vi "UHR-Fleezers Control (host) - 9.5.vi"() -> ()   [LabVIEW 2009]
uses:
  <vilib>/Utility/miscctls.llb/LVPoint32TypeDef.ctl
  <vilib>/Utility/miscctls.llb/LVMinMaxIncTypeDef.ctl
  <vilib>/userDefined/High Color/nirio_resource_hc.ctl
  <vilib>/Instr/_visa.llb/VISA Configure Serial Port (Instr).vi
  <vilib>/Platform/TimedLoop/XDataNode/XDataNode.xnode
  <vilib>/Platform/TimedLoop/XDataNode/loadlvalarms.vi
  <vilib>/Platform/TimedLoop/XDataNode/timing_clust.ctl
  <vilib>/Platform/TimedLoop/XDataNode/nitl_modes.ctl
  <vilib>/Platform/TimedLoop/XDataNode/wakeup.ctl
  <vilib>/rvi/interface/nirviOpenFPGA/nirviOpenFPGA.xnode
  FPGA Bitfiles/UHR-Fleezers Instr~3C_FPGA Target_UHR-Fleezers Contr~A5.lvbitx
  UHR-Fleezers Control (fpga) - 9.4.vi
  <vilib>/FPGAPlugInAG/PCIe-7852R/nirviIntfOpen_PCIe-7852R.vi
  <vilib>/rvi/interface/nirviMethod/nirviMethod.xnode
  <vilib>/Utility/error.llb/Merge Errors.vi
  <vilib>/LabVIEW Targets/FPGA/Rio/nirio_HostInterface/nirio_Reset.vi
  <vilib>/LabVIEW Targets/FPGA/Rio/nirio_HostInterface/nirio_DMAStopAll.vi
  <vilib>/rvi/interface/common/niFpgaNodeNameForErrorReporting.ctl
  <vilib>/rvi/errors/niLvFpgaWhatHappensToTopLevelVI.ctl
  <vilib>/LabVIEW Targets/FPGA/Rio/nirio_HostInterface/nirio_DisableInterrupts.vi
  <vilib>/Utility/error.llb/Error Cluster From Error Code.vi
  <vilib>/rvi/errors/niLvFpgaAdjustHostInterfaceError.vi
  <vilib>/rvi/interface/nirviReadWriteControl/nirviReadWriteControl.xnode
  <vilib>/LabVIEW Targets/FPGA/Rio/nirio_HostInterface/nirio_WriteBig.vi
  <vilib>/LabVIEW Targets/FPGA/Rio/nirio_HostInterface/nirio_DMAConfigure.vi
  <vilib>/LabVIEW Targets/FPGA/Rio/nirio_HostInterface/nirio_DMAStop.vi
  <vilib>/RVI Host/nirviSupport.llb/nirviErrorClusterFromErrorCode.vi
  <vilib>/LabVIEW Targets/FPGA/Rio/nirio_HostInterface/nirio_EnableInterrupts.vi
  <vilib>/rvi/errors/niLvFpgaReportInternalErrorWithAdditionalInfo.vi
  <vilib>/express/express analysis/Spectral/XNode/ExpressSpectralMeasurementsBlockNode.xnode
  <vilib>/express/express analysis/Spectral/Block/exnSpectralBlock spectral measurements PSD poly.vi
  <vilib>/express/express analysis/Spectral/Block/exnSpectralBlock spectral measurements PSD WFM.vi
  <vilib>/Waveform/WDTOps.llb/WDT Append Waveforms DBL.vi
  <vilib>/LabVIEW Targets/FPGA/Rio/nirio_HostInterface/nirio_ReadBig.vi
  <vilib>/rvi/interface/nirviCloseFPGA/nirviCloseFPGA.xnode
  <vilib>/FPGAPlugInAG/PCIe-7852R/nirviIntfClose_PCIe-7852R.vi
  <vilib>/vision/Avi1.llb/AviRefnum.ctl
  <vilib>/Analysis/NI_AALBase.lvlib
  <vilib>/Platform/TimedLoop/XDataNode/XDNodeRunTimeDep.lvlib
  openfpgaref.8.6.ctl
  NiRioSrv.dll
  <vilib>/vision/NI_Vision_Development_Module.lvlib
panel:
  in  "Sample Channel Flow":bool
  in  "Pump 3 contents":string="Left: ADig beads" caption="contents"
  in  "Pump 1 contents":string="Right: DNA beads" caption="contents"
  in  "Scripts":T1(tab)=enum."Fluor. Triggering (Yanking)"
  in  "Cap 1 Samp Flow ON":bool=TRUE
  in  "Cap 2 Samp Flow ON":bool=TRUE
  in  "Got DNA bead":bool
  in  "Got ADig bead":bool
  in  "Cap 2 Flow ON":bool=TRUE
  in  "Cap 1 Flow ON":bool=TRUE
  in  "Cap 2 T ON":bool=TRUE
  in  "Move Cap. 2 (ADig Left)":bool
  in  "Move Cap. 1 (DNA Right)":bool
  in  "Offset @ (MHz)":dbl=13.0
  in  "Cal/Data Acq. Spot":bool
  in  "W/ Offset":bool=TRUE
  in  "Cal @ (MHz)":dbl=15.0
  in  "Dump Beads":bool
  in  "Lower Ch. Cap.":bool
  in  "Cap 1 T ON":bool=TRUE
  in  "Move to Delta 2 (MHz)":dbl=15.0
  in  "Attempt Limit":dbl=30.0 caption="Limit"
  out "Attempts":dbl
  in  "Wait Before Save (s)":u32=1
  in  "Fish for Tether":bool
  in  "Closest Delta (MHz)":dbl=10.45 step=0.25
  in  "Stop F (pN)":dbl=2.0
  in  "Then...":string(combo)="5"
  in  "Move to Delta 1 (MHz)":dbl=13.0
  in  "Tether Alarm?":bool=TRUE
  out "Tether":bool
  in  "TA Cancel Save?":bool
  in  "TA Green Off?":bool
  in  "Dip Trap Delta 1 (MHz)":dbl=15.0
  in  "Move Trap Before?":bool
  in  "Save Data After?":bool
  in  "Green ON After?":bool
  in  "Dip Trap Delta 2 (MHz)":dbl=15.0
  in  "Move Trap After?":bool
  in  "Duration (s)":dbl=1.0
  in  "Dip for Protein":bool
  in  "APD to Watch":bool
  out "Duration (s)":dbl
  in  "Action":string(combo)="Yank"
  in  "Fl. Triggered...":bool
  in  "Fl. Delta Thresh. (kHz)":dbl=0.6
  out "Waiting":bool
  out "Fl. High":bool
  in  "N pts to average":u16=6
  in  "Yank Delay (s)":dbl=3.5
  in  "Yank to Delta Array (MHz)":dbl[](array[numeric])=[16.3, 15.85, 14.85]
  in  "N Array El":u8=3 min=1 step=1
  in  "Random Choice":bool=TRUE
  in  "Force Yank":bool
  in  "Force Reset":bool
  in  "Y change (mm)":dbl
  in  "Profile":bool
  out "Current Position":cluster{dbl, dbl, dbl}
  out "Sigma/Mean 2":dbl caption="Sigma/Mean" format="%#_2g"
  out "Rate sigma (Hz) 2":dbl caption="Sigma (Hz)" format="%0.2f"
  out "APD 2 Rate (Hz)":dbl format="%#_3p"
  out "Primary Video Display":T2(plugin-control)
  out "Waveform Graph":dbl[](graph) caption="APD Line Scan"
  in  "Inject Pump 3":bool
  in  "Inject Pump 1":bool
  out "Messages":string
  in  "APD Ave N":dbl=10.0
  out "Int. Time (s)":dbl
  in  "Stop All":bool
  out "Sigma/Mean":dbl format="%#_2g"
  out "Rate sigma (Hz)":dbl caption="Sigma (Hz)" format="%0.2f"
  in  "Tab Control 6":T3(tab)=enum."Imaging"
  in  "APD 2 Offset":dbl
  in  "APD 1 Offset":dbl
  out "RMS (Ang)":dbl format="%_2g"
  in  "Bead Sep. Int. Time (s)":dbl=5.0 caption="Int. Time (s)"
  in  "Below (kHz)":dbl=0.5
  in  "Above (kHz)":dbl=2.0
  in  "Adjust Scale\nto Mean":bool
  in  "Rescale on Mean":bool
  in  "Offset (nm)":dbl
  out "Mean":dbl caption="Mean (pN)" format="%#_3g"
  out "Force":waveform(dbl)[](graph)
  out "APD Chart":waveform(dbl)[](graph)
  in  "Calibration":u16(ring)=2 items=["None", "Position", "Force"]
  out "T1 X":dbl caption="T1 X (pN)" format="%0.2f"
  out "T2 X":dbl caption="T2 X (pN)" format="%0.2f"
  out "Bead Separation":waveform(dbl)(graph)
  in  "Amplitude (nm)":dbl=1.0
  out "Bead Mean (nm)":dbl caption="Mean (nm)" format="%0.2f"
  out "Difference":dbl caption="Difference (pN)" format="%.2g"
  in  "Take Detection Laser\nImage":bool
  out "APD 2":T2(plugin-control) caption="APD 2 (Cy5)"
  in  "Flip Green Filter":bool
  in  "Set X Only":bool
  in  "Set Y Only":bool
  out "APD 1":T2(plugin-control) caption="APD 1 (Cy3)"
  out "Detection Laser Y":T2(plugin-control)
  out "Pointer Y (V)":dbl format="%_3g"
  out "Pointer X (V)":dbl format="%_3g"
  in  "Set Confocal Spot (X-Y)":bool
  out "Detection Laser X":T2(plugin-control)
  out "Saved APD":dbl[][](graph) caption="Most Recent Time Trace"
  out "Trap Delta Graph":dbl[](graph) caption="Most Recent Time Trace"
  out "Save APD Deriv":dbl[][](graph) caption="Most Recent Time Trace"
  out "Delta Fl. 1":dbl
  out "Delta Fl. 2":dbl
  out "All Signals":waveform(dbl)[](graph)
  in  "Signals to Plot":i32(listbox)
  out "Trap Disp. Freq. (Hz)":dbl caption="Freq. (Hz)" format="%#_6p"
  out "Display Period (s)":dbl caption="Period (s)" format="%#_6p"
  in  "Trap Disp. Downsample":dbl=20000.0 caption="Downsample"
  in  "APD Disp. Scale":dbl=0.1 caption="Scale (Divide,\nfor above plot only)"
  in  "APD Disp. Downsample":dbl=30.0 caption="Integrate" min=1.0 step=1.0
  out "APD Display Freq. (Hz)":dbl caption="Freq. (Hz)"
  out "APD Display Period (s)":dbl caption="Period (s)"
  out "FFT 1":cluster{"f0":dbl, "df":dbl, "magnitude":dbl[]}[](graph)
  out "FFT 2":cluster{"f0":dbl, "df":dbl, "magnitude":dbl[]}[](graph)
  in  "FFT 1 Choice 1":u16(ring) items=["T1 Y", "T1 X", "T1 Sum", "T2 Y", "T2 X", "T2 Sum", "T1 FB X", "T1 FB Sum", "T2 FB X", "T2 FB Sum", "PSD Y", "PSD X", "PSD Y Sum", "none"]
  in  "FFT 2 Choice 1":u16(ring)=13 items=["T1 Y", "T1 X", "T1 Sum", "T2 Y", "T2 X", "T2 Sum", "T1 FB X", "T1 FB Sum", "T2 FB X", "T2 FB Sum", "PSD Y", "PSD X", "PSD Y Sum", "none"]
  in  "FFT 1 Choice 2":u16(ring)=1 items=["T1 Y", "T1 X", "T1 Sum", "T2 Y", "T2 X", "T2 Sum", "T1 FB X", "T1 FB Sum", "T2 FB X", "T2 FB Sum", "PSD Y", "PSD X", "PSD Y Sum", "none"]
  in  "FFT 2 Choice 2":u16(ring)=13 items=["T1 Y", "T1 X", "T1 Sum", "T2 Y", "T2 X", "T2 Sum", "T1 FB X", "T1 FB Sum", "T2 FB X", "T2 FB Sum", "PSD Y", "PSD X", "PSD Y Sum", "none"]
  in  "Compute FFT":bool
  in  "Reset FFT":bool
  in  "# Spectra to Ave.":dbl=100.0
  out "Ave. Time (s)":dbl
  out "1 Channel":waveform(dbl)(graph)
  out "Slow mean":dbl format="%0.2f"
  in  "Slow mean N ave.":dbl=1.0 min=1.0 step=1.0
  out "Mean Intensity":dbl
  out "Sigma":dbl
  out "Sigma/Mean":dbl
  in  "Subtract mean":bool
  in  "High Res. Display":u16(ring) items=["T1 Y", "T1 X", "T1 Sum", "T2 Y", "T2 X", "T2 Sum", "T1 FB X", "T1 FB Sum", "T2 FB X", "T2 FB Sum", "PSD Y", "PSD X", "PSD Y Sum"]
  out "APD 1 Rate (Hz)":dbl format="%#_3p"
  in  "Tab Control":T4(tab)=enum."Configuration"
  out "Stage Moving":bool
  in  "Read Cal":bool
  in  "Confocal Linescan":bool
  in  "Speed (nm/s)":dbl=100.0
  in  "Furthest Withdraw (MHz)":dbl=15.0
  in  "Confocal Image":bool
  in  "Round T1 X":bool caption="Round"
  in  "T1 offset_x (mV)":dbl=-26.302542012392074 format="%#_2g"
  in  "T1 kappa_x (pN/nm)":dbl=0.22546432407642192 min=0.0 step=0.001 format="%#_2g"
  out "Time (s)":dbl
  out "Total Time (s)":dbl
  in  "Start Saving":bool
  in  "Cal sets to save":u32=50 min=1 step=1
  in  "Comment (data description)":string="testing confocal setup"
  out "Calibrating Trap...":bool
  in  "Trap 2 (ON/OFF)":bool
  in  "Trap 1 (ON/OFF)":bool
  in  "Save Calibration":bool
  in  "N sets to save":u32=200 caption="N Sets"
  in  "Save N Sets":bool
  out "Save file name":path
  in  "Save ave N":dbl=500.0 caption="Averaging Factor"
  out "Saving...":bool
  in  "Stop Saving":bool
  out "Progress":u16(slide) scale=0.0..100.0
  out "Manipulating Trap":bool
  out "Buffer Status":dbl(slide) scale=0.0..1.0
  out "Overflow (data lost)":bool
  in  "Reset":bool
  out "Data Rate (Hz)":dbl caption="Trap Data Rate (Hz)" format="%#_3p"
  out "Data Period (s)":dbl caption="Trap Data Period (s)" format="%#_6p"
  out "Save Data Rate (Hz)":dbl caption="Rate (Hz)" format="%#_6p"
  out "Save Data Period (s)":dbl caption="Period (s)" format="%#_6p"
  in  "T1 alpha_x (nm/V)":dbl=630.439304367558 step=10.0 format="%#_3g"
  in  "T2 alpha_x (nm/V)":dbl=704.7738222964198 step=10.0 format="%#_3g"
  in  "T2 kappa_x (pN/nm)":dbl=0.2030110880477556 min=0.0 step=0.001 format="%#_2g"
  in  "T2 offset_x (mV)":dbl=-26.67973517613748 format="%#_2g"
  in  "BD 1 Frequency 1 (MHz)":dbl=70.0000037011009 caption="T1 X (MHz)" min=60.0 max=90.0 step=1.0 format="%#_6p"
  in  "BD 1 Frequency 2 (MHz)":dbl=85.0 caption="T2 X (MHz)" min=60.0 max=90.0 step=1.0 format="%#_6p"
  in  "Green Laser ON/Interlacing":bool
  in  "Round T2 X":bool caption="Round"
  in  "AO1":dbl(slide)=6.408063513378007 caption="Confocal Y (V)" min=0.0 max=10.0 step=0.01 scale=0.0..10.0 scale format="%_1f"
  in  "AO2":dbl(slide)=2.4332770775475328 caption="Confocal X (V)" min=0.0 max=10.0 step=0.01 scale=0.0..10.0 scale format="%_1f"
  in  "Trap Raster Scan":bool
  out "Raster Scanning...":bool
  in  "Trap Delta (MHz)":dbl=14.999996298899106
  in  "Setpoints (V)":cluster{"Set 1":dbl, "Set 2":dbl}={"Set 1"=9.0, "Set 2"=9.0}
  in  "Index":dbl=1.0 caption="Save File Index" min=1.0 step=1.0
  in  "Position Label 5":string="upper flow spot (UvrD)" caption="5"
  in  "Move to Position":bool
  in  "Position":dbl=1.0 min=1.0 max=10.0 step=1.0
  in  "Set Position":bool
  in  "Saved Stage Positions":dbl[][](array[numeric])=[[1.0, 2.24438, -0.22402, 0.00732], [2.0, 0.0, 0.0, 0.0], [3.0, 2.75063, -0.30498, 0.00732], [4.0, 2.75063, -0.30498, 0.00732], [5.0, 2.75063, -2.32612, 0.00732], [6.0, 0.0, 0.0, 0.0], [7.0, 0.0, 0.0, 0.0], [8.0, 0.0, 0.0, 0.0], [9.0, 0.0, 0.0, 0.0], [10.0, 0.0, 0.0, 0.0]]
  in  "Move to Position 5":bool
  in  "z nudge increment (um)":dbl=0.5
  in  "+z":bool
  in  "Position 1 Label":string="Right capillary (DNA beads)" caption="1"
  in  "Set Position 1":bool
  in  "Set Position 2":bool
  in  "Set Position 3":bool
  in  "Set Position 4":bool
  in  "Move to Position 3":bool
  in  "Move to Position 4":bool
  in  "Move to Position 2":bool
  in  "Move to Position 1":bool
  in  "Position 2 Label":string="Left capillary (ADig beads)" caption="2"
  in  "Position 3 Label":string="lower flow spot (ATP)" caption="3"
  in  "Position 4 Label":string="Dump beads" caption="4"
  in  "-z":bool
  in  "Set Position 5":bool
  out "Stage Control Serial Error":errorcluster
  out "Pump 3 cont disp":string="Left: ADig beads"
  out "Pump 1 cont disp":string="Right: DNA beads "
  in  "Ch 1 Inject Rate (ul/h)":dbl=10.0
  in  "Pump write delay (ms)":dbl=300.0
  in  "All Pump Parameters":T5={"Pump 1"={"Diameter (mm)"=4.61, "Units"=3.0, "Volume"=0.0, "Rate"=0.0}, "Pump 2"={"Diameter (mm)"=4.61, "Units"=3.0, "Volume"=0.0, "Rate"=0.0}, "Pump 3"={"Diameter (mm)"=4.61, "Units"=3.0, "Volume"=0.0, "Rate"=0.0}}
  in  "Ch 2 Inject Volume (uL)":dbl=100.0
  in  "Pump pause delay (ms)":u32
  in  "Ch 3 Inject Volume (uL)":dbl=100.0
  in  "Ch 3 Inject Rate (ul/h)":dbl=10.0
  in  "Flush Center Ch Volume (uL)":dbl=15.0
  in  "Flush Center Ch Rate (ul/m)":dbl=100.0
  in  "Inject Pump 2":bool caption="Inject Pump 2\n(Flush Center)"
  in  "Total Volume\nFlushed (uL)":dbl
  in  "Tab Control 2":T6(tab)=enum."AOD Raster Scan"
  out "Total Counts (ticks)":u32
  in  "Trap ON/OFF X or Y Amp?":bool=TRUE
  in  "Oscillate Set 1":bool
  in  "Trap 1 ON":bool
  in  "Number Interlace Sets":u8=3 min=1 max=3
  in  "DIO count 3 (ticks)":u32=200
  in  "DIO count 2 (ticks)":u32=200
  in  "DIO count 1 (ticks)":u32=200
  in  "BD 2 Amplitude 3 (%)":dbl min=0.0 max=50.0 step=1.0
  in  "BD 2 Amplitude 2 (%)":dbl min=0.0 max=50.0 step=1.0
  in  "BD 2 Amplitude 1 (%)":dbl min=0.0 max=50.0 step=1.0
  in  "BD 1 Amplitude 3 (%)":dbl min=0.0 max=50.0 step=1.0
  in  "BD 1 Amplitude 2 (%)":dbl=35.0 min=0.0 max=50.0 step=1.0
  in  "BD 1 Amplitude 1 (%)":dbl=10.0 min=0.0 max=50.0 step=1.0
  in  "BD 2 Frequency 3 (MHz)":dbl=26.0 min=0.0 max=40.0 step=1.0 format="%#_6p"
  in  "BD 1 Frequency 3 (MHz)":dbl=70.0 min=60.0 max=90.0 step=1.0 format="%#_6p"
  in  "BD 2 Frequency 2 (MHz)":dbl=26.0 min=0.0 max=40.0 step=1.0 format="%#_6p"
  in  "BD 2 Frequency 1 (MHz)":dbl=26.0 min=0.0 max=40.0 step=1.0 format="%#_6p"
  in  "Not-Interlacing Set":enum32{"Set 1", "Set 2", "Set 3"}(radio)
  in  "Interlace":bool=TRUE
  in  "Trap 2 ON":bool
  in  "Trap 3 ON":bool
  in  "Scan axis 2":bool=TRUE
  in  "Osc. freq. (Hz)":dbl=0.25
  in  "Osc. amp. (MHz)":dbl=2.0
  out "Coords":T7
  in  "Manipulation Scaling":cluster{"Horizontal":dbl, "Vertical":dbl}={"Horizontal"=0.075, "Vertical"=0.01}
  in  "Freq or Amp switch first":bool=TRUE
  in  "Swap F1 and F2":bool
  in  "Freq switch delay":u16
  in  "Amp switch delay":u16=5
  in  "MCL Step Increment (V_int)":dbl=3.0
  out "Time to Finish All (min)":dbl format="%#_2p"
  in  "Scan Speed (nm/s)":dbl=100.0
  in  "Scan Range (nm)":dbl=500.0
  in  "Step Size (nm)":dbl=1.0
  in  "MCL/AOM Scale Tweak":dbl=1.0
  in  "MCL Step Position Ratio":dbl=0.5
  in  "Move MCL Also?":bool=TRUE
  out "Final sep (nm)":dbl
  out "Initial sep (nm)":dbl
  out "Save index":dbl
  out "Final delta (MHz)":dbl
  out "Initial delta (MHz)":dbl
  out "Final freq. (MHz)":dbl
  out "Initial freq. (MHz)":dbl
  in  "Saved AOD Raster Scan Parameter Sets":T8(array[cluster])=[{"Scan Range AOD (nm) 2"=500.0, "Step Size AOD (nm) 2"=1.0, "Scan Speed AOD (nm/s) 2"=200.0, "Number of scans (AOD) 2"=1, "Label"=""}, {"Scan Range AOD (nm) 2"=1000.0, "Step Size AOD (nm) 2"=1.0, "Scan Speed AOD (nm/s) 2"=200.0, "Number of scans (AOD) 2"=5, "Label"="wide offset scan"}, {"Scan Range AOD (nm) 2"=20.0, "Step Size AOD (nm) 2"=0.68, "Scan Speed AOD (nm/s) 2"=0.68, "Number of scans (AOD) 2"=1, "Label"="2 bp steps"}]
  in  "Load parameters":bool
  out "Scan Range (MHz)":dbl=10.0
  in  "Restart DMA? (AOD)":bool=TRUE caption="Restart DMA?"
  out "Incr. int (AOD)":i64
  out "Time/Scan (s) (AOD)":dbl format="%#_2p"
  out "Data points/scans":dbl
  out "Data points/scan (f/b)":dbl
  in  "Save scans":bool=TRUE
  out "AOD Scan I":u64 caption="Scan I"
  in  "Continuous AOD Scanning":bool caption="Continuous Scanning"
  in  "Abort AOD Scan":bool caption="Abort Scan"
  in  "Scan BD":bool=TRUE
  out "Cycles/step (AOD)":u64=400 format="%.0p"
  in  "Number of F/B Scans (AOD)":u16=1 min=1
  out "Scan steps (AOD)":u64=1000
  out "Scan Increment (MHz)":dbl=0.2
  out "AOD Scanning":bool caption="Scanning"
  in  "Start AOD Scan":bool caption="Start Scan"
  out "N sets should be saved":dbl
  out "Progress 2":u16(slide) caption="Progress" scale=0.0..100.0
  in  "Abort save 2":bool caption="Abort save"
  in  "Trap 1 Bead Size (nm)":dbl=860.0
  in  "Trap 2 Bead Size (nm)":dbl=790.0
  out "MCL Count":dbl
  in  "All FB On/Off":bool=TRUE
  in  "AI2 to Setpoint":cluster{"Set 1":bool, "Set 2":bool}
  out "AI2 (V)":cluster{"Set 1":dbl, "Set 2":dbl}
  in  "Reset Feedback":cluster{"Set 1":bool, "Set 2":bool}
  in  "PID Gains":T9={"Set 1"={"proportional gain (Kc)"=0, "integral gain (Kc*Ts/Ti)"=5, "derivative gain (Kc*Td/Ts)"=0}, "Set 2"={"proportional gain (Kc)"=0, "integral gain (Kc*Ts/Ti)"=5, "derivative gain (Kc*Td/Ts)"=0}}
  in  "Feedback On/Off":cluster{"Set 1":bool, "Set 2":bool}={"Set 1"=TRUE, "Set 2"=TRUE}
  in  "Tab Control 3":enum32{"Timing", "MCL Scan", "Analog Out"}(tab)
  out "APD 2 Gate Late Counter":u32
  out "APD 2 Gate Relative Phase":i16
  in  "Phase Adj. (APD 2 Gate)":i16=20
  in  "Initial Phase Adjustment (APD 2 Gate)":i16=55
  out "APD 1 Gate Late Counter":u32
  in  "- phase (APD 1 Gate)":bool
  in  "+ phase (APD 1 Gate)":bool
  out "APD 1 Gate Relative Phase":i16
  in  "Phase Adj. (APD 1 Gate)":i16=20
  in  "Initial Phase Adjustment (APD 1 Gate)":i16=60
  in  "Save APD Data\nwith Trap Data":bool=TRUE
  out "APD FIFO Elements Remaining":u32
  in  "- phase (APD Acq)":bool
  in  "+ phase (APD Acq)":bool
  out "APD Acq Late Counter":u32
  out "APD Acq Relative Phase":i16
  in  "Phase Adj. (APD Acq)":i16=20
  in  "Initial Phase Adjustment (APD Acq)":i16
  in  "Invert APD Gate":bool caption="Invert Gate"
  in  "APD Gate OFF Count":u32=450 caption="Gate OFF Count"
  in  "APD Gate ON Count":u32=150 caption="Gate ON Count"
  in  "APD Gate":enum32{"ON", "OFF", "Interlace"}(radio)=enum."Interlace"
  in  "APD Integration Time (s)":dbl=0.01 caption="Integration Time (s)"
  out "APD Acq Rate (Hz)":dbl=20000000.0 caption="Rate (Hz)"
  out "APD Samples/FIFO Acq.":dbl
  out "APD Elements/DMA read":u32
  out "APD Int. Count":u32 format="%.0p"
  in  "+ phase (APD 2 Gate)":bool
  in  "- phase (APD 2 Gate)":bool
  in  "Tab Control 5":enum32{"PSD X", "PSD Y", "Other Data Channel"}(tab)
  out "Data map":dbl[][](graph)
  in  "Channel":i32=4
  in  "Abort MCL Scan":bool
  out "MCL Scan I":u64
  out "MCL Scanning":bool
  in  "Start MCL Scan":bool
  out "wait to reset values":bool
  in  "Tab Control 4":enum32{"Scan Settings", "MCL FPGA Loop Timing"}(tab)
  out "Total Time (s)":dbl
  in  "Scan lines (y)":u64=20
  in  "Fast Scan Dir":bool=TRUE
  in  "2D or 1D Scan":bool=TRUE
  out "Initial X":dbl
  out "Initial Y":dbl
  out "Time/f+b scan (s) (MCL)":dbl caption="Time/scan (s)"
  in  "Number of scans (MCL)":u64=1 caption="Scans"
  in  "Scan steps (MCL)":u64=40 caption="Scan steps (x)"
  in  "N APD Samp/step":dbl=3.0
  in  "Scan Range (V)\n(of steps)":dbl=3.5
  in  "Restart DMA? (MCL)":bool=TRUE caption="Restart DMA?"
  in  "Continuous MCL Scanning":bool caption="Cont. Scanning"
  in  "Center Scan":bool=TRUE
  in  "Save Data (MCL)":bool=TRUE caption="Save Data"
  out "Actual Incr. int (MCL)":i16 caption="Incr. int"
  out "Desired incr (int)":dbl
  out "Desired Scan Incr (V)":dbl
  out "N sets should be saved (MCL)":dbl caption="N sets should be saved"
  out "Data points/scans (MCL)":dbl caption="Data points/scans"
  out "Data points/scan (f+b)":dbl caption="points/scan (f+b)"
  out "Cycles/step (MCL)":u64 caption="Cycles/step" format="%.0p"
  out "Actual MCL Inc (V)":dbl
  in  "Phase adjust (MCL)":i16 caption="Phase adjust"
  out "Relative Phase (MCL)":i16 caption="Relative Phase"
  in  "Initial Phase Adj. (MCL)":i16 caption="Initial Phase Adj."
  in  "Update Count (MCL)":u32=600
  in  "+ phase (MCL)":bool
  in  "- phase (MCL)":bool
  out "MCL Late Counter":u32
  in  "APD 1 AO Mult.":i16=1 min=1
  in  "APD 2 AO Mult.":i16=1 min=1
  in  "APD 1 AO offset":i16
  in  "APD 2 AO offset":i16
  in  "Tab Control 7":enum32{"Green FB Signals", "Slow MCL Scan"}(tab)
  out "Green FB Plot":dbl(graph)
  out "MCL Scan 2":cluster{"Begin (V)":dbl, dbl, dbl[]}(graph)
  out "MCL Scan":cluster{"Begin (V)":dbl, dbl, dbl[]}(graph)
  in  "Green laser mode":enum32{"Laser ON", "Laser OFF", "Interlace"}(radio)=enum."Interlace"
  in  "GI Frequency, ON count":u32=150 min=1 step=1
  in  "Invert GI":bool
  out "GI Late Counter":u32
  in  "Phase adj. (GI)":i16=5
  out "GI relative phase":i16
  in  "+ phase (GI)":bool
  in  "Initial Phase Adjustment (GI)":i16=19
  in  "GI Frequency, OFF count":u32=450 min=1 step=1
  in  "- phase (GI)":bool
  out "Green FB Signals (V)":cluster{"Y":dbl, "X":dbl, "Sum":dbl}
  out "Relative phase (Green FB)":i16
  in  "+ phase (Green FB)":bool
  in  "- phase (Green FB)":bool
  in  "Green FB Count":u32=600
  in  "Phase adj. (Green FB)":i16=10
  in  "Initial Phase Adjustment (Green FB)":i16=50
  in  "Green FB On/Off":bool=TRUE
  in  "Current When FB OFF (%)":dbl=87.0 min=0.0 max=100.0 step=1.0
  in  "Green int current ON count adj":u32=150
  in  "Green FB Gains":T10={"proportional gain (Kc)"=10, "integral gain (Kc*Ts/Ti)"=5, "derivative gain (Kc*Td/Ts)"=0}
  in  "Green FB Setpoint (mV)":dbl=100.0
  in  "- phase (GI) 2":bool
  in  "Initial Phase Adjustment (GI) 2":i16=-100
  in  "+ phase (GI) 2":bool
  out "GI relative phase 2":i16
  in  "Phase adj. (GI) 2":i16=20
  out "GI Late Counter 2":u32
  in  "# Samples/trap":dbl=20000.0 format="%#_6p"
  out "Elements/DMA read":u32 format="%.0p"
  out "Ave. Rate (Hz)":dbl format="%#_6p"
  out "FIFO El. Rem.":u32 format="%.0p"
  in  "Phase adj. (AI1)":i16=15
  out "Relative phase (AI1)":i16
  in  "+ phase (AI1)":bool
  in  "- phase (AI1)":bool
  out "Late Counter (AI1)":u32
  in  "Initial Phase Adjustment (AI1)":i16=220
  out "AI rate (Hz)":dbl=50000.0 format="%#_6p"
  in  "AI Count (ticks)":u32=200
  out "# Samples/channel":u32=20000 format="%.0p"
  in  "FIFO Depth":u32=600000 format="%.0p"
  in  "Detector Type":string(combo)="IR-QPD + PSD + FB-QPD X position"
  in  "N Acq Sets (Traps + Fl.)":i16=3
  in  "Sets to FIFO (Traps)":T11={"Set 1"=TRUE, "Set 2"=TRUE, "Set 3"=FALSE}
  in  "FPGA Ave.":dbl=1.0 min=1.0 step=1.0
  out "Ave. Period (s)":dbl format="%#_6p"
  out "DMA Update Period (s)":dbl
  out "FPGA Averaging":bool
  out "Trap Sets":i16
  out "Counts/DMA":dbl format="%#_6p"
  in  "Video Capture Rate (Hz)":dbl=30.0
  in  "Video Index":dbl=1.0 min=1.0 step=1.0
  in  "New Video File":bool
  in  "Save Video":bool
  in  "Reset Averaging":bool
  in  "Averaging":bool
  in  "Save Image":bool
  in  "Image Index":dbl=1.0 min=1.0
  out "Path Out":path
  in  "Center Point":cluster{"X":i32, "Y":i32}={"X"=335, "Y"=271}
  in  "Zoom Factor":sgl=7.0
  out "Window Size":cluster{"Width":i32, "Height":i32}
  out "Window Position":cluster{"X Position":i32, "Y Position":i32}={"X Position"=40, "Y Position"=40}
  in  "Initial Window Size":cluster{"Width":i32, "Height":i32}={"Width"=884, "Height"=619}
  in  "Initial Window Position":cluster{"X Position":i32, "Y Position":i32}={"X Position"=796, "Y Position"=4}
  in  "Intensity Upper":dbl=88.0
  in  "Intensity Lower":dbl=66.0
  out "error out":errorcluster
  out "error out 2":errorcluster
  in  "Harvard Syringe Pump Serial Port":refnum<visa-resource-name>="ASRL5::INSTR"
  in  "Lost Tether Alarm Threshold (pN)":dbl=0.5
  in  "AOM X Cal (nm/MHz)":dbl=123.0
  in  "MCL X Cal (nm/V)":dbl=1070.0
  out "X RF Amplitude Limits (%)":T12={"Minimum"=0.0, "Maximum"=50.0, "Increment"=1.0}
  out "X RF Frequency Limits (MHz)":T12={"Minimum"=60.0, "Maximum"=90.0, "Increment"=1.0}
  out "Y RF Frequency Limits (MHz)":T12={"Minimum"=60.0, "Maximum"=90.0, "Increment"=1.0}
  out "Y RF Amplitude Limits (%)":T12={"Minimum"=0.0, "Maximum"=50.0, "Increment"=1.0}
  in  "Manip. X?":bool=TRUE
  in  "Manip. Y?":bool
  in  "Force Manip Abort":bool
  out "Read cal error":errorcluster
  in  "DAQ Delay (ms)":u32=1000
  in  "Start Scan":bool
  in  "Scan axis":bool=TRUE
  in  "Osc. amp. (V)":dbl=5.0
  in  "Osc. center (V)":dbl=5.0
  in  "Osc. freq. (Hz) 2":dbl=1.0
  in  "MCL Mode":u16(ring) items=["Manual Positioning", "Sinusoidal Wave", "Linear Scan"]
  in  "Begin (V)":dbl
  in  "End (V)":dbl=10.0
  in  "N Points":dbl=20.0
  in  "Delay to Interlace (s)":dbl
  in  "Delayed Interlace Start":bool
  in  "Read Lateness and Rel Phase":bool
  out "Vec Mean of T1 T2":dbl[](array[numeric])
  in  "Cal read wait (s)":u32=5
  out "Time tether formed":timestamp
  in  "Sample Chamber Stage Serial Port":refnum<visa-resource-name>="ASRL4::INSTR"
  in  "Chemyx Syringe Pump Serial Port":refnum<visa-resource-name>="ASRL3::INSTR"
  in  "APD2 Trigger on Edge?":bool=TRUE
  in  "APD1 Trigger on Edge?":bool=TRUE
  in  "Limit Min (MHz)":dbl=10.0 caption="Min (MHz)"
  in  "Limit Max (MHz)":dbl=16.0 caption="Max (MHz)"
  in  "Limits Enable":bool=TRUE caption="Enable"
  # "After"
  # "During"
  # "Trap On?"
  # "BD Flow ON?"
  # "Samp Flow ON?"
  # "1"
  # "2"
  # "Trap Display:"
  # "APD Display:"
  # "DAQ"
  # "Trap Manipulation"
  # "Data Saving"
  # "Bead Calibration"
  # "Harvard Pump\n(sample channel for flow exp)"
  # "Chemyx Pump 2"
  # "Units: \n1 = ml/m\n2 = ml/h\n3 = ul/m\n4 = ul/h"
  # "Rate param is ul/h\nVolume param is ul"
  # "X"
  # "Y"
  # "Oscillate Set 1 freq. (debugging)"
  # "BD 1"
  # "BD 2"
  # "AOD Raster Scan"
  # "Approx. trap separations"
  # "X"
  # "Y"
  # "APD Gates"
  # "APD 2"
  # "APD 1"
  # "X"
  # "2D"
  # "Y"
  # "1D"
  # "Green Laser Interlacing"
  # "Green FB Measurement"
  # "Digital Gate"
  # "Current Analog Control"
  # "Total AI Rates (NOT rates/trap)"
  # "(Samples/trap x Trap Sets)"
  # "(Samples/channel x\n8 if averaging (8 channels)\n4 if no averaging)"
  # "Trap 1"
  # "Trap 2"
  # "Flour./Trap 3"
  # "External Video Window"
  # "MCL Position Debugging"
  # "Temporary Control Storage\n(these used to be somewhere else, still want to keep them)"
  # "Y"
  # "X"
  # "Trap Position Difference Limits"
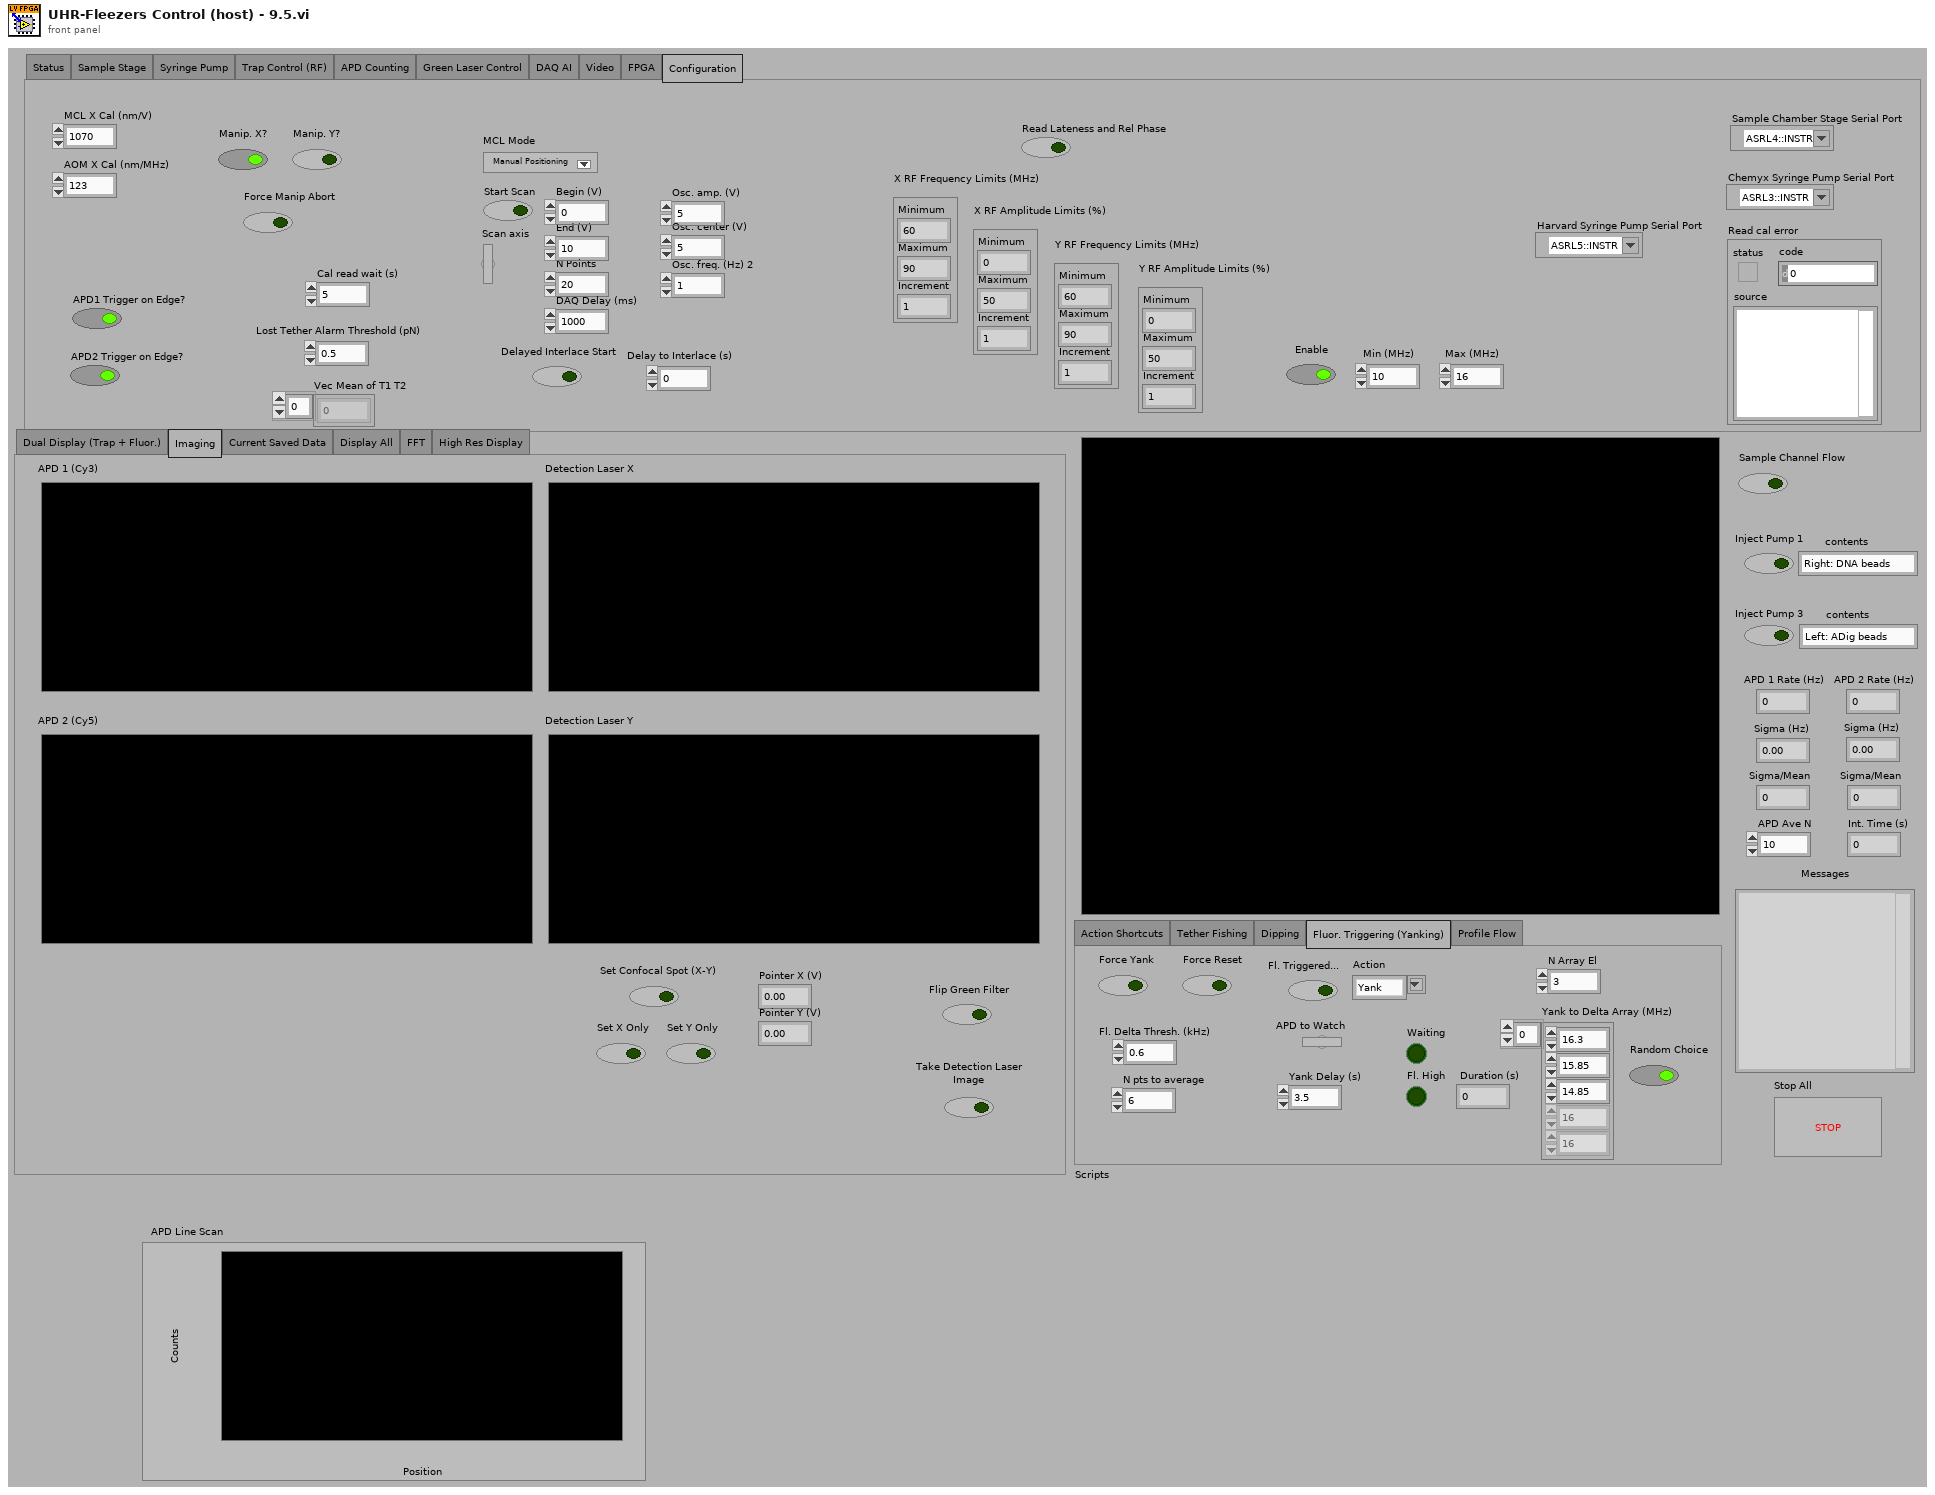
[diagram p1: front panel]
types:
  T1 = enum32{"Action Shortcuts", "Tether Fishing", "Dipping", "Fluor. Triggering (Yanking)", "Profile Flow"}
  T2 = typedef "IMAQ Image.ctl" = refnum<image>
  T3 = enum32{"Dual Display (Trap + Fluor.)", "Imaging", "Current Saved Data", "Display All", "FFT", "High Res Display"}
  T4 = enum32{"Status", "Sample Stage", "Syringe Pump", "Trap Control (RF)", "APD Counting", "Green Laser Control", "DAQ AI", "Video", "FPGA", "Configuration"}
  T5 = cluster{"Pump 1":cluster{"Diameter (mm)":dbl, "Units":dbl, "Volume":dbl, "Rate":dbl}, "Pump 2":cluster{"Diameter (mm)":dbl, "Units":dbl, "Volume":dbl, "Rate":dbl}, "Pump 3":cluster{"Diameter (mm)":dbl, "Units":dbl, "Volume":dbl, "Rate":dbl}}
  T6 = enum32{"IR Laser Interlacing (Direct RF Board Control Method)", "AOD Raster Scan", "Feedback on BD 1 Amp to Control AI2"}
  T7 = typedef "LVPoint32TypeDef.ctl" = cluster{"Horizontal":i32, "Vertical":i32}
  T8 = cluster{"Scan Range AOD (nm) 2":dbl, "Step Size AOD (nm) 2":dbl, "Scan Speed AOD (nm/s) 2":dbl, "Number of scans (AOD) 2":u16, "Label":string}[]
  T9 = cluster{"Set 1":cluster{"proportional gain (Kc)":i16, "integral gain (Kc*Ts/Ti)":i16, "derivative gain (Kc*Td/Ts)":i16}, "Set 2":cluster{"proportional gain (Kc)":i16, "integral gain (Kc*Ts/Ti)":i16, "derivative gain (Kc*Td/Ts)":i16}}
  T10 = cluster{"proportional gain (Kc)":i16, "integral gain (Kc*Ts/Ti)":i16, "derivative gain (Kc*Td/Ts)":i16}
  T11 = cluster{"Set 1":bool, "Set 2":bool, "Set 3":bool}
  T12 = typedef "LVMinMaxIncTypeDef.ctl" = cluster{"Minimum":dbl, "Maximum":dbl, "Increment":dbl}
  T13 = typedef "Image Type" = u32
  T14 = typedef "nirio_resource_hc.ctl" = tag
  T15 = typedef "openfpgaref.8.6.ctl" = refnum<k20>
  T16 = typedef "niFpgaNodeNameForErrorReporting.ctl" = enum16{"Open FPGA VI Reference", "Read/Write Control", "Invoke Method: Abort", "Invoke Method: Acknowledge IRQ", "Invoke Method: Download", "Invoke Method: FIFO.Configure", "Invoke Method: FIFO.Read", "Invoke Method: FIFO.Start", "Invoke Method: FIFO.Stop", "Invoke Method: FIFO.Write", "Invoke Method: Reset", "Invoke Method: Run", "Invoke Method: Wait on IRQ", "Close FPGA VI Reference"}
  T17 = typedef "niLvFpgaWhatHappensToTopLevelVI.ctl" = enum16{"top level VI scripted behind XNode", "top level VI inlined behind XNode"}
  T18 = cluster{"New Image":T2, "New Image":T2, "New Image":T2, "New Image":T2}
  T19 = typedef "XDNodeRunTimeDep.lvlib/timing_clust.ctl" = cluster{"Expected End [f-1]":u64, "Actual End [f-1]":u64, "Finished Late? [f-1]":bool, "Expected End [i-1]":u64, "Actual End [i-1]":u64, "Finished Late? [i-1]":bool, "Expected Start [i]":u64, "Actual Start [i]":u64, "Expected Start [f]":u64, "Actual Start [f]":u64, "Source Name":string, "Structure Name":string, "Period":i64, "Deadline":i64, "Offset":i64, "Start":i64, "Priority":i32, "Timeout":i32, "Mode":T20, "Wakeup Reason":T21, "Error":errorcluster, "Source Type":string, "Secondary Source Type":string, "Global End Time":u64, "Global Start Time":u64, "Frame Duration":u64, "Iteration Duration":u64, "Assigned CPU":i32, "I/O Scan Engine Mode":u32}
  T20 = typedef "XDNodeRunTimeDep.lvlib/nitl_modes.ctl" = enum32{"No Change", "Process missed periods, maintain original phase", "Discard missed periods, maintain original phase", "Process missed periods, ignore original phase", "Discard missed periods, ignore original phase"}
  T21 = typedef "XDNodeRunTimeDep.lvlib/wakeup.ctl" = enum32{"Normal", "Aborted", "Asynchronous wakeup", "Timing source error", "Timed loop error", "Timeout"}
  T22 = enum32{"Normal Display", "Dual Display (APD)", "FFT", "High Res Display"}
  T23 = cluster{"Origin Pixel":cluster{"X":sgl, "Y":sgl}, "Angle Relative to Horizontal (deg)":sgl, "Axis Reference":u32}
  T24 = typedef "Simple Grid Descriptor" = cluster{"X Step":sgl, "Y Step":sgl, "Unit":T25}
  T25 = typedef "Image Unit" = enum32{"Undefined", "Angström", "Micrometer", "Millimeter", "Centimeter", "Meter", "Kilometer", "Microinch", "Inch", "Feet", "Nautical miles", "Standard miles", "Steps"}
  T26 = cluster{"averaging mode":u16, "weighting mode":u16, "number of averages":u32}
  T27 = cluster{"dB On (F)":bool, "unwrap phase (F)":bool, "convert to degree (F)":bool}
  T28 = cluster{"Green FB Ch 0":i16, "Green FB Ch 1":i16, "Green FB Ch 2":i16}
  T29 = enum16{"open", "replace", "create", "open or create", "replace or create", "replace or create with confirmation"}
  T30 = enum16{"big-endian, network order", "native, host order", "little-endian"}
  T31 = cluster{string, string, string, string, string, string, string, string}
  T32 = cluster{string, string, string, string, string, string, string, string, string, string, string, string}
  T33 = cluster{string, string, string, string, string, string, string, string, string, string, string, string, string}
  T34 = cluster{string, string, string, string, string, string, string, string, string, string, string, string, string, string}
  T35 = cluster{"f0":dbl, "df":dbl, "magnitude":dbl[]}[][]
  T36 = cluster{"Green FB Ch 0":dbl, "Green FB Ch 1":dbl, "Green FB Ch 2":dbl}
  T37 = enum32{"setting", "request", "request control", "info", "statistics", "system settings", "I/O sub system", "HRT control", "camera descriptions", "device specific data", "event sub system settings", "event sub system results", "image memory manager"}
  T38 = typedef "AviRefnum.ctl" = refnum<k1>
  T39 = typedef "imagedata.ctl" = cluster{"image type":i32, "image depth":i32, "image":u8[], "mask":u8[], "colors":u32[], "Rectangle":cluster{"left":i16, "top":i16, "right":i16, "bottom":i16}}
  T40 = cluster{"Scan Range AOD (nm) 2":dbl, "Step Size AOD (nm) 2":dbl, "Scan Speed AOD (nm/s) 2":dbl, "Number of scans (AOD) 2":u16, "Label":string}
  T41 = cluster{"[0]":dbl, "[1]":dbl, "[2]":dbl, "[3]":dbl, "[4]":dbl, "[5]":dbl}
  T42 = cluster{"Diameter (mm)":dbl, "Units":dbl, "Volume":dbl, "Rate":dbl}
  T43 = cluster{"Left":i32, "Top":i32, "Width":u32, "Height":u32}
  T44 = cluster{cluster{"Left":i32, "Top":i32, "Width":u32, "Height":u32}}[]
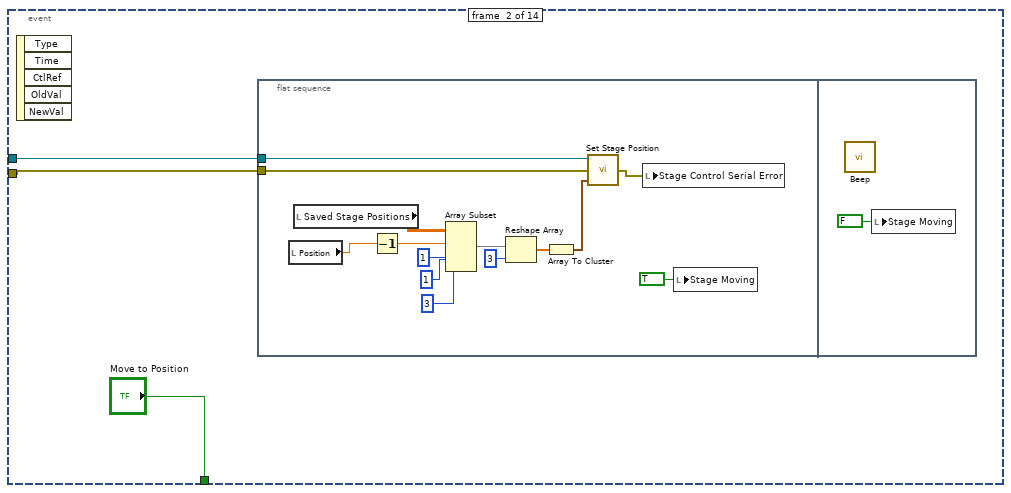
[diagram p2: hidden frame]
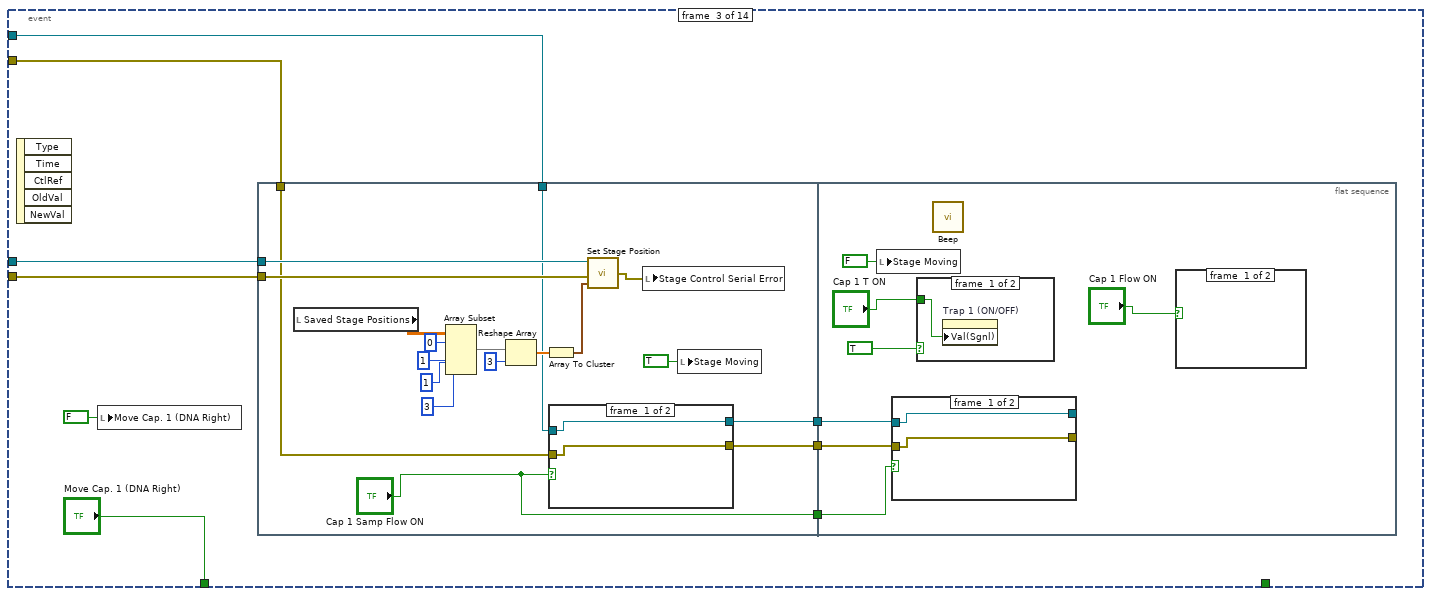
[diagram p3: hidden frame]
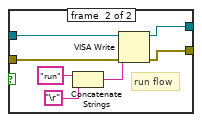
[diagram p4: hidden frame]
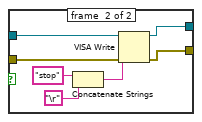
[diagram p5: hidden frame]
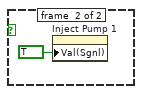
[diagram p6: hidden frame]
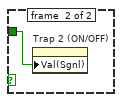
[diagram p7: hidden frame]
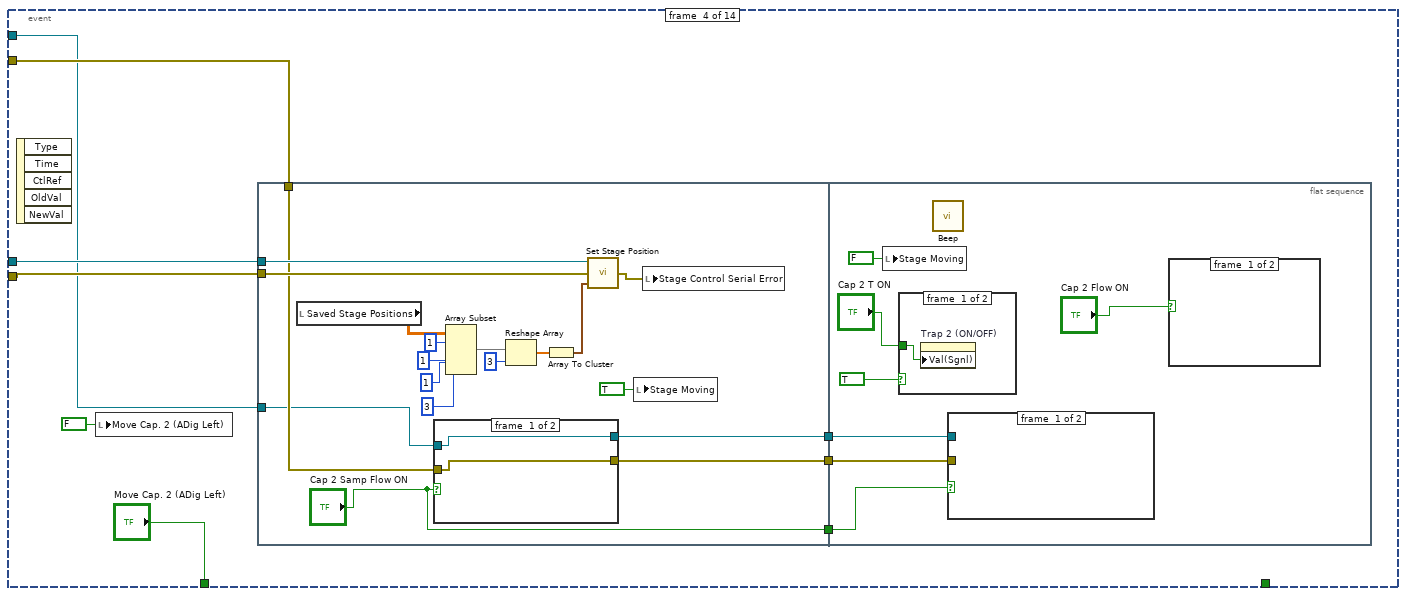
[diagram p8: hidden frame]
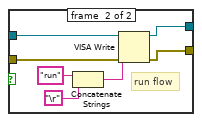
[diagram p9: hidden frame]
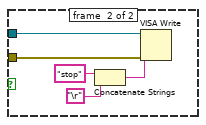
[diagram p10: hidden frame]
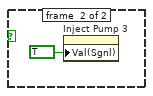
[diagram p11: hidden frame]
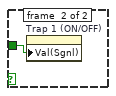
[diagram p12: hidden frame]
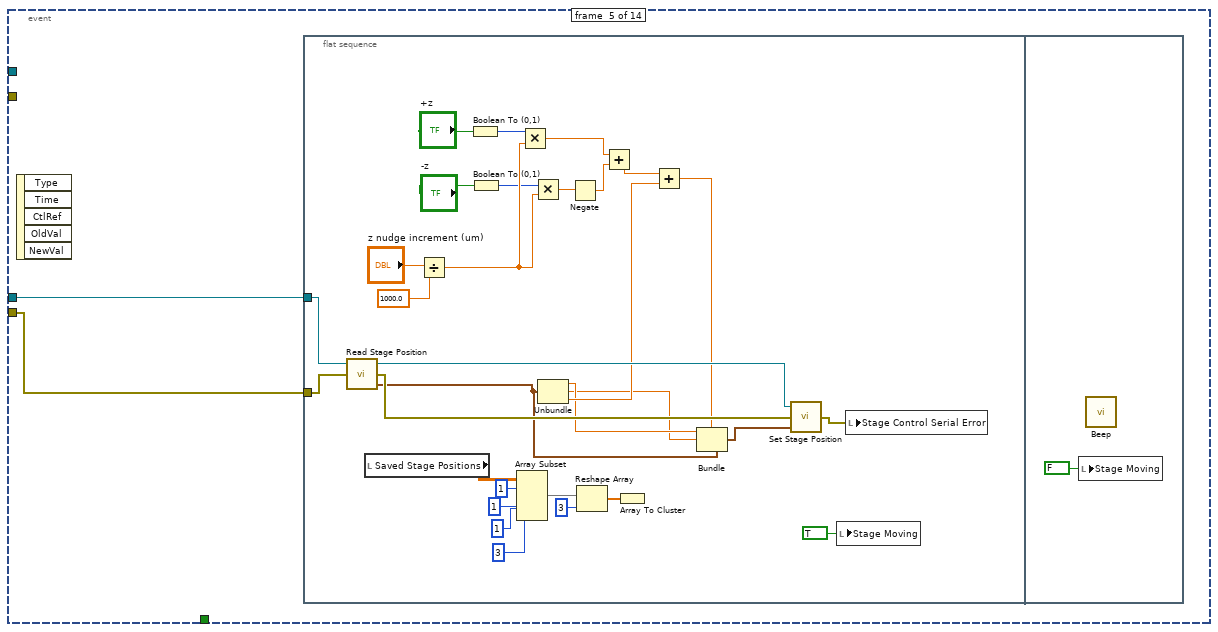
[diagram p13: hidden frame]
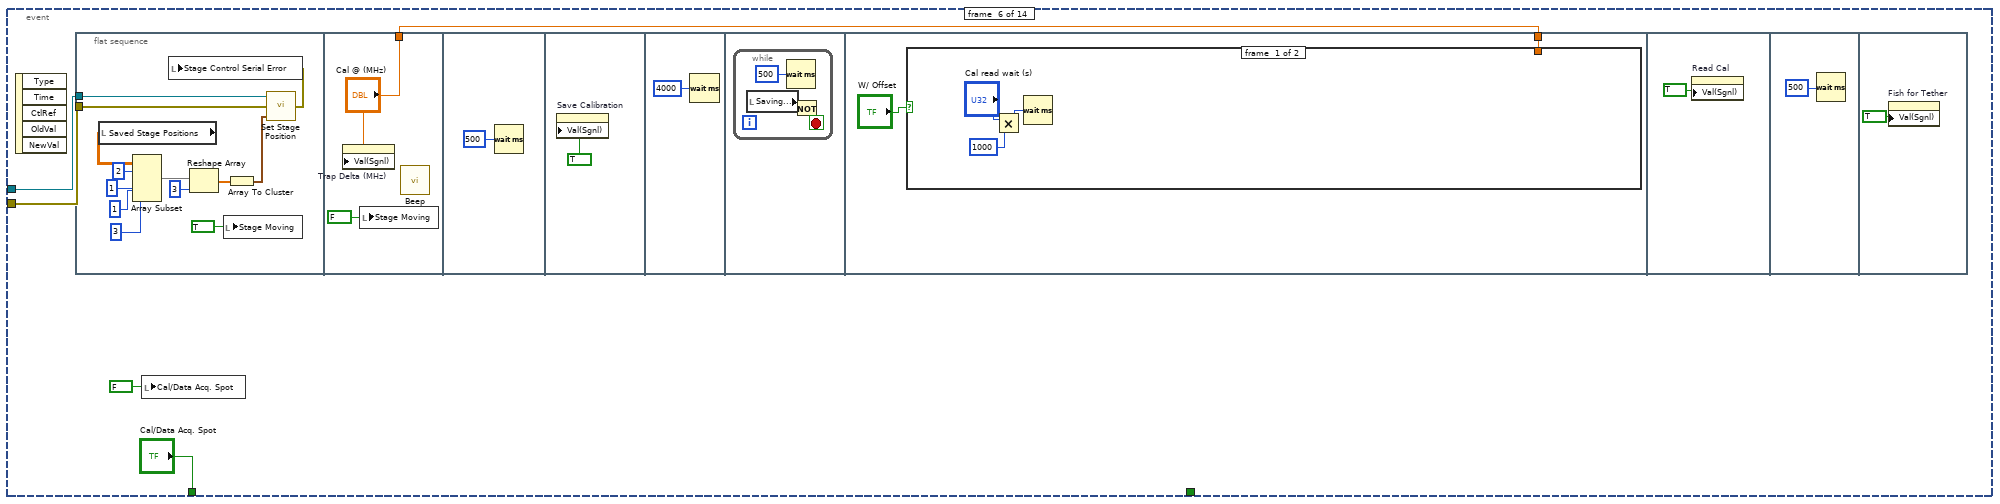
[diagram p14: hidden frame]
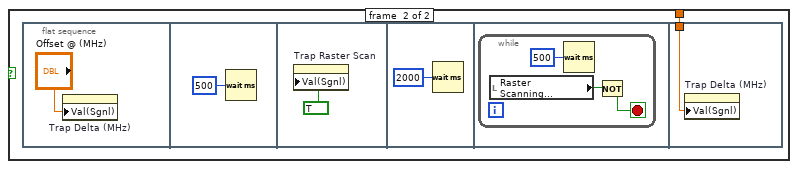
[diagram p15: hidden frame]
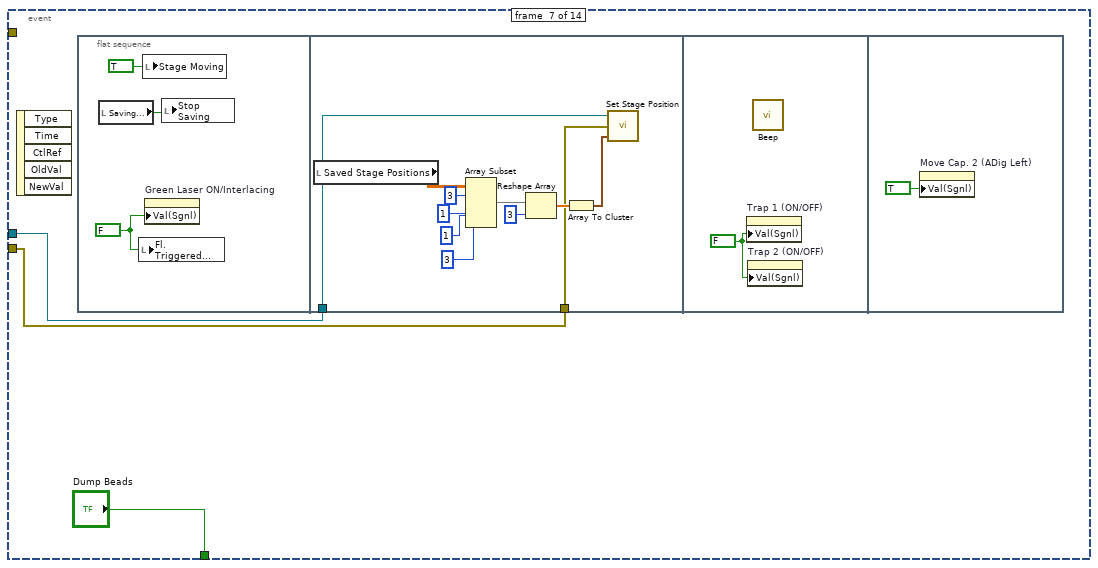
[diagram p16: hidden frame]
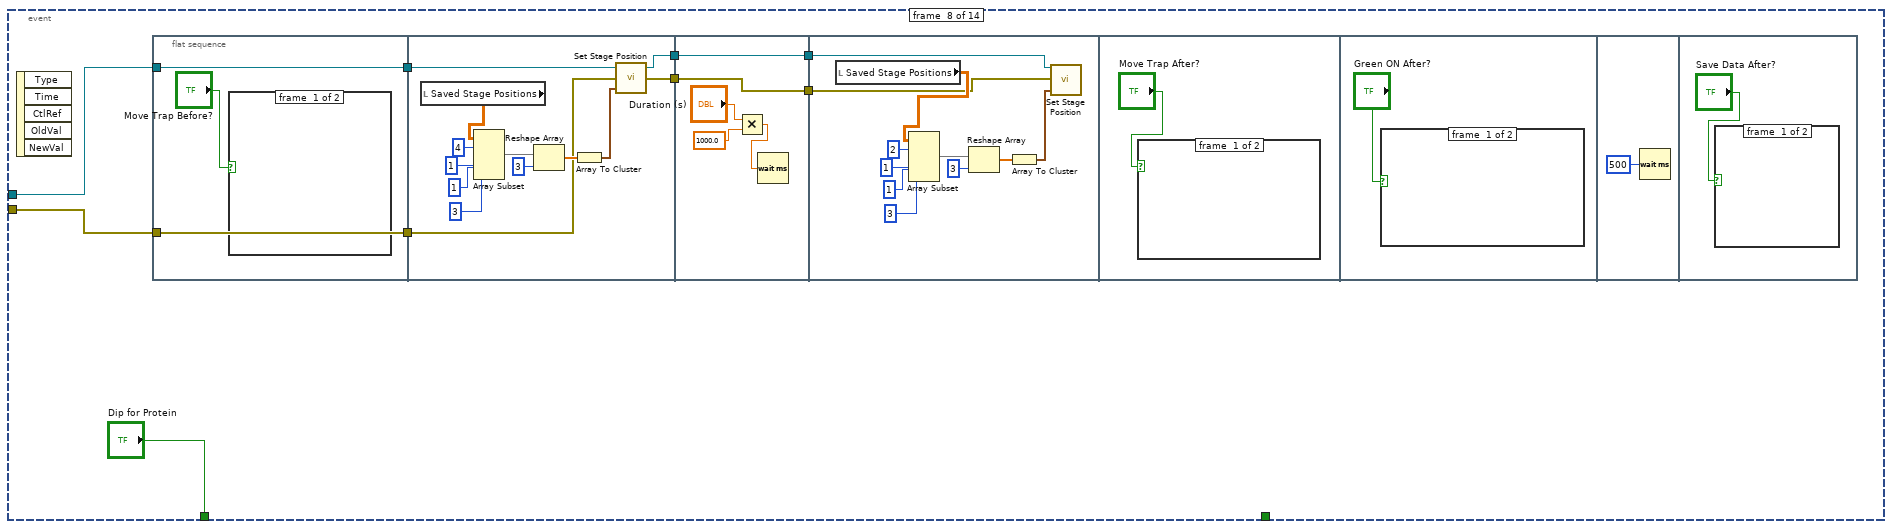
[diagram p17: hidden frame]
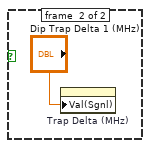
[diagram p18: hidden frame]
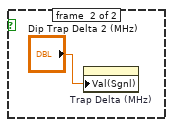
[diagram p19: hidden frame]
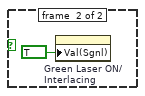
[diagram p20: hidden frame]
diagram:
  w4 = u16 20 items=["1.0"=10, "1.5"=15, "2.0"=20] ("stop bits (10: 1 bit)")
  w11 = T13 2 items=["Grayscale (U8)", "Grayscale (I16)", "Grayscale (SGL)", "Complex (CSG)", "RGB (U32)", "HSL (U32)", "RGB (U64)", "Grayscale (U16)"] ("Image Type")
  w81 = cluster{"output high":i16, "output low":i16} {"output high"=3000, "output low"=0} ("FB output range 1")
  w87 = TRUE ("AI to FIFO")
  w172 = 10.0 ("y")
  w171 = 32767.0 ("y")
  w187 = 6.0  # clock mult.
  w188 = 49152000.0  # TCXO frequ.
  n1 = Build Array("DIO count 1 (ticks)", "DIO count 2 (ticks)", "DIO count 3 (ticks)") -> (w68:u32[])
  n2 = Multiply(x="APD Integration Time (s)", y=40000000.0) -> (x*y=w95:dbl)
  n3 = Reciprocal(x="APD Integration Time (s)") -> (1/x=w92:dbl)
  n4 = local write "APD Acq Rate (Hz)"(w92) -> ()
  n5 = local read "AO1"() -> (w166:dbl)
  n6 = local read "AO2"() -> (w165:dbl)
  n7 = To Unsigned Long Integer(number=w95) -> (unsigned 32bit integer=w94:u32)
  "APD Int. Count" <- w94
  n8 = local read "Scan Increment (MHz)"() -> (w183:dbl)
  n9 = local read "Continuous MCL Scanning"() -> (w153:bool)
  n10 = local read "Fast Scan Dir"() -> (w152:bool)
  n11 = Multiply(x=w166, y=w171) -> (x*y=w168:dbl)
  n12 = local read "Number of scans (MCL)"() -> (w154:u64)
  n13 = Multiply(x=w165, y=w171) -> (x*y=w170:dbl)
  n14 = Divide(x=w168, y=w172) -> (x/y=w167:dbl)
  n15 = Divide(x=w170, y=w172) -> (x/y=w169:dbl)
  n16 = To Word Integer(number=w167) -> (16bit integer=w164:i16)
  n17 = To Word Integer(number=w169) -> (16bit integer=w163:i16)
  n18 = Not(x=w152) -> (.not. x?=w147:bool)
  n19 = local read "Cycles/step (MCL)"() -> (w155:u64)
  n20 = Multiply(x=w183, y=1000.0) -> (x*y=w190:dbl)
  n21 = local read "Scan steps (MCL)"() -> (w156:u64)
  n22 = local read "Desired Scan Incr (V)"() -> (w158:dbl)
  n23 = Scale By Power Of 2(n=48, x=w190) -> (x*2^n=w191:dbl)
  n24 = Multiply(x=w188, y=w187) -> (x*y=w186:dbl)
  n25 = Divide(x=w191, y=w186) -> (x/y=w185:dbl)
  n26 = local read "Setpoints (V)"() -> (w208:cluster{"Set 1":dbl, "Set 2":dbl})
  n27 = property on="AI Count (ticks)" class="DigNum (strict)"("Val(Sgnl)"="AI Count (ticks)") -> ()  [unwired: 2 in, 2 out]
  n28 = local read "Number Interlace Sets"() -> (w61:u8)
  n29 = Split 1D Array(array=w68, index=w61) -> (first subarray=w70:u32[])  [unwired: 1 out]
  n30 = Add Array Elements(numeric array=w70) -> (sum=w69:u32)
  n31 = local read "# Samples/channel"() -> (w175:u32)
  n32 = To Quad Integer(1:w185) -> (0:w182:i64)
  n33 = local read "Sets to FIFO (Traps)"() -> (w215:T11)
  n34 = local read "Number of F/B Scans (AOD)"() -> (w176:u16)
  n35 = local read "Not-Interlacing Set"() -> (w60:enum32{"Set 1", "Set 2", "Set 3"})
  n36 = To Unsigned Byte Integer(number=w60) -> (unsigned 8bit integer=w66:u8)
  n37 = Index Array(array=w68, index=w66) -> (element=w67:u32)
  n38 = Divide(x=40000000.0, y="AI Count (ticks)") -> (x/y=w143:dbl)
  n39 = Multiply(x=w158, y=32767.0) -> (x*y=w160:dbl)
  n40 = local read "Feedback On/Off"() -> (w211:cluster{"Set 1":bool, "Set 2":bool})
  n41 = local read "PID Gains"() -> (w203:T9)
  n42 = local read "Scan steps (AOD)"() -> (w181:u64)
  n43 = local read "All FB On/Off"() -> (w212:bool)
  n44 = local read "Cycles/step (AOD)"() -> (w180:u64)
  n45 = local write "AI rate (Hz)"(w143) -> ()
  n46 = Divide(x=w160, y=10.0) -> (x/y=w159:dbl)
  n47 = Multiply(x=w181, y=w180) -> (x*y=w179:u64)
  n48 = Multiply(x=3276.7, y=w208) -> (x*y=w207:cluster{"Set 1":dbl, "Set 2":dbl})
  n49 = To Word Integer(number=w159) -> (16bit integer=w157:i16)
  n50 = Multiply(x=w179, y=u64 2) -> (x*y=w177:u64)
  n51 = Divide(x=w143, y="FPGA Ave.") -> (x/y=w144:dbl)
  n52 = To Word Integer(number=w207) -> (16bit integer=w206:cluster{"Set 1":i16, "Set 2":i16})
  n53 = xnode "Open FPGA VI Reference"("resource name"=T14 "750kHzDAQ") -> ("FPGA VI Reference Out"=w198:T15, "error out"=w197:errorcluster)  [unwired: 1 in]
  n54 = Unbundle By Name(w203) -> ("Set 1"=w202:T10, "Set 2"=w201:T10)
  n55 = Multiply(x=w177, y=w176) -> (x*y=w174:u64)
  n56 = Divide(x=w174, y=w175) -> (x/y=w173:dbl)
  n57 = local write "Ave. Rate (Hz)"(w144) -> ()
  n58 = Unbundle By Name(w206) -> ("Set 1"=w205:i16, "Set 2"=w204:i16)
  n59 = local read "2D or 1D Scan"() -> (w84:bool)
  n60 = local write "Data points/scans"(w174) -> ()
  n61 = And(x=w211, y=w212) -> (x .and. y?=w210:cluster{"Set 1":bool, "Set 2":bool})
  n62 = local read "Scan BD"() -> (w192:bool)
  n63 = Reciprocal(x=w144) -> (1/x=w145:dbl)
  n64 = local write "Data points/scan (f/b)"(w177) -> ()
  n65 = local read "N Acq Sets (Traps + Fl.)"() -> (w136:i16)
  n66 = local write "N sets should be saved"(w173) -> ()
  n67 = Unbundle By Name(w210) -> ("Set 1"=w214:bool, "Set 2"=w213:bool)
  n68 = xnode "Invoke Method"("FPGA VI Reference In"=w198, "error in"=w197) -> ("FPGA VI Reference Out"=w80:T15, "error out"=w110:errorcluster)
  n69 = local read "Interlace"() -> (w62:bool)
  n70 = Select(t=w69, s=w62, f=w67) -> (s? t:f=w59:u32)
  n71 = local write "Update Count (MCL)"(w59) -> ()
  n72 = local write "Total Counts (ticks)"(w59) -> ()
  n73 = local write "Ave. Period (s)"(w145) -> ()
  n74 = property on="2D or 1D Scan" class="Bool (strict)"("Val(Sgnl)"=w84) -> ()  [unwired: 2 in, 2 out]
  n75 = xnode "Read/Write Control"("FPGA VI Reference In"=w79, "error in"=w110, "ai count"="AI Count (ticks)", "AI Averages"="FPGA Ave.", "DMA buffer timeout"=0, "AI to FIFO"=FALSE, "Interlace ON/OFF"=w62, "Number Interlace Cycles"=w61, "AI1 Sets to FIFO"=w215, "FB On/Off Set 1"=w214, "FB On/Off Set 2"=w213, "Interlace Off Parameters"=w60, "FB Setpoint Set 1"=w205, "FB Setpoint Set 2"=w204, "FB Gains Set 1"=w202, "FB Gains Set 2"=w201, "FB output range 1"=w81, "FB output range 2"=w81, "Cycles per step"=w180, "Scan BD"=w192, "Number of scans"=w176, "Scan steps"=w181, "Scan freq.  increment"=w182, "AO1"=w164, "AO2"=w163, "Scan freq.  increment (MCL)"=w157, "Scan steps (MCL)"=w156, "Cycles per step (MCL)"=w155, "Number of scans (MCL)"=w154, "MCL count"=w59, "Cont. Scan (MCL)"=w153, "MCL Scan Axis"=w147, "1D or 2D Scan?"=w84, "N of AI1 Int Acq Sets"=w136, "Freq or Amp switch first"="Freq or Amp switch first", "Freq switch delay"="Freq switch delay", "Amp switch delay"="Amp switch delay", "Swap F1 and F2"="Swap F1 and F2", "APD Acq Rate Count"=w94, "APD to FIFO"=FALSE, "APD Gate Operating Mode"="APD Gate", "APD Gate ON Count"="APD Gate ON Count", "APD Gate OFF Count"="APD Gate OFF Count", "Invert APD Gate"="Invert APD Gate", "DIO count 1 (ticks)"="DIO count 1 (ticks)", "DIO count 2 (ticks)"="DIO count 2 (ticks)", "DIO count 3 (ticks)"="DIO count 3 (ticks)", "APD 1 AO scale factor"="APD 1 AO Mult.", "APD 2 AO scale factor"="APD 2 AO Mult.", "APD 1 AO offset"="APD 1 AO offset", "APD 2 AO offset"="APD 2 AO offset") -> ("FPGA VI Reference Out"=w54:T15, "error out"=w56:errorcluster)
  n76 = local read "Green Laser ON/Interlacing"() -> (w57:bool)
  n77 = local read "GI Frequency, OFF count"() -> (w50:u32)
  n78 = local read "GI Frequency, ON count"() -> (w49:u32)
  n79 = Multiply(x="Current When FB OFF (%)", y=655.35) -> (x*y=w40:dbl)
  n80 = local read "Green laser mode"() -> (w58:enum32{"Laser ON", "Laser OFF", "Interlace"})
  n81 = local read "Green FB Count"() -> (w48:u32)
  n82 = To Unsigned Word Integer(number=w40) -> (unsigned 16bit integer=w38:u16)
  n83 = local read "Invert GI"() -> (w52:bool)
  n84 = Multiply(x="Green FB Setpoint (mV)", y=3.2767) -> (x*y=w37:dbl)
  n85 = case shown="False" w57 {
    tunnel: w58 -> [_ w242]
    tunnel: [enum32{"Laser ON", "Laser OFF", "Interlace"}."Laser OFF" ("Green laser mode") w242] -> w51
    frame #0 {
    }
    frame #1 {
    }
  }
  n86 = To Word Integer(number=w37) -> (16bit integer=w35:i16)
  n87 = xnode "Read/Write Control"("FPGA VI Reference In"=w54, "error in"=w56, "Green interlace ON count 2"=w49, "Green interlace OFF count 2"=w50, "Invert GI 2"=w52, "Operating Mode 2"=w51, "Green FB Gains"="Green FB Gains", "Green FB Setpoint"=w35, "Green FB On/Off"="Green FB On/Off", "Current Out"=w38, "Green int current ON count adj"="Green int current ON count adj", "Green FB Count"=w48, "Operating Mode"=w51, "Green interlace OFF count"=w50, "Green interlace ON count"=w49, "Invert GI"=w52, "APD2 Trigger on Edge?"="APD2 Trigger on Edge?", "APD1 Trigger on Edge?"="APD1 Trigger on Edge?") -> ("FPGA VI Reference Out"=w53:T15, "error out"=w55:errorcluster)
  n88 = flat-sequence {
    tunnel: w80 -> [w247]
    tunnel: [w247] -> w79
    tunnel: [w246] -> w78
    tunnel: [w245] -> w77
    tunnel: [w243] -> w75
    tunnel: [w244] -> w76
    frame #0 {
      w244 = T12 {"Minimum"=0.0, "Maximum"=40.0, "Increment"=1.0} ("Min Max Inc")
      w243 = T12 {"Minimum"=0.0, "Maximum"=50.0, "Increment"=1.0} ("Data Entry Limits")
      w246 = T12 {"Minimum"=60.0, "Maximum"=90.0, "Increment"=1.0} ("Min Max Inc")
      w245 = T12 {"Minimum"=0.0, "Maximum"=50.0, "Increment"=1.0} ("Data Entry Limits")
      n89 = property on="BD 2 Frequency 1 (MHz)" class="DigNum (strict)"("Data Range"=w244) -> ()  [unwired: 2 in, 2 out]
      n90 = property on="BD 2 Frequency 3 (MHz)" class="DigNum (strict)"("Data Range"=w244) -> ()  [unwired: 2 in, 2 out]
      n91 = property on="BD 2 Frequency 2 (MHz)" class="DigNum (strict)"("Data Range"=w244) -> ()  [unwired: 2 in, 2 out]
      n92 = property on="BD 1 Frequency 1 (MHz)" class="DigNum (strict)"("Data Range"=w246) -> ()  [unwired: 2 in, 2 out]
      n93 = property on="BD 1 Frequency 2 (MHz)" class="DigNum (strict)"("Data Range"=w246) -> ()  [unwired: 2 in, 2 out]
      n94 = property on="BD 1 Frequency 3 (MHz)" class="DigNum (strict)"("Data Range"=w246) -> ()  [unwired: 2 in, 2 out]
      n95 = property on="BD 2 Amplitude 1 (%)" class="DigNum (strict)"("Data Range"=w243) -> ()  [unwired: 2 in, 2 out]
      n96 = property on="BD 2 Amplitude 2 (%)" class="DigNum (strict)"("Data Range"=w243) -> ()  [unwired: 2 in, 2 out]
      n97 = property on="BD 2 Amplitude 3 (%)" class="DigNum (strict)"("Data Range"=w243) -> ()  [unwired: 2 in, 2 out]
      n98 = property on="BD 1 Amplitude 3 (%)" class="DigNum (strict)"("Data Range"=w245) -> ()  [unwired: 2 in, 2 out]
      n99 = property on="BD 1 Amplitude 2 (%)" class="DigNum (strict)"("Data Range"=w245) -> ()  [unwired: 2 in, 2 out]
      n100 = property on="BD 1 Amplitude 1 (%)" class="DigNum (strict)"("Data Range"=w245) -> ()  [unwired: 2 in, 2 out]
      "X RF Frequency Limits (MHz)" <- w246
      "X RF Amplitude Limits (%)" <- w245
      "Y RF Amplitude Limits (%)" <- w243
      "Y RF Frequency Limits (MHz)" <- w244
    }
  }
  n101 = xnode "Invoke Method"("FPGA VI Reference In"=w53, "error in"=w55, "Depth"="FIFO Depth") -> ("FPGA VI Reference Out"=w200:T15, "error out"=w199:errorcluster)
  n102 = xnode "Invoke Method"("FPGA VI Reference In"=w200, "error in"=w199) -> ("FPGA VI Reference Out"=w109:T15, "error out"=w108:errorcluster)
  n103 = xnode "Invoke Method"("FPGA VI Reference In"=w109, "error in"=w108) -> ("FPGA VI Reference Out"=w107:T15, "error out"=w106:errorcluster)  [unwired: 1 out]
  n104 = flat-sequence "Initial FPGA Loop Relative Phase Adjustment" {
    tunnel: "Initial Phase Adjustment (AI1)" -> [w258]
    tunnel: "Initial Phase Adjustment (GI)" -> [w257]
    tunnel: w107 -> [w256]
    tunnel: w106 -> [w255]
    tunnel: "Initial Phase Adj. (MCL)" -> [w254]
    tunnel: [w259] -> w118
    tunnel: [w253] -> w114
    tunnel: "Initial Phase Adjustment (APD Acq)" -> [w252]
    tunnel: "Initial Phase Adjustment (APD 1 Gate)" -> [w251]
    tunnel: "Initial Phase Adjustment (Green FB)" -> [w250]
    tunnel: "Initial Phase Adjustment (GI) 2" -> [w249]
    tunnel: "Initial Phase Adjustment (APD 2 Gate)" -> [w248]
    tunnel: w118 -> [w430]
    tunnel: [w431] -> w115
    tunnel: w114 -> [w431]
    tunnel: [w430] -> w113
    tunnel: w115 -> [w434]
    tunnel: w113 -> [w433]
    tunnel: [w436] -> w112
    tunnel: [w435] -> w111
    tunnel: [w615] -> w116
    tunnel: [w616] -> w117
    tunnel: w112 -> [w616]
    tunnel: w111 -> [w615]
    frame #0 {
      n105 = xnode "Read/Write Control"("FPGA VI Reference In"=w256, "error in"=w255, "Phase count adjustment"=w258, "Phase count adjustment (GI)"=w257, "Phase count adjustment (MCL)"=w254, "Phase Count Adjustment (APD Acq)"=w252, "Phase count adjustment (APD 1 Gate)"=w251, "Phase count adjustment (APD 2 Gate)"=w248, "Phase count adjustment (Green FB)"=w250, "Phase count adjustment (GI) 2"=w249) -> ("FPGA VI Reference Out"=w253:T15, "error out"=w259:errorcluster)
    }
    frame #1 {
      n106 = Wait (ms)(milliseconds to wait=u32 1000) -> ()  [unwired: 1 out]
    }
    frame #2 {
      w432 = TRUE
      n107 = xnode "Read/Write Control"("FPGA VI Reference In"=w434, "error in"=w433, "+ phase"=w432, "+ phase (GI)"=w432, "+ phase (MCL)"=w432, "+ phase (APD Acq)"=w432, "+ phase (APD 1 Gate)"=w432, "+ phase (APD 2 Gate)"=w432, "+ phase (Green FB)"=w432, "+ phase (GI) 2"=w432) -> ("FPGA VI Reference Out"=w435:T15, "error out"=w436:errorcluster)
    }
    frame #3 {
      n108 = Wait (ms)(milliseconds to wait=u32 1000) -> ()  [unwired: 1 out]
    }
  }
  n109 = local read "Phase adj. (Green FB)"() -> (w71:i16)
  n110 = local read "Phase adj. (GI) 2"() -> (w41:i16)
  n111 = local read "Phase adjust (MCL)"() -> (w148:i16)
  n112 = local read "Phase adj. (AI1)"() -> (w150:i16)
  n113 = local read "Phase adj. (GI)"() -> (w149:i16)
  n114 = xnode "Read/Write Control"("FPGA VI Reference In"=w116, "error in"=w117, "Phase count adjustment"=w150, "Phase count adjustment (GI)"=w149, "Phase count adjustment (MCL)"=w148, "Phase Count Adjustment (APD Acq)"="Phase Adj. (APD Acq)", "Phase count adjustment (APD 1 Gate)"="Phase Adj. (APD 1 Gate)", "Phase count adjustment (APD 2 Gate)"="Phase Adj. (APD 2 Gate)", "Phase count adjustment (Green FB)"=w71, "Phase count adjustment (GI) 2"=w41) -> ("FPGA VI Reference Out"=w27:T15, "error out"=w125:errorcluster)
  n115 = call "Initialize RF boards - interlace 3.vi"("error in"=w125, "FPGA VI Reference In"=w27) -> ("error out"=w123:errorcluster, "FPGA VI Reference Out"=w124:T15)
  n116 = call "set RF board frequency - interlace.vi"("Board 2 Frequency Limits"=w76, "Board 1 Frequency Limits"=w78, "error in"=w123, "FPGA VI Reference In"=w124, "Board 2 Frequency 3 (MHz)"="BD 2 Frequency 3 (MHz)", "Board 1 Frequency 3 (MHz)"="BD 1 Frequency 3 (MHz)", "Board 2 Frequency 2 (MHz)"="BD 2 Frequency 2 (MHz)", "Board 2 Frequency 1 (MHz)"="BD 2 Frequency 1 (MHz)", "Board 1 Frequency 2 (MHz)"="BD 1 Frequency 2 (MHz)", "Board 1 Frequency 1  (MHz)"="BD 1 Frequency 1 (MHz)") -> ("error out"=w231:errorcluster, "FPGA VI Reference Out"=w232:T15)
  n117 = call "set RF board amplitude - interlace.vi"("Board 2 Amplitude Limits"=w75, "Board 1 Amplitude Limits"=w77, "error in"=w231, "FPGA VI Reference In"=w232, "Board 2 Amplitude 3 (%)"="BD 2 Amplitude 3 (%)", "Board 1 Amplitude 3 (%)"="BD 1 Amplitude 3 (%)", "Board 2 Amplitude 2 (%)"="BD 2 Amplitude 2 (%)", "Board 2 Amplitude 1 (%)"="BD 2 Amplitude 1 (%)", "Board 1 Amplitude 2 (%)"="BD 1 Amplitude 2 (%)", "Board 1 Amplitude 1 (%)"="BD 1 Amplitude 1 (%)") -> ("error out"=w219:errorcluster, "FPGA VI Reference Out"=w220:T15)
  n118 = flat-sequence {
    tunnel: w220 -> [w625]
    tunnel: w219 -> [w624]
    tunnel: [w623] -> w224
    tunnel: [w622] -> w223
    tunnel: [w666] -> w222
    tunnel: w224 -> [w666]
    tunnel: [w665] -> w221
    tunnel: w223 -> [w665]
    tunnel: w222 -> [w674]
    tunnel: w221 -> [w673]
    tunnel: [w672] -> w89
    tunnel: [w671] -> w88
    frame #0 {
      n119 = local read "Trap 1 (ON/OFF)"() -> (w617:bool)
      n120 = xnode "Read/Write Control"("FPGA VI Reference In"=w625, "error in"=w624, "Direct RF Box  Communication"=FALSE) -> ("FPGA VI Reference Out"=w623:T15, "error out"=w622:errorcluster)
      n121 = local write "Saving..."(FALSE ("Saving Data")) -> ()
      n122 = local write "Stop All"(FALSE ("Stop All")) -> ()
      n123 = local write "Index"(1.0 ("Index")) -> ()
      n124 = property on="Trap 1 ON" class="Bool (strict)"("Value"=w617) -> ()  [unwired: 2 in, 2 out]
      "Manipulating Trap" <- FALSE ("Manipulating Trap")
    }
    frame #1 {
      n125 = local read "Trap 2 (ON/OFF)"() -> (w664:bool)
      n126 = Wait (ms)(milliseconds to wait=u32 10) -> ()  [unwired: 1 out]
      n127 = property on="Trap 2 ON" class="Bool (strict)"("Val(Sgnl)"=w664) -> ()  [unwired: 2 in, 2 out]
    }
    frame #2 {
      n128 = xnode "Read/Write Control"("FPGA VI Reference In"=w674, "error in"=w673, "FPGA Controls  RF Box"=TRUE ("Direct RF Box  Communication")) -> ("FPGA VI Reference Out"=w672:T15, "error out"=w671:errorcluster)
      n129 = call "Update messages.vi"("Message to add"="UHR-Fleezers ready.", "Old message string"="") -> ("New message string"=w670:string)
      n130 = local write "Messages"(w670) -> ()
    }
  }
  n131 = Subtract(x="BD 1 Frequency 1 (MHz)", y="BD 1 Frequency 2 (MHz)") -> (x-y=w135:dbl)
  n132 = Subtract(x="BD 2 Frequency 1 (MHz)", y="BD 2 Frequency 2 (MHz)") -> (x-y=w134:dbl)
  n133 = Square(x=w134) -> (x^2=w132:dbl)
  n134 = Square(x=w135) -> (x^2=w133:dbl)
  n135 = Add(x=w133, y=w132) -> (x+y=w131:dbl)
  n136 = Square Root(x=w131) -> (sqrt(x)=w130:dbl)
  n137 = local write "Trap Delta (MHz)"(w130) -> ()
  n138 = xnode "Read/Write Control"("FPGA VI Reference In"=w89, "error in"=w88, "AI to FIFO"=w87, "APD to FIFO"=w87) -> ("FPGA VI Reference Out"=w86:T15, "error out"=w85:errorcluster)
  n139 = call-poly "VISA Configure Serial Port"("VISA resource name"="Sample Chamber Stage Serial Port") -> ("VISA resource name out"=w22:refnum<visa-resource-name>, "error out"=w23:errorcluster)  [unwired: 5 in, 8 out]
  "Stage Control Serial Error" <- w23
  n140 = call "IMAQ Create"("Image Name"="APD 1 Image", "Image Type"=w11) -> ("New Image"=w10:T2)  [unwired: 3 in, 1 out]
  n141 = call "IMAQ Create"("Image Name"="APD 2 Image", "Image Type"=w11) -> ("New Image"=w9:T2)  [unwired: 3 in, 1 out]
  n142 = call "IMAQ Create"("Image Name"="Det. X Image", "Image Type"=w11) -> ("New Image"=w8:T2)  [unwired: 3 in, 1 out]
  n143 = call "IMAQ Create"("Image Name"="Det. Y Image", "Image Type"=w11) -> ("New Image"=w7:T2)  [unwired: 3 in, 1 out]
  n144 = call-poly "VISA Configure Serial Port"("VISA resource name"="Harvard Syringe Pump Serial Port", "baud rate (9600)"=u32 115200, "stop bits (10: 1 bit)"=w4) -> ("VISA resource name out"=w1:refnum<visa-resource-name>, "error out"=w2:errorcluster)  [unwired: 4 in, 7 out]
  n145 = Bundle("New Image"=w10, "New Image"=w9, "New Image"=w8, "New Image"=w7) -> (w6:T18)  [unwired: 1 in]
  n146 = node-c288(i64 1 ("Period")) -> (w139:T19)  [unwired: 3 out]
  n147 = node-c288() -> (w31:T19)  [unwired: 4 out]
  n148 = node-c288() -> (w29:T19)  [unwired: 4 out]
  n149 = node-c288() -> (w33:T19)  [unwired: 4 out]
  n150 = node-c288() -> (w18:T19)  [unwired: 4 in]
  n151 = timed-loop "Acquire Data" {
    tunnel: w86 -> [w904]
    tunnel: w85 -> [w903]
    tunnel: [w939] -> w239
    tunnel: [w933] -> w237
    timing: w139 -> [_]
    timing-out: [_] -> w138
    tunnel: w6 -> [w714]
    stop <- "Stop All" stop-if-true
    w790 = "NI_ChannelName" ("name")
    n152 = node-c288() -> ()  [unwired: 2 out]
    n153 = case "Reset data stream" shown="True" "Reset" {
      tunnel: w904 -> [w3205 w3212]
      tunnel: w903 -> [w3204 w3211]
      tunnel: [w3205 w3207] -> w899
      tunnel: [w3204 w3206] -> w898
      frame #0 {
      }
      frame #1 {
        w3210 = TRUE ("AI to FIFO")
        w3217 = FALSE ("AI to FIFO")
        n154 = local write "Overflow (data lost)"(FALSE ("Overflow (data lost)")) -> ()
        n155 = xnode "Read/Write Control"("FPGA VI Reference In"=w3212, "error in"=w3211, "AI to FIFO"=w3217, "APD to FIFO"=w3217) -> ("FPGA VI Reference Out"=w3215:T15, "error out"=w3216:errorcluster)
        n156 = xnode "Invoke Method"("FPGA VI Reference In"=w3215, "error in"=w3216) -> ("FPGA VI Reference Out"=w3213:T15, "error out"=w3214:errorcluster)
        n157 = xnode "Invoke Method"("FPGA VI Reference In"=w3213, "error in"=w3214) -> ("FPGA VI Reference Out"=w3209:T15, "error out"=w3208:errorcluster)
        n158 = xnode "Read/Write Control"("FPGA VI Reference In"=w3209, "error in"=w3208, "AI to FIFO"=w3210, "APD to FIFO"=w3210) -> ("FPGA VI Reference Out"=w3207:T15, "error out"=w3206:errorcluster)
      }
    }
    n159 = Or(x="Start AOD Scan", y="Trap Raster Scan") -> (x .or. y?=w849:bool)
    n160 = And(x="Save scans", y=w849) -> (x .and. y?=w895:bool)
    n161 = case "Start AOM raster scan" shown="True" w849 {
      tunnel: w899 -> [w2443 w2453]
      tunnel: w898 -> [w2442 w2452]
      tunnel: [w2443 w2446] -> w897
      tunnel: [w2442 w2445] -> w896
      frame #0 {
      }
      frame #1 {
        n162 = case shown="True" "Restart DMA? (AOD)" {
          tunnel: [w2819 w2820] -> w2447
          tunnel: [w2818 w2821] -> w2448
          tunnel: w2453 -> [w2819 w2827]
          tunnel: w2452 -> [w2818 w2826]
          frame #0 {
          }
          frame #1 {
            w2823 = FALSE ("AI to FIFO")
            n163 = xnode "Read/Write Control"("FPGA VI Reference In"=w2827, "error in"=w2826, "AI to FIFO"=w2823, "APD to FIFO"=w2823) -> ("FPGA VI Reference Out"=w2825:T15, "error out"=w2824:errorcluster)
            n164 = xnode "Invoke Method"("FPGA VI Reference In"=w2825, "error in"=w2824) -> ("FPGA VI Reference Out"=w2829:T15, "error out"=w2828:errorcluster)
            n165 = xnode "Invoke Method"("FPGA VI Reference In"=w2829, "error in"=w2828) -> ("FPGA VI Reference Out"=w2820:T15, "error out"=w2821:errorcluster)
            n166 = local write "Overflow (data lost)"(FALSE ("Overflow (data lost)")) -> ()
          }
        }
        n167 = case shown="True" "Move MCL Also?" {
          tunnel: w2448 -> [w2456 w2562]
          tunnel: w2447 -> [w2457 w2563]
          tunnel: [w2455 w2566] -> w2446
          tunnel: [w2454 w2565] -> w2445
          frame #0 {
            w2458 = TRUE ("AI to FIFO")
            n168 = xnode "Read/Write Control"("FPGA VI Reference In"=w2457, "error in"=w2456, "AI to FIFO"=w2458, "APD to FIFO"=w2458, "Start scan"=w2458) -> ("FPGA VI Reference Out"=w2455:T15, "error out"=w2454:errorcluster)
          }
          frame #1 {
            w2559 = FALSE ("1D or 2D Scan?")
            w2564 = TRUE ("AI to FIFO")
            # "Count for MCL loop"
            # "N total cycles"
            # "N steps"
            # "V_int"
            n169 = local read "Scan Range (nm)"() -> (w2541:dbl)
            n170 = local read "Number of F/B Scans (AOD)"() -> (w2558:u16)
            n171 = Sign(1:w2541) -> (0:w2540:dbl)
            n172 = Compound Arithmetic op=MULTIPLY(w2541, "MCL Step Position Ratio", "MCL/AOM Scale Tweak") -> (w2545:dbl)
            n173 = Negate(x=w2540) -> (-x=w2537:dbl)
            n174 = Multiply(x=w2537, y="MCL Step Increment (V_int)") -> (x*y=w2539:dbl)
            n175 = Divide(x=w2545, y="MCL X Cal (nm/V)") -> (x/y=w2551:dbl)
            n176 = Multiply(x=32767.0 ("y"), y=w2551) -> (x*y=w2557:dbl)
            n177 = local read "Total Counts (ticks)"() -> (w2542:u32)
            n178 = local read "Cycles/step (AOD)"() -> (w2553:u64)
            n179 = local read "Scan steps (AOD)"() -> (w2554:u64)
            n180 = Divide(x=w2557, y=10.0) -> (x/y=w2550:dbl)
            n181 = Divide(x=w2550, y="MCL Step Increment (V_int)") -> (x/y=w2548:dbl)
            n182 = Absolute Value(x=w2548) -> (abs(x)=w2536:dbl)
            n183 = Compound Arithmetic op=MULTIPLY(w2554, w2553, w2542) -> (w2549:u64)
            n184 = local write "wait to reset values"(w2564) -> ()
            n185 = local write "MCL Scanning"(w2564) -> ()
            n186 = Divide(x=w2549, y=w2536) -> (x/y=w2546:dbl)
            "MCL Count" <- w2546
            n187 = xnode "Read/Write Control"("FPGA VI Reference In"=w2563, "error in"=w2562, "Scan steps (MCL)"=w2536, "Number of scans (MCL)"=w2558, "Cycles per step (MCL)"=u64 1, "Scan freq.  increment (MCL)"=w2539, "1D or 2D Scan?"=w2559, "MCL Scan Axis"=w2559, "Cont. Scan (MCL)"=w2559, "MCL count"=w2546) -> ("FPGA VI Reference Out"=w2561:T15, "error out"=w2560:errorcluster)
            n188 = xnode "Read/Write Control"("FPGA VI Reference In"=w2561, "error in"=w2560, "AI to FIFO"=w2564, "APD to FIFO"=w2564, "Start scan"=w2564, "Start scan (MCL)"=w2564) -> ("FPGA VI Reference Out"=w2566:T15, "error out"=w2565:errorcluster)
          }
        }
        n189 = local write "Trap Raster Scan"(FALSE ("Trap Raster Scan")) -> ()
        "Raster Scanning..." <- TRUE ("Scanning...")
      }
    }
    n190 = Compound Arithmetic op=OR("Start MCL Scan", "Confocal Image", "Confocal Linescan") -> (w847:bool)
    n191 = And(x="Save Data (MCL)", y=w847) -> (x .and. y?=w894:bool)
    n192 = case "Start MCL raster scan" shown="True" w847 {
      tunnel: w897 -> [w1627 w1642]
      tunnel: w896 -> [w1626 w1641]
      tunnel: [w1627 w1637] -> w785
      tunnel: [w1626 w1636] -> w784
      tunnel: [FALSE w1635] -> w880
      tunnel: "Start MCL Scan" -> [_ w1630]
      tunnel: "Confocal Image" -> [_ w1629]
      tunnel: "Confocal Linescan" -> [_ _]
      frame #0 {
      }
      frame #1 {
        w1635 = TRUE
        n193 = case shown="True" "Restart DMA? (MCL)" {
          tunnel: [w1879 w1882] -> w1640
          tunnel: [w1878 w1881] -> w1639
          tunnel: w1642 -> [w1879 w1887]
          tunnel: w1641 -> [w1878 w1886]
          frame #0 {
          }
          frame #1 {
            w1883 = FALSE ("AI to FIFO")
            n194 = xnode "Read/Write Control"("FPGA VI Reference In"=w1887, "error in"=w1886, "AI to FIFO"=w1883, "APD to FIFO"=w1883) -> ("FPGA VI Reference Out"=w1885:T15, "error out"=w1884:errorcluster)
            n195 = xnode "Invoke Method"("FPGA VI Reference In"=w1885, "error in"=w1884) -> ("FPGA VI Reference Out"=w1889:T15, "error out"=w1888:errorcluster)
            n196 = xnode "Invoke Method"("FPGA VI Reference In"=w1889, "error in"=w1888) -> ("FPGA VI Reference Out"=w1882:T15, "error out"=w1881:errorcluster)
            n197 = local write "Overflow (data lost)"(FALSE ("Overflow (data lost)")) -> ()
          }
        }
        n198 = case shown="False" w1630 {
          selector: w1630 -> [_ w1646]
          tunnel: w1629 -> [w1645 _]
          tunnel: [w1645 w1646] -> w1628
          frame #0 {
            n199 = property on="2D or 1D Scan" class="Bool (strict)"("Val(Sgnl)"=w1645) -> ()  [unwired: 2 in, 2 out]
            n200 = property on="Confocal Image" class="Bool (strict)"("Value"=FALSE ("Start Confocal Map")) -> ()  [unwired: 2 in, 2 out]
          }
          frame #1 {
          }
        }
        n201 = local write "MCL Scanning"(w1635) -> ()
        n202 = local read "AO1"() -> (w1632:dbl)
        n203 = local read "AO2"() -> (w1631:dbl)
        n204 = case shown="True" "Center Scan" {
          tunnel: w1640 -> [w1653 w1762]
          tunnel: w1639 -> [w1652 w1761]
          tunnel: [w1651 w1760] -> w1637
          tunnel: [w1650 w1759] -> w1636
          tunnel: [w1648 w1746] -> w1634
          tunnel: [w1647 w1745] -> w1633
          tunnel: w1632 -> [w1648 w1751]
          tunnel: w1631 -> [w1647 w1754]
          tunnel: w1628 -> [_ _]
          frame #0 {
            w1649 = TRUE ("AI to FIFO")
            n205 = xnode "Read/Write Control"("FPGA VI Reference In"=w1653, "error in"=w1652, "AI to FIFO"=w1649, "APD to FIFO"=w1649, "Start scan (MCL)"=w1649) -> ("FPGA VI Reference Out"=w1651:T15, "error out"=w1650:errorcluster)
          }
          frame #1 {
            w1758 = TRUE ("AI to FIFO")
            n206 = local read "Scan steps (MCL)"() -> (w1737:u64)
            n207 = local read "Scan lines (y)"() -> (w1733:u64)
            n208 = local read "Fast Scan Dir"() -> (w1744:bool)
            n209 = local read "Actual MCL Inc (V)"() -> (w1734:dbl)
            n210 = Decrement(x=w1733) -> (x-1=w1732:u64)
            n211 = Decrement(x=w1737) -> (x-1=w1736:u64)
            n212 = Multiply(x=w1734, y=w1732) -> (x*y=w1731:dbl)
            n213 = Divide(x=w1731, y=2.0) -> (x/y=w1741:dbl)
            n214 = Multiply(x=w1734, y=w1736) -> (x*y=w1735:dbl)
            n215 = Divide(x=w1735, y=2.0) -> (x/y=w1740:dbl)
            n216 = Select(t=w1740, s=w1744, f=w1741) -> (s? t:f=w1739:dbl)
            n217 = Select(t=w1741, s=w1744, f=w1740) -> (s? t:f=w1743:dbl)
            n218 = Subtract(x=w1751, y=w1743) -> (x-y=w1742:dbl)
            n219 = Subtract(x=w1754, y=w1739) -> (x-y=w1738:dbl)
            n220 = local read "2D or 1D Scan"() -> (w1756:bool)
            n221 = Not(x=w1744) -> (.not. x?=w1750:bool)
            n222 = Not(x=w1756) -> (.not. x?=w1752:bool)
            n223 = And(x=w1744, y=w1752) -> (x .and. y?=w1753:bool)
            n224 = And(x=w1752, y=w1750) -> (x .and. y?=w1755:bool)
            n225 = Select(t=w1754, s=w1755, f=w1738) -> (s? t:f=w1745:dbl)
            n226 = Select(t=w1751, s=w1753, f=w1742) -> (s? t:f=w1746:dbl)
            n227 = call "Volt to I16.vi"("Voltage In"=w1746) -> ("I16 Voltage Out"=w1749:i16)
            n228 = call "Volt to I16.vi"("Voltage In"=w1745) -> ("I16 Voltage Out"=w1748:i16)
            n229 = xnode "Read/Write Control"("FPGA VI Reference In"=w1762, "error in"=w1761, "AI to FIFO"=w1758, "APD to FIFO"=w1758, "Start scan (MCL)"=w1758, "AO1"=w1749, "AO2"=w1748) -> ("FPGA VI Reference Out"=w1760:T15, "error out"=w1759:errorcluster)
          }
        }
        "Initial Y" <- w1634
        "Initial X" <- w1633
        "wait to reset values" <- w1635
      }
    }
    n230 = local read "APD Elements/DMA read"() -> (w753:u32)
    n231 = local read "Elements/DMA read"() -> (w808:u32)
    n232 = xnode "Get APD Data"("FPGA VI Reference In"=w785, "error in"=w784, "Number of Elements"=w753, "Timeout (ms)"=-1) -> ("Data"=w752:u32[], "Elements Remaining"=→"APD FIFO Elements Remaining":u32)  [unwired: 2 out]
    n233 = xnode "Get Trap Data"("FPGA VI Reference In"=w785, "error in"=w784, "Number of Elements"=w808, "Timeout (ms)"=-1 ("Timeout")) -> ("FPGA VI Reference Out"=w787:T15, "error out"=w786:errorcluster, "Data"=w918:u32[], "Elements Remaining"=w948:u32)
    "FIFO El. Rem." <- w948
    n234 = local read "FIFO Depth"() -> (w950:u32)
    n235 = Subtract(x=w950, y=w808) -> (x-y=w949:u32)
    n236 = Divide(x=w948, y=w949) -> (x/y=w947:dbl)
    "Buffer Status" <- w947
    n237 = Equal?(x=w947, y=1.0) -> (x = y?=w945:bool)
    n238 = case "Alert buffer overflow" shown="True" w945 {
      frame #0 {
      }
      frame #1 {
        n239 = call <vilib>:"Beep.vi"() -> ()  [unwired: 3 in, 9 out]
        "Overflow (data lost)" <- TRUE ("Overflow (data lost)")
      }
    }
    n240 = local read "FPGA Averaging"() -> (w807:bool)
    n241 = case "Special unpacking case if no averaging done by FPGA" shown="False" w807 {
      tunnel: w918 -> [w2039 w2065]
      tunnel: [w2010 w2040] -> w917
      frame #0 {
        n242 = Decimate 1D Array(w2039) -> (w2038:u32[], w2037:u32[], w2036:u32[], w2035:u32[])
        n243 = Split Number(x=w2038) -> (hi(x)=w2034:u16[], lo(x)=w2033:u16[])
        n244 = Split Number(x=w2037) -> (hi(x)=w2032:u16[], lo(x)=w2031:u16[])
        n245 = Split Number(x=w2036) -> (hi(x)=w2030:u16[], lo(x)=w2029:u16[])
        n246 = Split Number(x=w2035) -> (hi(x)=w2028:u16[], lo(x)=w2027:u16[])
        n247 = To Word Integer(number=w2034) -> (16bit integer=w2026:i16[])
        n248 = To Word Integer(number=w2033) -> (16bit integer=w2025:i16[])
        n249 = To Word Integer(number=w2032) -> (16bit integer=w2024:i16[])
        n250 = To Word Integer(number=w2031) -> (16bit integer=w2023:i16[])
        n251 = To Word Integer(number=w2030) -> (16bit integer=w2022:i16[])
        n252 = To Word Integer(number=w2029) -> (16bit integer=w2021:i16[])
        n253 = To Word Integer(number=w2028) -> (16bit integer=w2020:i16[])
        n254 = To Word Integer(number=w2027) -> (16bit integer=w2019:i16[])
        n255 = To Double Precision Float(number=w2026) -> (double precision float=w2018:dbl[])
        n256 = To Double Precision Float(number=w2025) -> (double precision float=w2017:dbl[])
        n257 = To Double Precision Float(number=w2024) -> (double precision float=w2016:dbl[])
        n258 = To Double Precision Float(number=w2023) -> (double precision float=w2015:dbl[])
        n259 = To Double Precision Float(number=w2022) -> (double precision float=w2014:dbl[])
        n260 = To Double Precision Float(number=w2021) -> (double precision float=w2013:dbl[])
        n261 = To Double Precision Float(number=w2020) -> (double precision float=w2012:dbl[])
        n262 = To Double Precision Float(number=w2019) -> (double precision float=w2011:dbl[])
        n263 = Interleave 1D Arrays(w2018, w2017, w2016, w2015, w2014, w2013, w2012, w2011) -> (w2010:dbl[])
      }
      frame #1 {
        n264 = Decimate 1D Array(w2065) -> (w2056:u32[], w2054:u32[], w2052:u32[], w2050:u32[], w2048:u32[], w2046:u32[], w2044:u32[], w2042:u32[])
        n265 = To Long Integer(number=w2056) -> (32bit integer=w2064:i32[])
        n266 = To Long Integer(number=w2054) -> (32bit integer=w2063:i32[])
        n267 = To Long Integer(number=w2052) -> (32bit integer=w2062:i32[])
        n268 = To Long Integer(number=w2050) -> (32bit integer=w2061:i32[])
        n269 = To Long Integer(number=w2048) -> (32bit integer=w2060:i32[])
        n270 = To Long Integer(number=w2046) -> (32bit integer=w2059:i32[])
        n271 = To Long Integer(number=w2044) -> (32bit integer=w2058:i32[])
        n272 = To Long Integer(number=w2042) -> (32bit integer=w2057:i32[])
        n273 = To Double Precision Float(number=w2064) -> (double precision float=w2055:dbl[])
        n274 = To Double Precision Float(number=w2063) -> (double precision float=w2053:dbl[])
        n275 = To Double Precision Float(number=w2062) -> (double precision float=w2051:dbl[])
        n276 = To Double Precision Float(number=w2061) -> (double precision float=w2049:dbl[])
        n277 = To Double Precision Float(number=w2060) -> (double precision float=w2047:dbl[])
        n278 = To Double Precision Float(number=w2059) -> (double precision float=w2045:dbl[])
        n279 = To Double Precision Float(number=w2058) -> (double precision float=w2043:dbl[])
        n280 = To Double Precision Float(number=w2057) -> (double precision float=w2041:dbl[])
        n281 = Interleave 1D Arrays(w2055, w2053, w2051, w2049, w2047, w2045, w2043, w2041) -> (w2040:dbl[])
      }
    }
    n282 = local read "FPGA Ave."() -> (w806:dbl)
    n283 = feedback #1(i16 -1 ("Trap Sets")) -> (w804:i16)
    n284 = feedback #2("" ("Detector Type")) -> (w801:string)
    n285 = Not Equal?(x=w801, y="Detector Type") -> (x != y?=w799:bool)
    n286 = local read "Trap Sets"() -> (w803:i16)
    n287 = Not Equal?(x=w804, y=w803) -> (x != y?=w798:bool)
    n288 = Or(x=w799, y=w798) -> (x .or. y?=w797:bool)
    n289 = Divide(x=w917, y=w806) -> (x/y=w925:dbl[])
    n290 = case "Deinterlace trap data, average down PSD" shown="2" w803 {
      tunnel: w925 -> [w2084 w2149]
      tunnel: [w2081 w2146] -> w791
      tunnel: [w2084 w2148] -> w924
      tunnel: "Detector Type" -> [w2083 w2144]
      tunnel: [w2082 w2147] -> w789
      tunnel: [w2080 w2145] -> w916
      frame #0 {
        n291 = Divide(x=w2084, y=3276.7) -> (x/y=w2085:dbl[])
        n292 = Decimate 1D Array(w2085) -> (w2094:dbl[], w2093:dbl[], w2092:dbl[], w2091:dbl[], w2090:dbl[], w2089:dbl[], w2088:dbl[], w2087:dbl[])
        n293 = case shown="\"IR-QPD + PSD + FB-QPD position\"" w2083 {
          tunnel: w2094 -> [w2118 w2143]
          tunnel: w2093 -> [w2117 w2142]
          tunnel: w2092 -> [w2102 w2120]
          tunnel: w2091 -> [w2103 w2130]
          tunnel: w2090 -> [w2116 w2141]
          tunnel: w2089 -> [w2115 w2140]
          tunnel: w2088 -> [w2099 w2121]
          tunnel: w2087 -> [w2098 w2119]
          tunnel: [w2097 w2127] -> w2082
          tunnel: [w2096 w2126] -> w2081
          tunnel: [w2095 w2125] -> w2080
          frame #0 {
            w2095 = 0  # Channel pattern
            n294 = Divide(x=w2118, y=w2103) -> (x/y=w2105:dbl[])
            n295 = Divide(x=w2117, y=w2103) -> (x/y=w2104:dbl[])
            n296 = Divide(x=w2116, y=w2099) -> (x/y=w2101:dbl[])
            n297 = Divide(x=w2115, y=w2098) -> (x/y=w2100:dbl[])
            n298 = Build Array(w2105, w2104, w2103, w2102, w2101, w2100, w2099, w2098) -> (w2096:dbl[][])
            n299 = Bundle("T1 Y", "T1 X", "T1 Sum", "FB Sum", "PSD Y", "PSD X", "PSD Y Sum", "PSD X Sum") -> (w2114:T31)  [unwired: 1 out]
            n300 = Cluster To Array(cluster=w2114) -> (array=w2097:string[])
          }
          frame #1 {
            w2125 = 3  # Channel pattern
            n301 = Negate(x=w2121) -> (-x=w2122:dbl[])
            n302 = Divide(x=w2143, y=w2130) -> (x/y=w2132:dbl[])
            n303 = Divide(x=w2142, y=w2130) -> (x/y=w2131:dbl[])
            n304 = Divide(x=w2141, y=w2121) -> (x/y=w2129:dbl[])
            n305 = Divide(x=w2140, y=w2122) -> (x/y=w2128:dbl[])
            n306 = Build Array(w2132, w2131, w2130, w2119, w2120, w2129, w2128, w2121) -> (w2126:dbl[][])
            n307 = Bundle("T1 Y", "T1 X", "T1 Sum", "FB X", "FB Sum", "PSD Y", "PSD X", "PSD Y Sum") -> (w2139:T31)  [unwired: 1 out]
            n308 = Cluster To Array(cluster=w2139) -> (array=w2127:string[])
          }
        }
      }
      frame #1 {
        n309 = case shown="\"IR-QPD + PSD + FB-QPD X position\"" w2144 {
          tunnel: w2149 -> [w2210 w2277 w2347]
          tunnel: [w2190 w2262 w2334] -> w2148
          tunnel: [w2176 w2253 w2325] -> w2147
          tunnel: [w2175 w2213 w2292] -> w2146
          tunnel: [w2169 w2251 w2323] -> w2145
          frame #0 {
            w2169 = 1  # Channel pattern
            # "time average x2 the 4th signal and the 4 psd signals (detection laser)"
            # "deinterlace 3 signals from qpd"
            n310 = Decimate 1D Array(w2210) -> (w2209:dbl[], w2208:dbl[], w2174:dbl[], w2207:dbl[], w2197:dbl[], w2195:dbl[], w2194:dbl[], w2192:dbl[])
            n311 = Decimate 1D Array(w2174) -> (w2173:dbl[], w2172:dbl[])
            n312 = Decimate 1D Array(w2209) -> (w2206:dbl[], w2178:dbl[])
            n313 = Decimate 1D Array(w2208) -> (w2205:dbl[], w2203:dbl[])
            n314 = Decimate 1D Array(w2207) -> (w2204:dbl[], w2202:dbl[])
            n315 = call "downsample 1D array - double.vi"("Ave N"=2.0, "Array In"=w2197) -> ("Array Out"=w2196:dbl[])  [unwired: 1 out]
            n316 = call "downsample 1D array - double.vi"("Ave N"=2.0, "Array In"=w2195) -> ("Array Out"=w2177:dbl[])  [unwired: 1 out]
            n317 = call "downsample 1D array - double.vi"("Ave N"=2.0, "Array In"=w2194) -> ("Array Out"=w2193:dbl[])  [unwired: 1 out]
            n318 = call "downsample 1D array - double.vi"("Ave N"=2.0, "Array In"=w2192) -> ("Array Out"=w2191:dbl[])  [unwired: 1 out]
            n319 = Interleave 1D Arrays(w2206, w2205, w2204, w2178, w2203, w2202, w2173, w2172, w2196, w2177, w2193, w2191) -> (w2190:dbl[])
            n320 = Divide(x=w2190, y=3276.7) -> (x/y=w2189:dbl[])
            n321 = Decimate 1D Array(w2189) -> (w2188:dbl[], w2187:dbl[], w2186:dbl[], w2185:dbl[], w2184:dbl[], w2183:dbl[], w2171:dbl[], w2170:dbl[], w2182:dbl[], w2181:dbl[], w2180:dbl[], w2179:dbl[])
            n322 = Divide(x=w2188, y=w2186) -> (x/y=w2156:dbl[])
            n323 = Divide(x=w2187, y=w2186) -> (x/y=w2155:dbl[])
            n324 = Divide(x=w2185, y=w2183) -> (x/y=w2154:dbl[])
            n325 = Divide(x=w2184, y=w2183) -> (x/y=w2153:dbl[])
            n326 = Divide(x=w2182, y=w2180) -> (x/y=w2152:dbl[])
            n327 = Divide(x=w2181, y=w2179) -> (x/y=w2151:dbl[])
            n328 = Build Array(w2156, w2155, w2186, w2154, w2153, w2183, w2171, w2170, w2152, w2151, w2180, w2179) -> (w2175:dbl[][])
            n329 = Bundle("T1 Y", "T1 X", "T1 Sum", "T2 Y", "T2 X", "T2 Sum", "T1 FB Sum", "T2 FB Sum", "PSD Y", "PSD X", "PSD Y Sum", "PSD X Sum") -> (w2157:T32)  [unwired: 1 out]
            n330 = Cluster To Array(cluster=w2157) -> (array=w2176:string[])
          }
          frame #1 {
            w2251 = 2  # Channel pattern
            # "time average x2 the 3 psd signals (detection laser)"
            # "deinterlace 3 signals from qpds"
            n331 = Decimate 1D Array(w2277) -> (w2276:dbl[], w2275:dbl[], w2252:dbl[], w2274:dbl[], w2265:dbl[], w2264:dbl[], w2263:dbl[], w2239:dbl[])
            n332 = Decimate 1D Array(w2252) -> (w2234:dbl[], w2232:dbl[])
            n333 = Decimate 1D Array(w2276) -> (w2273:dbl[], w2254:dbl[])
            n334 = Decimate 1D Array(w2275) -> (w2272:dbl[], w2270:dbl[])
            n335 = Decimate 1D Array(w2274) -> (w2271:dbl[], w2269:dbl[])
            n336 = Decimate 1D Array(w2239) -> (w2235:dbl[], w2233:dbl[])
            n337 = call "downsample 1D array - double.vi"("Ave N"=2.0, "Array In"=w2265) -> ("Array Out"=w2238:dbl[])  [unwired: 1 out]
            n338 = call "downsample 1D array - double.vi"("Ave N"=2.0, "Array In"=w2264) -> ("Array Out"=w2237:dbl[])  [unwired: 1 out]
            n339 = call "downsample 1D array - double.vi"("Ave N"=2.0, "Array In"=w2263) -> ("Array Out"=w2236:dbl[])  [unwired: 1 out]
            n340 = Interleave 1D Arrays(w2273, w2272, w2271, w2254, w2270, w2269, w2235, w2234, w2233, w2232, w2238, w2237, w2236) -> (w2262:dbl[])
            n341 = Divide(x=w2262, y=3276.7) -> (x/y=w2261:dbl[])
            n342 = Decimate 1D Array(w2261) -> (w2260:dbl[], w2259:dbl[], w2258:dbl[], w2257:dbl[], w2256:dbl[], w2255:dbl[], w2224:dbl[], w2222:dbl[], w2221:dbl[], w2219:dbl[], w2218:dbl[], w2217:dbl[], w2214:dbl[])
            n343 = Negate(x=w2214) -> (-x=w2212:dbl[])
            n344 = Divide(x=w2218, y=w2214) -> (x/y=w2216:dbl[])
            n345 = Divide(x=w2217, y=w2212) -> (x/y=w2215:dbl[])
            n346 = Divide(x=w2260, y=w2258) -> (x/y=w2243:dbl[])
            n347 = Divide(x=w2259, y=w2258) -> (x/y=w2242:dbl[])
            n348 = Divide(x=w2257, y=w2255) -> (x/y=w2241:dbl[])
            n349 = Divide(x=w2256, y=w2255) -> (x/y=w2240:dbl[])
            n350 = Divide(x=w2224, y=w2222) -> (x/y=w2223:dbl[])
            n351 = Divide(x=w2221, y=w2219) -> (x/y=w2220:dbl[])
            n352 = Build Array(w2243, w2242, w2258, w2241, w2240, w2255, w2223, w2222, w2220, w2219, w2216, w2215, w2214) -> (w2213:dbl[][])
            n353 = Bundle("T1 Y", "T1 X", "T1 Sum", "T2 Y", "T2 X", "T2 Sum", "T1 FB X", "T1 FB Sum", "T2 FB X", "T2 FB Sum", "PSD Y", "PSD X", "PSD Y Sum") -> (w2244:T33)  [unwired: 1 out]
            n354 = Cluster To Array(cluster=w2244) -> (array=w2253:string[])
          }
          frame #2 {
            w2323 = 4  # Channel pattern
            # "time average x2 the 3 psd signals (detection laser)"
            # "deinterlace 3 signals from qpds"
            n355 = Decimate 1D Array(w2347) -> (w2346:dbl[], w2345:dbl[], w2324:dbl[], w2344:dbl[], w2290:dbl[], w2336:dbl[], w2335:dbl[], w2312:dbl[])
            n356 = Decimate 1D Array "Feedback Sum"(w2324) -> (w2308:dbl[], w2306:dbl[])
            n357 = Decimate 1D Array "QPD Y"(w2346) -> (w2343:dbl[], w2326:dbl[])
            n358 = Decimate 1D Array "QPD X"(w2345) -> (w2342:dbl[], w2340:dbl[])
            n359 = Decimate 1D Array "Feedback Y"(w2290) -> (w2289:dbl[], w2288:dbl[])
            n360 = Decimate 1D Array "QPD Sum"(w2344) -> (w2341:dbl[], w2339:dbl[])
            n361 = Decimate 1D Array "Feedback X"(w2312) -> (w2309:dbl[], w2307:dbl[])
            n362 = call "downsample 1D array - double.vi"("Ave N"=2.0, "Array In"=w2336) -> ("Array Out"=w2311:dbl[])  [unwired: 1 out]
            n363 = call "downsample 1D array - double.vi"("Ave N"=2.0, "Array In"=w2335) -> ("Array Out"=w2310:dbl[])  [unwired: 1 out]
            n364 = Interleave 1D Arrays(w2343, w2342, w2341, w2326, w2340, w2339, w2289, w2309, w2308, w2288, w2307, w2306, w2311, w2310) -> (w2334:dbl[])
            n365 = Divide(x=w2334, y=3276.7) -> (x/y=w2333:dbl[])
            n366 = Decimate 1D Array(w2333) -> (w2332:dbl[], w2331:dbl[], w2330:dbl[], w2329:dbl[], w2328:dbl[], w2327:dbl[], w2285:dbl[], w2299:dbl[], w2283:dbl[], w2284:dbl[], w2297:dbl[], w2281:dbl[], w2295:dbl[], w2293:dbl[])
            n367 = Negate(x=w2293) -> (-x=w2291:dbl[])
            n368 = Divide(x=w2295, y=w2291) -> (x/y=w2294:dbl[])
            n369 = Divide(x=w2284, y=w2281) -> (x/y=w2280:dbl[])
            n370 = Divide(x=w2285, y=w2283) -> (x/y=w2282:dbl[])
            n371 = Divide(x=w2332, y=w2330) -> (x/y=w2316:dbl[])
            n372 = Divide(x=w2331, y=w2330) -> (x/y=w2315:dbl[])
            n373 = Divide(x=w2329, y=w2327) -> (x/y=w2314:dbl[])
            n374 = Divide(x=w2328, y=w2327) -> (x/y=w2313:dbl[])
            n375 = Divide(x=w2299, y=w2283) -> (x/y=w2298:dbl[])
            n376 = Divide(x=w2297, y=w2281) -> (x/y=w2296:dbl[])
            n377 = Build Array(w2316, w2315, w2330, w2314, w2313, w2327, w2282, w2298, w2283, w2280, w2296, w2281, w2294, w2293) -> (w2292:dbl[][])
            n378 = Bundle("T1 Y", "T1 X", "T1 Sum", "T2 Y", "T2 X", "T2 Sum", "T1 FB Y", "T1 FB X", "T1 FB Sum", "T2 FB Y", "T2 FB X", "T2 FB Sum", "PSD X", "PSD Y Sum") -> (w2279:T34)  [unwired: 1 out]
            n379 = Cluster To Array(cluster=w2279) -> (array=w2325:string[])
          }
        }
      }
    }
    n380 = case "Update these things only if detector type or number of traps changes" shown="True" w797 {
      tunnel: w789 -> [_ w1076]
      frame #0 {
      }
      frame #1 {
        n381 = property on="High Res. Display" class="Ring (strict)"("Strings []"=w1076) -> ()  [unwired: 2 in, 2 out]
        n382 = Build Array (concatenate)(w1076, "none") -> (w1069:string[])
        n383 = property on="FFT 1 Choice 1" class="Ring (strict)"("Strings []"=w1069) -> ()  [unwired: 2 in, 2 out]
        n384 = property on="FFT 1 Choice 2" class="Ring (strict)"("Strings []"=w1069) -> ()  [unwired: 2 in, 2 out]
        n385 = property on="FFT 2 Choice 1" class="Ring (strict)"("Strings []"=w1069) -> ()  [unwired: 2 in, 2 out]
        n386 = property on="FFT 2 Choice 2" class="Ring (strict)"("Strings []"=w1069) -> ()  [unwired: 2 in, 2 out]
        n387 = Bundle("APD 1", "APD 2") -> (w1072:cluster{string, string})  [unwired: 1 out]
        n388 = Cluster To Array(cluster=w1072) -> (array=w1070:string[])
        n389 = Build Array (concatenate)(w1070, w1069) -> (w1074:string[])
        n390 = Array Size(array=w1074) -> (size(s)=w1075:i32)
        n391 = property on="Signals to Plot" class="LstBox (strict)"("Item Names"=w1074) -> ()  [unwired: 2 in, 2 out]
        n392 = property on="Signals to Plot" class="LstBox (strict)"("Number of Rows"=w1075) -> ()  [unwired: 2 in, 2 out]
        n393 = property on="All Signals" class="WFChart (strict)"("LegNumRows"=w1075) -> ()  [unwired: 2 in, 2 out]
      }
    }
    n394 = local read "Data points/scans (MCL)"() -> (w889:dbl)
    n395 = Increment(x=w889) -> (x+1=w890:dbl)
    n396 = feedback #3(w890) -> (w893:dbl)
    n397 = Select(t=0, s=w880, f=w893) -> (s? t:f=w886:dbl)
    n398 = To Word Integer(number=w924) -> (16bit integer=w951:i16[])
    n399 = Decimate 1D Array(w752) -> (w783:u32[], w716:u32[])
    n400 = To Double Precision Float(number=w783) -> (double precision float=w782:dbl[])
    n401 = Array Size(array=w782) -> (size(s)=w892:i32)
    n402 = Add(x=w892, y=w886) -> (x+y=w887:dbl)
    n403 = Greater?(x=w887, y=w889) -> (0:w888:bool)
    n404 = local read "DMA Update Period (s)"() -> (w809:dbl)
    n405 = Select(t=w886, s=w888, f=w887) -> (s? t:f=w885:dbl)
    n406 = local read "MCL Scanning"() -> (w883:bool)
    n407 = Build Array(w783, w716) -> (w877:u32[][])
    n408 = local read "Data Period (s)"() -> (w768:dbl)
    n409 = To Double Precision Float(number=w877) -> (double precision float=w878:dbl[][])
    n410 = Not(x=w888) -> (.not. x?=w882:bool)
    n411 = To Double Precision Float(number=w716) -> (double precision float=w715:dbl[])
    n412 = local read "APD Integration Time (s)"() -> (w729:dbl)
    n413 = And(x=w882, y=w883) -> (x .and. y?=w884:bool)
    n414 = feedback #4(0.0) -> (w912:dbl)
    n415 = Add(x=w809, y=w912) -> (x+y=w920:dbl)
    n416 = Or(x=w884, y=w880) -> (x .or. y?=w881:bool)
    n417 = Multiply(x=w768, y="Trap Disp. Downsample") -> (x*y=w766:dbl)
    "Display Period (s)" <- w766
    n418 = Equal?(x="Tab Control 6", y=T22."High Res Display") -> (x = y?=w794:bool)
    n419 = for {
      tunnel: [w2079] -> w911 mode=indexing
      tunnel: w912 -> [w2078]
      tunnel: "Trap Disp. Downsample" -> [w2075]
      tunnel: w791 -> [w2073] mode=indexing
      tunnel: w768 -> [w2072]
      tunnel: w789 -> [w2071] mode=indexing
      tunnel: w790 -> [w2070]
      tunnel: [w2069] -> w740 mode=indexing
      tunnel: w766 -> [w2068]
      workers-P: _ -> [_]
      n420 = Bundle By Name("Y"=w2073, "dt"=w2072) -> (w2074:waveform(dbl))  [unwired: 1 out]
      n421 = Set Waveform Attribute(5:w2071, 6:w2070, 7:w2074) -> (3:w2069:waveform(dbl))  [unwired: 1 in, 2 out]
      n422 = call "downsample 1D array - double.vi"("Ave N"=w2075, "Array In"=w2073) -> ("Array Out"=w2076:dbl[])  [unwired: 1 out]
      n423 = To Time Stamp(1:w2078) -> (0:w2077:timestamp)
      n424 = Bundle By Name(cluster=w2069, "t0"=w2077, "Y"=w2076, "dt"=w2068) -> (w2079:waveform(dbl))
    }
    n425 = case "For plotting results of scanning MCL" shown="True" w881 {
      tunnel: w880 -> [_ w1517]
      tunnel: w782 -> [_ w1613]
      tunnel: w889 -> [_ _]
      tunnel: w740 -> [_ w1587]
      tunnel: w715 -> [_ w1518]
      tunnel: w714 -> [_ w1491]
      frame #0 {
      }
      frame #1 {
        w1498 = u32 0 items=["Horizontal", "Vertical", "Central", "1st Diagonal", "2nd Diagonal"] ("Type of Symmetry")
        w1526 = u32 0 items=["Horizontal", "Vertical", "Central", "1st Diagonal", "2nd Diagonal"] ("Type of Symmetry")
        w1529 = u32 0 items=["Horizontal", "Vertical", "Central", "1st Diagonal", "2nd Diagonal"] ("Type of Symmetry")
        w1558 = u32 0 items=["Horizontal", "Vertical", "Central", "1st Diagonal", "2nd Diagonal"] ("Type of Symmetry")
        n426 = Index Array(array=w1587, index=10) -> (element=w1593:waveform(dbl))
        n427 = Index Array(array=w1587, index=11) -> (element=w1590:waveform(dbl))
        n428 = Index Array(array=w1587, index="Channel") -> (element=w1589:waveform(dbl))
        n429 = local read "Cycles/step (MCL)"() -> (w1543:u64)
        n430 = Unbundle(w1491) -> ("New Image"=w1490:T2, "New Image"=w1489:T2, "New Image"=w1488:T2, "New Image"=w1487:T2)
        n431 = Unbundle By Name(w1593) -> ("Y"=w1545:dbl[])
        n432 = Unbundle By Name(w1590) -> ("Y"=w1547:dbl[])
        n433 = Unbundle By Name(w1589) -> ("Y"=w1552:dbl[])
        n434 = call "downsample 1D array - double.vi"("Ave N"=w1543, "Array In"=w1545) -> ("Array Out"=w1544:dbl[])  [unwired: 1 out]
        n435 = call "downsample 1D array - double.vi"("Ave N"=w1543, "Array In"=w1547) -> ("Array Out"=w1546:dbl[])  [unwired: 1 out]
        n436 = call "downsample 1D array - double.vi"("Ave N"=w1543, "Array In"=w1552) -> ("Array Out"=w1551:dbl[])  [unwired: 1 out]
        n437 = feedback #5(w1613) -> (w1614:dbl[])
        n438 = Build Array (concatenate)(w1614, w1613) -> (w1595:dbl[])
        n439 = feedback #6(w1518) -> (w1520:dbl[])
        n440 = Build Array (concatenate)(w1520, w1518) -> (w1519:dbl[])
        n441 = Select(t=w1613, s=w1517, f=w1595) -> (s? t:f=w1599:dbl[])
        n442 = local read "Scan steps (MCL)"() -> (w1500:u64)
        n443 = Select(t=w1518, s=w1517, f=w1519) -> (s? t:f=w1501:dbl[])
        n444 = local read "Scan lines (y)"() -> (w1486:u64)
        n445 = local read "N APD Samp/step"() -> (w1502:dbl)
        n446 = feedback #7(w1544) -> (w1601:dbl[])
        n447 = Build Array (concatenate)(w1601, w1544) -> (w1592:dbl[])
        n448 = feedback #8(w1551) -> (w1611:dbl[])
        n449 = Build Array (concatenate)(w1611, w1551) -> (w1610:dbl[])
        n450 = feedback #9(w1546) -> (w1603:dbl[])
        n451 = Build Array (concatenate)(w1603, w1546) -> (w1604:dbl[])
        n452 = Select(t=w1544, s=w1517, f=w1592) -> (s? t:f=w1548:dbl[])
        n453 = Select(t=w1551, s=w1517, f=w1610) -> (s? t:f=w1550:dbl[])
        n454 = Select(t=w1546, s=w1517, f=w1604) -> (s? t:f=w1549:dbl[])
        n455 = Multiply(x=w1500, y=u64 2) -> (x*y=w1485:u64)
        n456 = call "integrate 1D array interval - double.vi"("Ave N"=w1502, "Array In"=w1501) -> ("Array Out"=w1513:dbl[])  [unwired: 1 out]
        n457 = call "integrate 1D array interval - double.vi"("Ave N"=w1502, "Array In"=w1599) -> ("Array Out"=w1598:dbl[])  [unwired: 1 out]
        n458 = Array Size(array=w1513) -> (size(s)=w1514:i32)
        n459 = Array Size(array=w1598) -> (size(s)=w1600:i32)
        n460 = Multiply(x=w1486, y=w1485) -> (x*y=w1516:u64)
        n461 = Multiply(x=w1486, y=w1485) -> (x*y=w1608:u64)
        n462 = call <vilib>:"Mean.vi"("X"=w1548) -> ("mean"=w1532:dbl)  [unwired: 1 out]
        n463 = Subtract(x=w1516, y=w1514) -> (x-y=w1507:u64)
        n464 = call <vilib>:"Mean.vi"("X"=w1550) -> ("mean"=w1537:dbl)  [unwired: 1 out]
        n465 = call <vilib>:"Mean.vi"("X"=w1549) -> ("mean"=w1535:dbl)  [unwired: 1 out]
        n466 = call <vilib>:"Mean.vi"("X"=w1513) -> ("mean"=w1504:dbl)  [unwired: 1 out]
        n467 = Subtract(x=w1608, y=w1600) -> (x-y=w1542:u64)
        n468 = call <vilib>:"Mean.vi"("X"=w1598) -> ("mean"=w1539:dbl)  [unwired: 1 out]
        n469 = Initialize Array(1.0 ("element"), w1507) -> (w1503:dbl[])
        n470 = Initialize Array(1.0 ("element"), w1542) -> (w1533:dbl[])
        n471 = Multiply(x=w1503, y=w1504) -> (x*y=w1505:dbl[])
        n472 = Multiply(x=w1533, y=w1535) -> (x*y=w1536:dbl[])
        n473 = Multiply(x=w1533, y=w1537) -> (x*y=w1538:dbl[])
        n474 = Multiply(x=w1533, y=w1532) -> (x*y=w1534:dbl[])
        n475 = Multiply(x=w1533, y=w1539) -> (x*y=w1540:dbl[])
        n476 = Build Array (concatenate)(w1548, w1534) -> (w1602:dbl[])
        n477 = Build Array (concatenate)(w1550, w1538) -> (w1606:dbl[])
        n478 = Build Array (concatenate)(w1549, w1536) -> (w1605:dbl[])
        n479 = Build Array (concatenate)(w1513, w1505) -> (w1515:dbl[])
        n480 = Build Array (concatenate)(w1598, w1540) -> (w1607:dbl[])
        n481 = Reshape Array(w1602, w1486, w1485) -> (w1568:dbl[][])
        n482 = Reshape Array(w1515, w1486, w1485) -> (w1511:dbl[][])
        n483 = Reshape Array(w1606, w1486, w1485) -> (w1560:dbl[][])
        n484 = Reshape Array(w1605, w1486, w1485) -> (w1575:dbl[][])
        n485 = Reshape Array(w1607, w1486, w1485) -> (w1585:dbl[][])
        n486 = Array Subset(array=w1575, index (col)=0 ("index"), length (col)=w1500) -> (w1580:dbl[][])  [unwired: 2 in]
        n487 = Array Subset(array=w1575, index (col)=w1500) -> (w1578:dbl[][])  [unwired: 3 in]
        n488 = Array Subset(array=w1560, index (col)=0 ("index"), length (col)=w1500) -> (w1566:dbl[][])  [unwired: 2 in]
        n489 = Array Subset(array=w1560, index (col)=w1500) -> (w1564:dbl[][])  [unwired: 3 in]
        n490 = Array Subset(array=w1511, index (col)=0 ("index"), length (col)=w1500) -> (w1510:dbl[][])  [unwired: 2 in]
        n491 = Array Subset(array=w1511, index (col)=w1500) -> (w1508:dbl[][])  [unwired: 3 in]
        n492 = Array Subset(array=w1585, index (col)=0 ("index"), length (col)=w1500) -> (w1584:dbl[][])  [unwired: 2 in]
        n493 = Array Subset(array=w1585, index (col)=w1500) -> (w1582:dbl[][])  [unwired: 3 in]
        n494 = Array Subset(array=w1568, index (col)=0 ("index"), length (col)=w1500) -> (w1573:dbl[][])  [unwired: 2 in]
        n495 = Array Subset(array=w1568, index (col)=w1500) -> (w1571:dbl[][])  [unwired: 3 in]
        n496 = for {
          tunnel: w1580 -> [w1622] mode=indexing
          tunnel: [w1621] -> w1579 mode=indexing
          workers-P: _ -> [_]
          n497 = Reverse 1D Array(array=w1622) -> (reversed array=w1621:dbl[])
        }
        n498 = for {
          tunnel: w1566 -> [w1618] mode=indexing
          tunnel: [w1617] -> w1565 mode=indexing
          workers-P: _ -> [_]
          n499 = Reverse 1D Array(array=w1618) -> (reversed array=w1617:dbl[])
        }
        n500 = for {
          tunnel: w1510 -> [w1616] mode=indexing
          tunnel: [w1615] -> w1509 mode=indexing
          workers-P: _ -> [_]
          n501 = Reverse 1D Array(array=w1616) -> (reversed array=w1615:dbl[])
        }
        n502 = for {
          tunnel: w1584 -> [w1624] mode=indexing
          tunnel: [w1623] -> w1583 mode=indexing
          workers-P: _ -> [_]
          n503 = Reverse 1D Array(array=w1624) -> (reversed array=w1623:dbl[])
        }
        n504 = for {
          tunnel: w1573 -> [w1620] mode=indexing
          tunnel: [w1619] -> w1572 mode=indexing
          workers-P: _ -> [_]
          n505 = Reverse 1D Array(array=w1620) -> (reversed array=w1619:dbl[])
        }
        n506 = Index Array(array=w1585, index (row)=0) -> (element=→"Waveform Graph":dbl[])  [unwired: 1 in]
        n507 = Add(x=w1579, y=w1578) -> (x+y=w1577:dbl[][])
        n508 = Add(x=w1565, y=w1564) -> (x+y=w1563:dbl[][])
        n509 = Add(x=w1509, y=w1508) -> (x+y=w1493:dbl[][])
        n510 = Add(x=w1583, y=w1582) -> (x+y=w1557:dbl[][])
        n511 = Add(x=w1572, y=w1571) -> (x+y=w1570:dbl[][])
        n512 = Divide(x=w1563, y=2) -> (x/y=w1561:dbl[][])
        n513 = Divide(x=w1577, y=2) -> (x/y=w1522:dbl[][])
        n514 = Divide(x=w1570, y=2) -> (x/y=w1524:dbl[][])
        n515 = To Single Precision Float(number=w1557) -> (single precision float=w1556:sgl[][])
        n516 = Transpose 2D Array(2D array=w1561) -> (transposed array=→"Data map":dbl[][])
        n517 = To Single Precision Float(number=w1493) -> (single precision float=w1497:sgl[][])
        n518 = To Single Precision Float(number=w1522) -> (single precision float=w1528:sgl[][])
        n519 = To Single Precision Float(number=w1524) -> (single precision float=w1525:sgl[][])
        n520 = call "IMAQ ArrayToImage"("Image Pixels (Float)"=w1556, "Image"=w1490) -> ("Image Out"=w1559:T2)  [unwired: 8 in, 1 out]
        n521 = call "IMAQ ArrayToImage"("Image Pixels (Float)"=w1497, "Image"=w1489) -> ("Image Out"=w1499:T2)  [unwired: 8 in, 1 out]
        n522 = call "IMAQ ArrayToImage"("Image Pixels (Float)"=w1528, "Image"=w1488) -> ("Image Out"=w1530:T2)  [unwired: 8 in, 1 out]
        n523 = call "IMAQ ArrayToImage"("Image Pixels (Float)"=w1525, "Image"=w1487) -> ("Image Out"=w1527:T2)  [unwired: 8 in, 1 out]
        n524 = call "IMAQ Symmetry"("Type of Symmetry"=w1558, "Image Src"=w1559) -> ("Image Dst Out"=w1554:T2)  [unwired: 3 in, 1 out]
        n525 = call "IMAQ Symmetry"("Type of Symmetry"=w1498, "Image Src"=w1499) -> ("Image Dst Out"=w1495:T2)  [unwired: 3 in, 1 out]
        n526 = call "IMAQ Symmetry"("Type of Symmetry"=w1529, "Image Src"=w1530) -> ("Image Dst Out"=→"Detection Laser X":T2)  [unwired: 3 in, 1 out]
        n527 = call "IMAQ Symmetry"("Type of Symmetry"=w1526, "Image Src"=w1527) -> ("Image Dst Out"=→"Detection Laser Y":T2)  [unwired: 3 in, 1 out]
        n528 = call "IMAQ Set Simple Calibration"("Calibration Axis Info"=T23 {"Origin Pixel"={"X"=0.0, "Y"=0.0}, "Angle Relative to Horizontal (deg)"=0.0, "Axis Reference"=0}, "Grid Descriptor"=T24 {"X Step"=0.3, "Y Step"=0.3, "Unit"=enum."Undefined"}, "Image"=w1554) -> ("Calibrated Image"=→"APD 1":T2)  [unwired: 7 in, 1 out]
        n529 = call "IMAQ Set Simple Calibration"("Calibration Axis Info"=T23 {"Origin Pixel"={"X"=0.0, "Y"=0.0}, "Angle Relative to Horizontal (deg)"=0.0, "Axis Reference"=0}, "Grid Descriptor"=T24 {"X Step"=0.3, "Y Step"=0.3, "Unit"=enum."Undefined"}, "Image"=w1495) -> ("Calibrated Image"=→"APD 2":T2)  [unwired: 7 in, 1 out]
      }
    }
    n530 = Reciprocal(x=w766) -> (1/x=→"Trap Disp. Freq. (Hz)":dbl)
    n531 = case shown="True" w794 {
      tunnel: w740 -> [_ w1045]
      frame #0 {
      }
      frame #1 {
        n532 = Index Array(array=w1045, index="High Res. Display") -> (element=w1046:waveform(dbl))
        n533 = call <vilib>:"Std Deviation and Variance.vi"("X"=w1046) -> ("mean"=w1053:dbl, "standard deviation"=w1058:dbl)  [unwired: 1 in, 1 out]
        "Mean Intensity" <- w1053
        "Sigma" <- w1058
        n534 = Subtract(x=w1046, y=w1053) -> (x-y=w1052:waveform(dbl))
        n535 = Select(t=w1052, s="Subtract mean", f=w1046) -> (s? t:f=→"1 Channel":waveform(dbl))
        n536 = Divide(x=w1058, y=w1053) -> (x/y=→"Sigma/Mean":dbl)
        n537 = feedback #10(1) -> (w1047:i32)
        n538 = Greater Or Equal?(x=w1047, y="Slow mean N ave.") -> (x >= y?=w1060:bool)
        n539 = Increment(x=w1047) -> (x+1=w1062:i32)
        n540 = Select(t=1, s=w1060, f=w1062) -> (s? t:f=w1049:i32)
        n541 = feedback #11() -> (w1050:waveform(dbl))  [unwired: 1 out]
        n542 = case shown="Default" w1047 {
          tunnel: [w1065 w1068] -> w1051
          tunnel: w1050 -> [w1067 _]
          tunnel: w1046 -> [w1066 w1068]
          frame #0 {
            n543 = call-poly <vilib>:"Append Waveforms.vi"("waveform B"=w1066, "waveform A"=w1067) -> ("waveform out"=w1065:waveform(dbl))  [unwired: 1 in, 8 out]
          }
          frame #1 {
          }
        }
        n544 = case shown="True" w1060 {
          tunnel: w1051 -> [_ w1064]
          frame #0 {
          }
          frame #1 {
            n545 = call <vilib>:"Mean.vi"("X"=w1064) -> ("mean"=→"Slow mean":dbl)  [unwired: 1 out]
          }
        }
      }
    }
    n546 = case "For computing FFTs for display" shown="True" "Compute FFT" {
      tunnel: w740 -> [_ w2964]
      frame #0 {
      }
      frame #1 {
        n547 = Build Array("FFT 1 Choice 1", "FFT 1 Choice 2", "FFT 2 Choice 1", "FFT 2 Choice 2") -> (w2957:u16[])
        n548 = Array Size(array=w2964) -> (size(s)=w2963:i32)
        n549 = feedback #12(u16[] [100, 100, 100, 100]) -> (w2958:u16[])
        n550 = feedback #13("# Spectra to Ave.") -> (w2955:dbl)
        n551 = Not Equal?(x="# Spectra to Ave.", y=w2955) -> (x != y?=w2954:bool)
        n552 = Not Equal?(x=w2957, y=w2958) -> (x != y?=w2956:bool)
        n553 = feedback #14(1.0) -> (w2941:dbl)
        n554 = Compound Arithmetic op=OR("Reset FFT", w2956, w2954) -> (w2939:bool)
        n555 = Select(t=1.0, s=w2939, f=w2941) -> (s? t:f=w2943:dbl)
        n556 = Greater?(x=w2943, y="# Spectra to Ave.") -> (0:w2962:bool)
        n557 = Increment(x=w2943) -> (x+1=w2942:dbl)
        n558 = local read "DMA Update Period (s)"() -> (w2937:dbl)
        n559 = Multiply(x="# Spectra to Ave.", y=w2937) -> (x*y=→"Ave. Time (s)":dbl)
        n560 = Build Array(cluster{"f0":dbl, "df":dbl, "magnitude":dbl[]} {"f0"=0.0, "df"=0.0, "magnitude"=[]} ("PSD")) -> (w2946:cluster{"f0":dbl, "df":dbl, "magnitude":dbl[]}[])
        n561 = Build Array(w2946, w2946, w2946, w2946) -> (w2948:T35)
        n562 = feedback #15(w2948) -> (w2953:T35)
        n563 = for {
          N: 4 -> [_]
          tunnel: w2957 -> [w2986] mode=indexing
          tunnel: w2964 -> [w2987]
          tunnel: w2963 -> [w2989]
          tunnel: w2939 -> [w2982]
          tunnel: w2962 -> [w2981]
          tunnel: "# Spectra to Ave." -> [w2980]
          tunnel: [w2979] -> w2952 mode=indexing
          tunnel: w2953 -> [w2984] mode=indexing
          tunnel: [w2983] -> w2940 mode=indexing
          tunnel: w2943 -> [w2978]
          n564 = Less?(x=w2986, y=w2989) -> (x < y?=w2988:bool)
          n565 = Index Array(array=w2987, index=w2986) -> (element=w2985:waveform(dbl))
          n566 = case shown="True" w2988 {
            tunnel: w2985 -> [_ w3006]
            tunnel: w2984 -> [w2991 w3004]
            tunnel: [w2991 w2992] -> w2983
            tunnel: w2982 -> [_ w3003]
            tunnel: w2981 -> [_ w2996]
            tunnel: w2980 -> [_ w2995]
            tunnel: [cluster{"f0":dbl, "df":dbl, "magnitude":dbl[]} {"f0"=0.0, "df"=0.0, "magnitude"=[]} ("PSD") w2997] -> w2979
            tunnel: w2978 -> [_ w2994]
            frame #0 {
            }
            frame #1 {
              n567 = call <vilib>:"Std Deviation and Variance.vi"("X"=w3006) -> ("mean"=w3007:dbl)  [unwired: 1 in, 2 out]
              n568 = Subtract(x=w3006, y=w3007) -> (x-y=w3005:waveform(dbl))
              n569 = xnode "Spectral Measurements"("Signals"=w3005) -> ("PSD"=w2999:cluster{"f0":dbl, "df":dbl, "magnitude":dbl[]})  [unwired: 1 in, 1 out]
              n570 = case shown="False" w3003 {
                tunnel: w3004 -> [w3016 _]
                tunnel: [w3012 w3021] -> w2992
                tunnel: w2999 -> [w3015 w3022]
                tunnel: w2996 -> [w3014 _]
                frame #0 {
                  n571 = Build Array (concatenate)(w3016, w3015) -> (w3013:cluster{"f0":dbl, "df":dbl, "magnitude":dbl[]}[])
                  n572 = case shown="True" w3014 {
                    tunnel: w3013 -> [w3017 w3020]
                    tunnel: [w3017 w3018] -> w3012
                    frame #0 {
                    }
                    frame #1 {
                      n573 = Delete From Array(array=w3020, index=0) -> (array with subset deleted=w3018:cluster{"f0":dbl, "df":dbl, "magnitude":dbl[]}[])  [unwired: 1 in, 1 out]
                    }
                  }
                }
                frame #1 {
                  n574 = Build Array(w3022) -> (w3021:cluster{"f0":dbl, "df":dbl, "magnitude":dbl[]}[])
                }
              }
              n575 = for {
                tunnel: w2992 -> [w3011] mode=indexing
                tunnel: [w3010] -> w3002 mode=indexing
                workers-P: _ -> [_]
                n576 = Unbundle By Name(w3011) -> ("magnitude"=w3010:dbl[])
              }
              n577 = Transpose 2D Array(2D array=w3002) -> (transposed array=w3001:dbl[][])
              n578 = for {
                tunnel: w3001 -> [w3009] mode=indexing
                tunnel: [w3008] -> w3000 mode=indexing
                workers-P: _ -> [_]
                n579 = Add Array Elements(numeric array=w3009) -> (sum=w3008:dbl)
              }
              n580 = Select(t=w2995, s=w2996, f=w2994) -> (s? t:f=w2993:dbl)
              n581 = Divide(x=w3000, y=w2993) -> (x/y=w2998:dbl[])
              n582 = Bundle By Name(cluster=w2999, "magnitude"=w2998) -> (w2997:cluster{"f0":dbl, "df":dbl, "magnitude":dbl[]})
            }
          }
        }
        n583 = case shown="True" w2939 {
          tunnel: w2940 -> [w2971 w2977]
          tunnel: [w2971 w2972] -> w2938
          frame #0 {
          }
          frame #1 {
            n584 = Array Subset(array=w2977, index (row)=0 ("index"), length (row)=4 ("length"), index (col)=0 ("index"), length (col)=1 ("length")) -> (w2972:T35)
          }
        }
        n585 = Split 1D Array(array=w2952, index=2) -> (first subarray=→"FFT 1":cluster{"f0":dbl, "df":dbl, "magnitude":dbl[]}[], second subarray=→"FFT 2":cluster{"f0":dbl, "df":dbl, "magnitude":dbl[]}[])
      }
    }
    n586 = Bundle("APD 1", "APD 2") -> (w910:cluster{string, string})  [unwired: 1 out]
    n587 = Cluster To Array(cluster=w910) -> (array=w907:string[])
    n588 = for {
      tunnel: w878 -> [w1999] mode=indexing
      tunnel: w912 -> [w2008]
      tunnel: w729 -> [w2007]
      tunnel: [w2003] -> w736 mode=indexing
      tunnel: "APD Disp. Scale" -> [w2004]
      tunnel: w790 -> [w2002]
      tunnel: w907 -> [w2001] mode=indexing
      tunnel: "APD Disp. Downsample" -> [w1997]
      tunnel: [w2000] -> w906
      workers-P: _ -> [_]
      n589 = call "integrate 1D array interval - double.vi"("Ave N"=w1997, "Array In"=w1999) -> ("Array Out"=w1998:dbl[])  [unwired: 1 out]
      n590 = Multiply(x=w2007, y=w1997) -> (x*y=w2000:dbl)
      n591 = Divide(x=w1998, y=w2004) -> (x/y=w2005:dbl[])
      n592 = To Time Stamp(1:w2008) -> (0:w2009:timestamp)
      n593 = Bundle By Name("t0"=w2009, "Y"=w2005, "dt"=w2000) -> (w2006:waveform(dbl))  [unwired: 1 out]
      n594 = Set Waveform Attribute(5:w2001, 6:w2002, 7:w2006) -> (3:w2003:waveform(dbl))  [unwired: 1 in, 2 out]
    }
    "APD Display Period (s)" <- w906
    n595 = Reciprocal(x=w906) -> (1/x=→"APD Display Freq. (Hz)":dbl)
    n596 = feedback #16(w783) -> (w876:u32[])
    n597 = Build Array (concatenate)(w876, w783) -> (w873:u32[])
    n598 = feedback #17(w716) -> (w735:u32[])
    n599 = Build Array (concatenate)(w735, w716) -> (w734:u32[])
    n600 = Array Size(array=w873) -> (size(s)=w870:i32)
    n601 = Array Size(array=w783) -> (size(s)=w872:i32)
    n602 = local read "APD Integration Time (s)"() -> (w743:dbl)
    n603 = Build Array (concatenate)(w736, w911) -> (w738:waveform(dbl)[])
    "All Signals" <- w738
    n604 = Multiply(x=w872, y="APD Ave N") -> (x*y=w871:dbl)
    n605 = Greater?(x=w870, y=w871) -> (0:w874:bool)
    n606 = case shown="True" w874 {
      tunnel: w873 -> [w1477 w1484]
      tunnel: [w1477 w1482] -> w814
      tunnel: w871 -> [_ w1479]
      tunnel: w870 -> [_ w1483]
      tunnel: w734 -> [w1476 w1481]
      tunnel: [w1476 w1478] -> w731
      frame #0 {
      }
      frame #1 {
        n607 = Subtract(x=w1483, y=w1479) -> (x-y=w1480:dbl)
        n608 = Array Subset(array=w1484, index=w1480, length=w1479) -> (w1482:u32[])
        n609 = Array Subset(array=w1481, index=w1480, length=w1479) -> (w1478:u32[])
      }
    }
    n610 = Multiply(x="APD Disp. Scale", y=w736) -> (x*y=w745:waveform(dbl)[])
    n611 = Multiply(x="APD Disp. Downsample", y=w743) -> (x*y=w741:dbl)
    n612 = Divide(x=w745, y=w741) -> (x/y=w713:waveform(dbl)[])
    n613 = Index Array(array=w713, index=0) -> (element=w723:waveform(dbl))
    n614 = Index Array(array=w713, index=1) -> (element=w721:waveform(dbl))
    n615 = Subtract(x=w721, y="APD 2 Offset") -> (x-y=w718:waveform(dbl))
    n616 = Subtract(x=w723, y="APD 1 Offset") -> (x-y=w719:waveform(dbl))
    n617 = Index Array(array=w738, index=3) -> (element=w825:waveform(dbl))
    n618 = Index Array(array=w738, index=6) -> (element=w822:waveform(dbl))
    n619 = Build Array(w719, w718) -> (→"APD Chart":waveform(dbl)[])
    n620 = Array Size(array=w814) -> (size(s)=w869:i32)
    n621 = call <vilib>:"Std Deviation and Variance.vi"("X"=w731) -> ("standard deviation"=w730:dbl)  [unwired: 1 in, 2 out]
    n622 = Add Array Elements(numeric array=w731) -> (sum=w733:u32)
    n623 = Add Array Elements(numeric array=w814) -> (sum=w879:u32)
    n624 = call <vilib>:"Std Deviation and Variance.vi"("X"=w814) -> ("standard deviation"=w813:dbl)  [unwired: 1 in, 2 out]
    n625 = Divide(x="T1 offset_x (mV)", y=1000.0) -> (x/y=w826:dbl)
    n626 = Divide(x=w730, y=w729) -> (x/y=w726:dbl)
    "Rate sigma (Hz) 2" <- w726
    n627 = Multiply(x=w729, y=w869) -> (x*y=w732:dbl)
    "Int. Time (s)" <- w732
    n628 = Divide(x=w733, y=w732) -> (x/y=w727:dbl)
    "APD 2 Rate (Hz)" <- w727
    n629 = Divide(x=w879, y=w732) -> (x/y=w811:dbl)
    "APD 1 Rate (Hz)" <- w811
    n630 = Divide(x=w813, y=w729) -> (x/y=w812:dbl)
    "Rate sigma (Hz)" <- w812
    n631 = Divide(x=w726, y=w727) -> (x/y=→"Sigma/Mean 2":dbl)
    n632 = Divide(x=w812, y=w811) -> (x/y=→"Sigma/Mean":dbl)
    n633 = Divide(x="T2 offset_x (mV)", y=1000.0) -> (x/y=w824:dbl)
    n634 = case shown="0, Default" "Calibration" {
      tunnel: "T1 alpha_x (nm/V)" -> [_ w1453 w1474]
      tunnel: "T1 kappa_x (pN/nm)" -> [_ _ w1464]
      tunnel: "T2 alpha_x (nm/V)" -> [_ w1452 w1472]
      tunnel: "T2 kappa_x (pN/nm)" -> [_ _ w1465]
      tunnel: w825 -> [w1435 w1450 w1470]
      tunnel: w822 -> [w1434 w1448 w1468]
      tunnel: [w1435 w1447 w1467] -> w855
      tunnel: [w1434 w1446 w1466] -> w854
      tunnel: ["T1 X (V)" ("Label.Text") "T1 X (nm)" ("Label.Text") "T1 X (pN)" ("Label.Text")] -> w843
      tunnel: ["T2 X (V)" ("Label.Text") "T2 X (nm)" ("Label.Text") "T2 X (pN)" ("Label.Text")] -> w842
      tunnel: ["Position (V)" ("Label.Text") "Position (nm)" ("Label.Text") "Force (pN)" ("Label.Text")] -> w844
      tunnel: w824 -> [_ w1438 w1457]
      tunnel: w826 -> [_ w1441 w1459]
      tunnel: ["Mean (V)" ("Label.Text") "Mean (nm)" ("Label.Text") "Mean (pN)" ("Label.Text")] -> w839
      tunnel: ["Difference (V)" ("Label.Text") "Difference (nm)" ("Label.Text") "Difference (pN)" ("Label.Text")] -> w746
      frame #0 {
      }
      frame #1 {
        n635 = Unbundle By Name(w1450) -> ("Y"=w1454:dbl[])
        n636 = Unbundle By Name(w1448) -> ("Y"=w1439:dbl[])
        n637 = Subtract(x=w1454, y=w1441) -> (x-y=w1442:dbl[])
        n638 = Subtract(x=w1439, y=w1438) -> (x-y=w1440:dbl[])
        n639 = Multiply(x=w1440, y=w1452) -> (x*y=w1449:dbl[])
        n640 = Multiply(x=w1453, y=w1442) -> (x*y=w1451:dbl[])
        n641 = Bundle By Name(cluster=w1448, "Y"=w1449) -> (w1446:waveform(dbl))
        n642 = Bundle By Name(cluster=w1450, "Y"=w1451) -> (w1447:waveform(dbl))
      }
      frame #2 {
        n643 = Unbundle By Name(w1470) -> ("Y"=w1475:dbl[])
        n644 = Unbundle By Name(w1468) -> ("Y"=w1473:dbl[])
        n645 = Subtract(x=w1473, y=w1457) -> (x-y=w1458:dbl[])
        n646 = Subtract(x=w1475, y=w1459) -> (x-y=w1460:dbl[])
        n647 = Compound Arithmetic op=MULTIPLY(w1458, w1472, w1465) -> (w1469:dbl[])
        n648 = Compound Arithmetic op=MULTIPLY(w1464, w1474, w1460) -> (w1471:dbl[])
        n649 = Bundle By Name(cluster=w1468, "Y"=w1469) -> (w1466:waveform(dbl))
        n650 = Bundle By Name(cluster=w1470, "Y"=w1471) -> (w1467:waveform(dbl))
      }
    }
    n651 = feedback #18(u16 1 ("Calibration")) -> (w846:u16)
    n652 = case shown="True" "Read Lateness and Rel Phase" {
      tunnel: w787 -> [w1078 w1098]
      tunnel: w786 -> [w1079 w1097]
      tunnel: [w1078 w1096] -> w817
      tunnel: [w1079 w1095] -> w816
      frame #0 {
      }
      frame #1 {
        n653 = xnode "Read/Write Control"("FPGA VI Reference In"=w1098, "error in"=w1097) -> ("FPGA VI Reference Out"=w1096:T15, "error out"=w1095:errorcluster, "GI Relative phase"=→"GI relative phase":i16, "Relative phase"=→"Relative phase (AI1)":i16, "AI Late Counter"=→"Late Counter (AI1)":u32, "GI Late Counter"=→"GI Late Counter":u32, "MCL Late Counter"=→"MCL Late Counter":u32, "MCL Relative Phase"=→"Relative Phase (MCL)":i16, "APD Acq Relative Phase"=→"APD Acq Relative Phase":i16, "APD 1 Gate Relative Phase"=→"APD 1 Gate Relative Phase":i16, "APD 2 Gate Relative Phase"=→"APD 2 Gate Relative Phase":i16, "APD Acq Late Counter"=→"APD Acq Late Counter":u32, "APD 1 Gate Late Counter"=→"APD 1 Gate Late Counter":u32, "APD 2 Gate Late Counter"=→"APD 2 Gate Late Counter":u32, "Green FB Relative Phase"=→"Relative phase (Green FB)":i16, "GI Relative phase 2"=→"GI relative phase 2":i16, "GI Late Counter 2"=→"GI Late Counter 2":u32)
      }
    }
    n654 = Not Equal?(x=w846, y="Calibration") -> (x != y?=w792:bool)
    n655 = Unbundle By Name(w825) -> ("Y"=w828:dbl[])
    n656 = Unbundle By Name(w822) -> ("Y"=w831:dbl[])
    n657 = Subtract(x=w828, y=w826) -> (x-y=w829:dbl[])
    n658 = Subtract(x=w831, y=w824) -> (x-y=w830:dbl[])
    n659 = Multiply(x=w830, y="T2 alpha_x (nm/V)") -> (x*y=w821:dbl[])
    n660 = Multiply(x="T1 alpha_x (nm/V)", y=w829) -> (x*y=w820:dbl[])
    n661 = Multiply(x=w854, y=-1.0) -> (x*y=w833:waveform(dbl))
    n662 = Subtract(x=w821, y=w820) -> (x-y=w819:dbl[])
    n663 = Unbundle By Name(w854) -> ("Y"=w774:dbl[])
    n664 = Unbundle By Name(w855) -> ("Y"=w775:dbl[])
    n665 = Build Array(w855, w833) -> (→"Force":waveform(dbl)[])
    n666 = Subtract(x=w819, y="Offset (nm)") -> (x-y=w772:dbl[])
    n667 = call <vilib>:"Mean.vi"("X"=w774) -> ("mean"=w750:dbl)  [unwired: 1 out]
    "T2 X" <- w750
    n668 = Absolute Value(x=w775) -> (abs(x)=w776:dbl[])
    n669 = Absolute Value(x=w774) -> (abs(x)=w777:dbl[])
    n670 = call <vilib>:"Mean.vi"("X"=w775) -> ("mean"=w751:dbl)  [unwired: 1 out]
    "T1 X" <- w751
    n671 = Add(x=w776, y=w777) -> (x+y=w778:dbl[])
    n672 = Bundle By Name(cluster=w825, "Y"=w772) -> (w737:waveform(dbl))
    "Bead Separation" <- w737
    n673 = Divide(x=w778, y=2.0) -> (x/y=→"Vec Mean of T1 T2":dbl[])
    n674 = case shown="True" w792 {
      tunnel: w844 -> [_ w1428]
      tunnel: w843 -> [_ w1427]
      tunnel: w842 -> [_ w1426]
      tunnel: w839 -> [_ w1425]
      tunnel: w746 -> [_ w1424]
      frame #0 {
      }
      frame #1 {
        n675 = property on="Force" class="WFChart (strict)"("YScale.NameLbl.Text"=w1428) -> ()  [unwired: 2 in, 2 out]
        n676 = property on="T2 X" class="DigNum (strict)"("Caption.Text"=w1426) -> ()  [unwired: 2 in, 2 out]
        n677 = property on="T1 X" class="DigNum (strict)"("Caption.Text"=w1427) -> ()  [unwired: 2 in, 2 out]
        n678 = property on="Mean" class="DigNum (strict)"("Caption.Text"=w1425) -> ()  [unwired: 2 in, 2 out]
        n679 = property on="Difference" class="DigNum (strict)"("Caption.Text"=w1424) -> ()  [unwired: 2 in, 2 out]
      }
    }
    n680 = local read "Tether"() -> (w781:bool)
    n681 = Absolute Value(x=w751) -> (abs(x)=w748:dbl)
    n682 = Absolute Value(x=w750) -> (abs(x)=w747:dbl)
    n683 = local read "Display Period (s)"() -> (w765:dbl)
    n684 = Add(x=w748, y=w747) -> (x+y=w841:dbl)
    n685 = Subtract(x=w748, y=w747) -> (x-y=→"Difference":dbl)
    n686 = feedback #19(w772) -> (w771:dbl[])
    n687 = Divide(x=w841, y=2.0) -> (x/y=w780:dbl)
    "Mean" <- w780
    n688 = case shown="True" w781 {
      tunnel: w780 -> [_ w1029]
      frame #0 {
      }
      frame #1 {
        n689 = Greater?(x="Lost Tether Alarm Threshold (pN)", y=w1029) -> (0:w1027:bool)
        n690 = case shown="True" w1027 {
          frame #0 {
          }
          frame #1 {
            n691 = flat-sequence {
              frame #0 {
                # "stop only if saving"
                n692 = local read "Saving..."() -> (w1041:bool)
                n693 = And(x=w1041, y="TA Cancel Save?") -> (x .and. y?=w1040:bool)
                n694 = local write "Stop Saving"(w1040) -> ()
              }
              frame #1 {
                n695 = case shown="True" "TA Green Off?" {
                  frame #0 {
                  }
                  frame #1 {
                    w1044 = FALSE ("Fl. Triggered...")
                    n696 = local write "Fl. Triggered..."(w1044) -> ()
                    n697 = property on="Green Laser ON/Interlacing" class="Bool (strict)"("Val(Sgnl)"=w1044) -> ()  [unwired: 2 in, 2 out]
                  }
                }
              }
            }
            n698 = local read "Time tether formed"() -> (w1035:timestamp)
            n699 = Get Date/Time In Seconds() -> (seconds since 1Jan1904=w1036:timestamp)
            n700 = Subtract(x=w1036, y=w1035) -> (x-y=w1034:dbl)
            n701 = Number To Decimal String(number=w1034) -> (decimal integer string=w1031:string)  [unwired: 1 out]
            n702 = local read "Messages"() -> (w1038:string)
            n703 = call <vilib>:"Beep.vi"() -> ()  [unwired: 3 in, 9 out]
            n704 = Concatenate Strings("Lost tether (" ("Message to add"), w1031, " s)." ("string")) -> (w1033:string)
            n705 = local write "Tether"(FALSE ("Tether")) -> ()
            n706 = call "Update messages.vi"("Message to add"=w1033, "Old message string"=w1038) -> ("New message string"=w1037:string)
            n707 = local write "Messages"(w1037) -> ()
          }
        }
      }
    }
    n708 = Build Array (concatenate)(w772, w771) -> (w770:dbl[])
    n709 = Divide(x="Bead Sep. Int. Time (s)", y=w765) -> (x/y=w764:dbl)
    n710 = Split 1D Array(array=w770, index=w764) -> (first subarray=w763:dbl[])  [unwired: 1 out]
    n711 = xnode "Read/Write Control"("FPGA VI Reference In"=w817, "error in"=w816) -> ("FPGA VI Reference Out"=w940:T15, "error out"=w934:errorcluster, "AI2 Y Sum Set 1"=w930:i16, "AI2 Y Sum Set 2"=w929:i16, "Scanning"=→"AOD Scanning":bool, "Scan I"=→"AOD Scan I":u64, "Scanning MCL"=w932:bool, "Scan I (MCL)"=→"MCL Scan I":u64, "Green FB Signals"=w864:T28)  [unwired: 1 out]
    "MCL Scanning" <- w932
    n712 = call <vilib>:"Mean.vi"("X"=w763) -> ("mean"=w762:dbl)  [unwired: 1 out]
    "Bead Mean (nm)" <- w762
    n713 = Subtract(x=w763, y=w762) -> (x-y=w761:dbl[])
    n714 = Square(x=w761) -> (x^2=w760:dbl[])
    n715 = call <vilib>:"Mean.vi"("X"=w760) -> ("mean"=w759:dbl)  [unwired: 1 out]
    n716 = Square Root(x=w759) -> (sqrt(x)=w758:dbl)
    n717 = Multiply(x=10.0, y=w758) -> (x*y=→"RMS (Ang)":dbl)
    n718 = flat-sequence "To save data" {
      tunnel: [w3405] -> w953
      tunnel: [w3406] -> w952
      tunnel: w895 -> [w3399]
      tunnel: w768 -> [w3403]
      tunnel: ["Save Calibration"] -> w921
      tunnel: w916 -> [w3402]
      tunnel: [w3395] -> w915
      tunnel: [w3392] -> w914
      tunnel: [w3389] -> w913
      tunnel: w894 -> [w3391]
      tunnel: w789 -> [w3385]
      tunnel: [w3385] -> w788
      tunnel: ["Start Saving"] -> w739
      tunnel: w953 -> [w3605]
      tunnel: w952 -> [w3604]
      tunnel: w951 -> [w3603]
      tunnel: w921 -> [w3602]
      tunnel: w915 -> [w3600]
      tunnel: w914 -> [w3599]
      tunnel: w913 -> [w3598]
      tunnel: w752 -> [w3597]
      tunnel: w809 -> [w3596]
      tunnel: w788 -> [w3595]
      tunnel: w739 -> [w3594]
      tunnel: w737 -> [w3593]
      tunnel: w713 -> [w3592]
      frame #0 {
        n719 = Or(x="Save N Sets", y="Start Saving") -> (x .or. y?=w3386:bool)
        n720 = To Double Precision Float(number=w3402) -> (double precision float=w3396:dbl)
        n721 = Build Array(w3386, "Save Calibration", w3399, w3391) -> (w3401:bool[])
        n722 = Compound Arithmetic op=OR("Save Calibration", w3399, w3386, w3391) -> (w3404:bool)
        n723 = Boolean Array To Number(Boolean array=w3401) -> (number=w3398:u32)
        n724 = feedback #20(refnum<k0> refnum) -> (w3407:refnum<file>)
        n725 = feedback #21(FALSE ("Save APD Data\nwith Trap Data")) -> (w3390:bool)
        n726 = feedback #22(refnum<k0> refnum) -> (w3393:refnum<file>)
        n727 = feedback #23(0) -> (w3409:i32)
        n728 = feedback #24() -> (w3397:u32)  [unwired: 1 out]
        n729 = case shown="True" w3404 {
          tunnel: [w3414 1] -> w3405
          tunnel: w3409 -> [w3416 _]
          tunnel: [w3415 w3429] -> w3406
          tunnel: w3407 -> [w3415 _]
          tunnel: w3403 -> [_ w3449]
          tunnel: w3396 -> [_ w3447]
          tunnel: w3398 -> [_ w3450]
          tunnel: [w3413 w3428] -> w3395
          tunnel: w3397 -> [w3413 _]
          tunnel: [w3412 w3425] -> w3392
          tunnel: w3393 -> [w3412 _]
          tunnel: [w3411 w3424] -> w3389
          tunnel: w3390 -> [w3411 _]
          tunnel: "Start Saving" -> [_ w3422]
          tunnel: w3385 -> [_ w3421]
          frame #0 {
            n730 = Increment(x=w3416) -> (x+1=w3414:i32)
          }
          frame #1 {
            w3417 = FALSE ("Start Saving")
            w3423 = 9.0  # File Version
            w3432 = FALSE ("prepend array or string size? (T)")
            w3430 = T30."big-endian, network order" ("byte order (0:big-endian, network order)")
            n731 = Array Size(array=w3421) -> (size(s)=w3420:i32)
            n732 = local read "BD 1 Frequency 1 (MHz)"() -> (w3446:dbl)
            n733 = local read "BD 2 Frequency 1 (MHz)"() -> (w3445:dbl)
            n734 = local read "BD 1 Frequency 2 (MHz)"() -> (w3444:dbl)
            n735 = local read "BD 2 Frequency 2 (MHz)"() -> (w3443:dbl)
            n736 = local read "BD 1 Frequency 3 (MHz)"() -> (w3442:dbl)
            n737 = local read "BD 2 Frequency 3 (MHz)"() -> (w3441:dbl)
            n738 = To Double Precision Float(number=w3420) -> (double precision float=w3419:dbl)
            n739 = local write "Save Calibration"(w3417) -> ()
            n740 = local write "Start Saving"(w3417) -> ()
            n741 = Build Array(w3446, w3445, w3444, w3443, w3442, w3441) -> (w3440:dbl[])
            n742 = case shown="1, Default" w3450 {
              tunnel: w3449 -> [w3498 w3518 w3533 w3570]
              tunnel: w3419 -> [w3503 w3525 w3553 w3589]
              tunnel: w3447 -> [w3502 w3524 w3552 w3588]
              tunnel: [w3499 w3520 w3544 w3580] -> w3438
              tunnel: [w3489 "Cal sets to save" w3534 w3571] -> w3428
              tunnel: w3440 -> [w3500 w3521 w3546 w3582]
              tunnel: "Save APD Data\nwith Trap Data" -> [w3497 _ w3529 w3567]
              tunnel: [w3497 w3514 w3529 w3567] -> w3424
              tunnel: w3423 -> [w3492 w3512 w3527 w3565]
              tunnel: w3422 -> [w3491 _ _ _]
              frame #0 {
                # "timeseries"
                n743 = case shown="True" "Profile" {
                  tunnel: [w3506 w3510] -> w3486
                  tunnel: [w3506 w3509] -> w3485
                  tunnel: [w3506 w3508] -> w3484
                  tunnel: [w3506 w3507] -> w3483
                  frame #0 {
                    w3506 = 0.0 ("f")
                  }
                  frame #1 {
                    n744 = local read "Current Position"() -> (w3511:cluster{dbl, dbl, dbl})
                    n745 = local read "Y change (mm)"() -> (w3507:dbl)
                    n746 = Unbundle(w3511) -> (w3510:dbl, w3509:dbl, w3508:dbl)
                  }
                }
                n747 = local read "Save ave N"() -> (w3505:dbl)
                n748 = Multiply(x=w3505, y=w3498) -> (x*y=w3504:dbl)
                n749 = Boolean To (0,1)(Boolean=w3497) -> (0, 1=w3496:i16)
                n750 = To Double Precision Float(number=w3496) -> (double precision float=w3495:dbl)
                n751 = Build Array(w3492, w3498, w3504, w3503, w3502, 0.0 ("f")) -> (w3501:dbl[])
                n752 = Build Array(w3495, w3486, w3485, w3484, w3483) -> (w3493:dbl[])
                n753 = Select(t=u32 4000000000, s=w3491, f="N sets to save") -> (s? t:f=w3489:u32)
                n754 = Build Array (concatenate)(w3501, w3500, w3493) -> (w3499:dbl[])
              }
              frame #1 {
                w3515 = 0.0 ("f")
                w3514 = FALSE ("Save APD Data\nwith Trap Data")
                # "calibration"
                n755 = Boolean To (0,1)(Boolean=w3514) -> (0, 1=w3517:i16)
                n756 = To Double Precision Float(number=w3517) -> (double precision float=w3516:dbl)
                n757 = Build Array(w3516, w3515, w3515, w3515, w3515) -> (w3513:dbl[])
                n758 = Build Array(w3512, w3518, w3518, w3525, w3524, 1.0 ("t")) -> (w3522:dbl[])
                n759 = Build Array (concatenate)(w3522, w3521, w3513) -> (w3520:dbl[])
                "Calibrating Trap..." <- TRUE ("Calibrating...")
              }
              frame #2 {
                w3530 = 0.0 ("f")
                # "scan dir (x/y = 0/1)"
                # "cycles/step"
                # "n scans (f/b)"
                # "steps"
                # "freq. range"
                # "AOD raster scan"
                n760 = local read "Number of F/B Scans (AOD)"() -> (w3538:u16)
                n761 = local read "Cycles/step (AOD)"() -> (w3540:u64)
                n762 = local read "Scan Range (MHz)"() -> (w3543:dbl)
                n763 = local read "Scan steps (AOD)"() -> (w3542:u64)
                n764 = local read "Scan BD"() -> (w3550:bool)
                n765 = local read "Save ave N"() -> (w3555:dbl)
                n766 = Boolean To (0,1)(Boolean=w3550) -> (0, 1=w3549:i16)
                n767 = To Double Precision Float(number=w3538) -> (double precision float=w3537:dbl)
                n768 = To Double Precision Float(number=w3542) -> (double precision float=w3541:dbl)
                n769 = To Double Precision Float(number=w3540) -> (double precision float=w3539:dbl)
                n770 = To Double Precision Float(number=w3549) -> (double precision float=w3548:dbl)
                n771 = Boolean To (0,1)(Boolean=w3529) -> (0, 1=w3532:i16)
                n772 = Multiply(x=w3555, y=w3533) -> (x*y=w3554:dbl)
                n773 = To Double Precision Float(number=w3532) -> (double precision float=w3531:dbl)
                n774 = Build Array(w3531, w3530, w3530, w3530, w3530) -> (w3528:dbl[])
                n775 = local read "N sets should be saved"() -> (w3535:dbl)
                n776 = Build Array(w3548, w3543, w3541, w3539, w3537) -> (w3545:dbl[])
                n777 = Build Array(w3527, w3533, w3554, w3553, w3552, 2.0 ("t")) -> (w3547:dbl[])
                n778 = Round Toward +Infinity(x=w3535) -> (ceil(x): smallest int >= x=w3536:dbl)
                n779 = Build Array (concatenate)(w3547, w3546, w3528, w3545) -> (w3544:dbl[])
                n780 = To Unsigned Long Integer(number=w3536) -> (unsigned 32bit integer=w3534:u32)
              }
              frame #3 {
                w3562 = 0.0 ("f")
                # "MCL raster scan"
                n781 = local read "Number of scans (MCL)"() -> (w3557:u64)
                n782 = local read "Scan lines (y)"() -> (w3556:u64)
                n783 = local read "2D or 1D Scan"() -> (w3559:bool)
                n784 = local read "Scan Range (V)\n(of steps)"() -> (w3579:dbl)
                n785 = local read "Fast Scan Dir"() -> (w3586:bool)
                n786 = local read "Cycles/step (MCL)"() -> (w3576:u64)
                n787 = local read "Scan steps (MCL)"() -> (w3578:u64)
                n788 = Select(t=w3556, s=w3559, f=w3557) -> (s? t:f=w3558:u64)
                n789 = Boolean To (0,1)(Boolean=w3559) -> (0, 1=w3561:i16)
                n790 = local read "Save ave N"() -> (w3591:dbl)
                n791 = local read "Initial X"() -> (w3564:dbl)
                n792 = local read "Initial Y"() -> (w3563:dbl)
                n793 = To Double Precision Float(number=w3561) -> (double precision float=w3560:dbl)
                n794 = Boolean To (0,1)(Boolean=w3586) -> (0, 1=w3585:i16)
                n795 = To Double Precision Float(number=w3558) -> (double precision float=w3574:dbl)
                n796 = To Double Precision Float(number=w3578) -> (double precision float=w3577:dbl)
                n797 = To Double Precision Float(number=w3576) -> (double precision float=w3575:dbl)
                n798 = To Double Precision Float(number=w3585) -> (double precision float=w3584:dbl)
                n799 = Boolean To (0,1)(Boolean=w3567) -> (0, 1=w3569:i16)
                n800 = Multiply(x=w3591, y=w3570) -> (x*y=w3590:dbl)
                n801 = To Double Precision Float(number=w3569) -> (double precision float=w3568:dbl)
                n802 = local read "N sets should be saved (MCL)"() -> (w3572:dbl)
                n803 = Build Array(w3568, w3560, w3562, w3562, w3562) -> (w3566:dbl[])
                n804 = Build Array(w3584, w3579, w3577, w3575, w3574, w3564, w3563) -> (w3581:dbl[])
                n805 = Build Array(w3565, w3570, w3590, w3589, w3588, 3.0 ("t")) -> (w3583:dbl[])
                n806 = Round Toward +Infinity(x=w3572) -> (ceil(x): smallest int >= x=w3573:dbl)
                n807 = Build Array (concatenate)(w3583, w3582, w3566, w3581) -> (w3580:dbl[])
                n808 = To Unsigned Long Integer(number=w3573) -> (unsigned 32bit integer=w3571:u32)
              }
            }
            n809 = local read "Index"() -> (w3455:dbl)
            n810 = call "Create new save file.vi"("Insert"="", "Ext"=".dat", "Index In"=w3455) -> ("Path Out"=w3426:path, "Index Out"=w3427:dbl)
            n811 = local write "Save file name"(w3426) -> ()
            n812 = local write "Index"(w3427) -> ()
            n813 = local write "Save index"(w3427) -> ()
            n814 = Array Size(array=w3438) -> (size(s)=w3439:i32)
            n815 = Open/Create/Replace File(file path (use dialog)=w3426, operation (0:open)=T29."create", access (0:read/write)=enum16{"read/write", "read-only", "write-only"}."write-only") -> (refnum out=w3452:refnum<file>)  [unwired: 1 in, 4 out]
            n816 = local write "Saving..."(TRUE ("Saving...")) -> ()
            n817 = To Double Precision Float(number=w3439) -> (double precision float=w3437:dbl)
            n818 = String Length(string="Comment (data description)") -> (length=w3435:i32)
            n819 = To Double Precision Float(number=w3435) -> (double precision float=w3434:dbl)
            n820 = Deny Access(7:w3452) -> (3:w3451:refnum<file>)  [unwired: 1 in, 2 out]
            n821 = Build Array (concatenate)(w3437, w3438, w3434) -> (w3436:dbl[])
            n822 = case "If fluorescence data to be saved" shown="True" w3424 {
              tunnel: w3426 -> [_ w3482]
              tunnel: [refnum<k0> refnum w3462] -> w3425
              frame #0 {
              }
              frame #1 {
                w3461 = 0.0
                n823 = local read "APD Integration Time (s)"() -> (w3467:dbl)
                n824 = local read "N APD Samp/step"() -> (w3460:dbl)
                n825 = Path To String(path=w3482) -> (string=w3481:string)
                n826 = String Length(string=w3481) -> (length=w3480:i32)
                n827 = Subtract(x=w3480, y=4) -> (x-y=w3478:i32)
                n828 = String Subset(string=w3481, length (rest)=w3478) -> (substring=w3477:string)  [unwired: 1 out]
                n829 = Build Array(w3467, w3460, w3461, w3461, w3461, w3461, w3461, w3461) -> (w3464:dbl[])
                n830 = Concatenate Strings(w3477, "_fl.dat" ("string")) -> (w3475:string)
                n831 = Array Size(array=w3464) -> (size(s)=w3466:i32)
                n832 = String To Path(string=w3475) -> (path=w3471:path)
                n833 = Open/Create/Replace File(file path (use dialog)=w3471, operation (0:open)=T29."create", access (0:read/write)=enum16{"read/write", "read-only", "write-only"}."write-only") -> (refnum out=w3472:refnum<file>)  [unwired: 1 in, 4 out]
                n834 = Deny Access(7:w3472) -> (3:w3468:refnum<file>)  [unwired: 1 in, 2 out]
                n835 = To Double Precision Float(number=w3466) -> (double precision float=w3465:dbl)
                n836 = Build Array (concatenate)(w3465, w3464) -> (w3463:dbl[])
                n837 = Write to Binary File(file (use dialog)=w3468, data=w3463, 5:FALSE ("prepend array or string size? (T)"), 9:T30."big-endian, network order" ("byte order (0:big-endian, network order)")) -> (refnum out=w3462:refnum<file>)  [unwired: 1 in, 3 out]
              }
            }
            n838 = Write to Binary File(file (use dialog)=w3451, data=w3436, 5:w3432, 9:w3430) -> (refnum out=w3433:refnum<file>)  [unwired: 1 in, 3 out]
            n839 = Write to Binary File(file (use dialog)=w3433, data="Comment (data description)", 5:w3432, 9:w3430) -> (refnum out=w3429:refnum<file>)  [unwired: 1 in, 3 out]
          }
        }
      }
      frame #1 {
        n840 = local read "Saving..."() -> (w3601:bool)
        n841 = case shown="True" w3601 {
          tunnel: w3605 -> [_ w3612]
          tunnel: w3604 -> [_ w3626]
          tunnel: w3603 -> [_ w3622]
          tunnel: w3602 -> [_ w3621]
          tunnel: w3600 -> [_ w3620]
          tunnel: w3599 -> [_ w3615]
          tunnel: w3598 -> [_ w3614]
          tunnel: w3597 -> [_ w3613]
          tunnel: w3596 -> [_ w3611]
          tunnel: w3595 -> [_ w3609]
          tunnel: w3594 -> [_ w3608]
          tunnel: w3593 -> [_ w3607]
          tunnel: w3592 -> [_ w3606]
          frame #0 {
          }
          frame #1 {
            n842 = Multiply(x=w3612, y=w3611) -> (x*y=→"Time (s)":dbl)
            n843 = Less Or Equal?(x=w3612, y=w3620) -> (x <= y?=w3624:bool)
            n844 = Or(x="Stop Saving", y="Abort save 2") -> (x .or. y?=w3616:bool)
            n845 = Not(x=w3616) -> (.not. x?=w3625:bool)
            n846 = And(x=w3624, y=w3625) -> (x .and. y?=w3623:bool)
            n847 = case shown="True" w3623 {
              tunnel: w3626 -> [w3631 w3694]
              tunnel: [0.0 w3697] -> w3619
              tunnel: w3612 -> [_ w3695]
              tunnel: w3620 -> [_ w3696]
              tunnel: w3622 -> [_ w3691]
              tunnel: w3621 -> [_ _]
              tunnel: w3615 -> [w3629 w3682]
              tunnel: w3614 -> [w3628 w3683]
              tunnel: w3613 -> [_ w3681]
              tunnel: w3609 -> [_ w3680]
              tunnel: w3608 -> [_ w3634]
              tunnel: w3607 -> [_ w3673]
              tunnel: w3606 -> [_ w3651]
              frame #0 {
                w3627 = FALSE
                n848 = Close File(refnum=w3631) -> ()  [unwired: 1 in, 2 out]
                n849 = case shown="True" w3628 {
                  tunnel: w3629 -> [_ w3632]
                  frame #0 {
                  }
                  frame #1 {
                    n850 = Close File(refnum=w3632) -> ()  [unwired: 1 in, 2 out]
                  }
                }
                n851 = local write "Raster Scanning..."(w3627) -> ()
                n852 = local write "Calibrating Trap..."(w3627) -> ()
                n853 = call <vilib>:"Beep.vi"() -> ()  [unwired: 3 in, 9 out]
                n854 = local write "Stop Saving"(w3627) -> ()
                "Saving..." <- w3627
              }
              frame #1 {
                n855 = local read "Calibrating Trap..."() -> (w3684:bool)
                n856 = case shown="True" w3683 {
                  tunnel: w3682 -> [_ w3701]
                  tunnel: w3681 -> [_ w3700]
                  frame #0 {
                  }
                  frame #1 {
                    n857 = Write to Binary File(file (use dialog)=w3701, data=w3700, 5:FALSE ("prepend array or string size? (T)"), 9:T30."big-endian, network order" ("byte order (0:big-endian, network order)")) -> ()  [unwired: 1 in, 4 out]
                  }
                }
                n858 = Greater?(x="Save ave N", y=1.0) -> (0:w3687:bool)
                n859 = Not(x=w3684) -> (.not. x?=w3686:bool)
                n860 = And(x=w3686, y=w3687) -> (x .and. y?=w3688:bool)
                n861 = case shown="True" w3688 {
                  tunnel: w3691 -> [w3704 w3716]
                  tunnel: [w3704 w3708] -> w3685
                  tunnel: "Save ave N" -> [_ w3709]
                  tunnel: w3680 -> [_ w3707]
                  frame #0 {
                  }
                  frame #1 {
                    n862 = Array Size(array=w3716) -> (size(s)=w3710:i32)
                    n863 = Array Size(array=w3707) -> (size(s)=w3706:i32)
                    n864 = Divide(x=w3710, y=w3706) -> (x/y=w3714:dbl)
                    n865 = Reshape Array(w3716, w3714, w3706) -> (w3715:i16[][])
                    n866 = Transpose 2D Array(2D array=w3715) -> (transposed array=w3713:i16[][])
                    n867 = for {
                      tunnel: w3713 -> [w3719] mode=indexing
                      tunnel: [w3718] -> w3705 mode=indexing
                      tunnel: w3709 -> [w3717]
                      workers-P: _ -> [_]
                      n868 = call "downsample 1D array - I16.vi"("Ave N"=w3717, "Array In"=w3719) -> ("Array Out"=w3718:i16[])  [unwired: 1 out]
                    }
                    n869 = Transpose 2D Array(2D array=w3705) -> (transposed array=w3712:i16[][])
                    n870 = Divide(x=w3710, y=w3709) -> (x/y=w3711:dbl)
                    n871 = Reshape Array(w3712, w3711) -> (w3708:i16[])
                  }
                }
                n872 = Index Array(array=w3651, index=1) -> (element=w3654:waveform(dbl))
                n873 = Index Array(array=w3651, index=0) -> (element=w3656:waveform(dbl))
                n874 = Unbundle By Name(w3654) -> ("Y"=w3658:dbl[])
                n875 = Unbundle By Name(w3656) -> ("Y"=w3666:dbl[])
                n876 = Write to Binary File(file (use dialog)=w3694, data=w3685, 5:FALSE ("prepend array or string size? (T)"), 9:T30."big-endian, network order" ("byte order (0:big-endian, network order)")) -> ()  [unwired: 1 in, 4 out]
                n877 = feedback #25(w3658) -> (w3660:dbl[])
                n878 = Build Array (concatenate)(w3660, w3658) -> (w3659:dbl[])
                n879 = Select(t=w3658, s=w3634, f=w3659) -> (s? t:f=w3644:dbl[])
                n880 = feedback #26(w3666) -> (w3679:dbl[])
                n881 = Build Array (concatenate)(w3679, w3666) -> (w3678:dbl[])
                n882 = Select(t=w3666, s=w3634, f=w3678) -> (s? t:f=w3653:dbl[])
                n883 = Divide(x=w3695, y=w3696) -> (x/y=w3698:dbl)
                n884 = Multiply(x=w3698, y=100.0) -> (x*y=w3697:dbl)
                n885 = Build Array(w3653, w3644) -> (→"Saved APD":dbl[][])
                n886 = Array Size(array=w3653) -> (size(s)=w3671:i32)
                n887 = Unbundle By Name(w3673) -> ("Y"=w3677:dbl[])
                n888 = Subtract(x=w3671, y="N pts to average") -> (x-y=w3647:i32)
                n889 = Multiply(x="N pts to average", y=u16 2) -> (x*y=w3648:u16)
                n890 = Subtract(x=w3671, y=w3648) -> (x-y=w3646:i32)
                n891 = feedback #27(w3677) -> (w3676:dbl[])
                n892 = Build Array (concatenate)(w3676, w3677) -> (w3675:dbl[])
                n893 = Select(t=w3677, s=w3634, f=w3675) -> (s? t:f=w3674:dbl[])
                "Trap Delta Graph" <- w3674
                n894 = Array Subset(array=w3653, index=w3647, length="N pts to average") -> (w3670:dbl[])
                n895 = Array Subset(array=w3653, index=w3646, length="N pts to average") -> (w3669:dbl[])
                n896 = Array Subset(array=w3644, index=w3647, length="N pts to average") -> (w3650:dbl[])
                n897 = Array Subset(array=w3644, index=w3646, length="N pts to average") -> (w3649:dbl[])
                n898 = call <vilib>:"Mean.vi"("X"=w3670) -> ("mean"=w3668:dbl)  [unwired: 1 out]
                n899 = call <vilib>:"Mean.vi"("X"=w3650) -> ("mean"=w3643:dbl)  [unwired: 1 out]
                n900 = call <vilib>:"Mean.vi"("X"=w3669) -> ("mean"=w3667:dbl)  [unwired: 1 out]
                n901 = call <vilib>:"Mean.vi"("X"=w3649) -> ("mean"=w3642:dbl)  [unwired: 1 out]
                n902 = Subtract(x=w3643, y=w3642) -> (x-y=w3633:dbl)
                "Delta Fl. 2" <- w3633
                n903 = Subtract(x=w3668, y=w3667) -> (x-y=w3665:dbl)
                "Delta Fl. 1" <- w3665
                n904 = Initialize Array(w3665, 1 ("dimension size")) -> (w3662:dbl[])
                n905 = Initialize Array(w3633, 1 ("dimension size")) -> (w3639:dbl[])
                n906 = feedback #28(w3662) -> (w3663:dbl[])
                n907 = Build Array (concatenate)(w3663, w3662) -> (w3661:dbl[])
                n908 = feedback #29(w3639) -> (w3640:dbl[])
                n909 = Build Array (concatenate)(w3640, w3639) -> (w3638:dbl[])
                n910 = Select(t=w3662, s=w3634, f=w3661) -> (s? t:f=w3637:dbl[])
                n911 = Select(t=w3639, s=w3634, f=w3638) -> (s? t:f=w3636:dbl[])
                n912 = Build Array(w3637, w3636) -> (→"Save APD Deriv":dbl[][])
              }
            }
            "Progress" <- w3619
            "Progress 2" <- w3619
          }
        }
      }
    }
    n913 = local read "AI2 (V)"() -> (w931:cluster{"Set 1":dbl, "Set 2":dbl})
    n914 = Bundle By Name(cluster=w931, "Set 1"=w930, "Set 2"=w929) -> (w927:cluster{"Set 1":dbl, "Set 2":dbl})
    n915 = Divide(x=w927, y=3276.7) -> (x/y=w926:cluster{"Set 1":dbl, "Set 2":dbl})
    n916 = local write "AI2 (V)"(w926) -> ()
    n917 = Divide(x=w864, y=3276.7) -> (x/y=w860:T36)
    n918 = Unbundle By Name(w860) -> ("Green FB Ch 0"=w863:dbl, "Green FB Ch 1"=w862:dbl, "Green FB Ch 2"=w861:dbl)
    n919 = Divide(x=w863, y=w861) -> (x/y=w859:dbl)
    n920 = Divide(x=w862, y=w861) -> (x/y=w858:dbl)
    n921 = Bundle By Name(cluster=w860, "Green FB Ch 0"=w859, "Green FB Ch 1"=w858) -> (w838:T36)
    "Green FB Signals (V)" <- w838
    n922 = Unbundle By Name(w838) -> ("Green FB Ch 2"=→"Green FB Plot":dbl)
    n923 = local read "wait to reset values"() -> (w935:bool)
    n924 = Not(x=w932) -> (.not. x?=w936:bool)
    n925 = And(x=w936, y=w935) -> (x .and. y?=w937:bool)
    n926 = case "Part of MCL raster scanning: returns to initial positions after scan done" shown="True" w937 {
      tunnel: w940 -> [w2350 w2357]
      tunnel: [w2350 w2356] -> w939
      tunnel: w934 -> [w2349 w2355]
      tunnel: [w2349 w2354] -> w933
      frame #0 {
      }
      frame #1 {
        w2365 = 10.0 ("y")
        w2364 = 32767.0 ("y")
        # "to return scan values\nafter a synchronous \nAOM scan"
        n927 = local read "AO2"() -> (w2358:dbl)
        n928 = local read "AO1"() -> (w2359:dbl)
        n929 = Multiply(x=w2359, y=w2364) -> (x*y=w2361:dbl)
        n930 = local write "wait to reset values"(FALSE ("wait to reset values")) -> ()
        n931 = Multiply(x=w2358, y=w2364) -> (x*y=w2363:dbl)
        n932 = Divide(x=w2361, y=w2365) -> (x/y=w2360:dbl)
        n933 = Divide(x=w2363, y=w2365) -> (x/y=w2362:dbl)
        n934 = To Word Integer(number=w2360) -> (16bit integer=w2366:i16)
        n935 = To Word Integer(number=w2362) -> (16bit integer=w2367:i16)
        n936 = local read "Total Counts (ticks)"() -> (w2351:u32)
        n937 = xnode "Read/Write Control"("FPGA VI Reference In"=w2357, "error in"=w2355, "AO1"=w2366, "AO2"=w2367, "MCL count"=w2351) -> ("FPGA VI Reference Out"=w2356:T15, "error out"=w2354:errorcluster)
        n938 = local read "Scan Range (V)\n(of steps)"() -> (w2352:dbl)
        n939 = property on="Scan Range (V)\n(of steps)" class="DigNum (strict)"("Val(Sgnl)"=w2352) -> ()  [unwired: 2 in, 2 out]
      }
    }
    n940 = node-c288() -> ()  [unwired: 2 out]
  }
  n941 = flat-sequence "Video" {
    tunnel: [w3800] -> w19
    tunnel: w19 -> [w3840]
    frame #0 {
      n942 = while {
        stop <- w3793 continue-if-true
        n943 = call "Close Video Capture.vi"() -> ("error code OUT"=w3795:i32)
        n944 = Equal?(x=w3795, y=0) -> (x = y?=w3793:bool)
      }
      n945 = local write "Stop All"(FALSE ("Stop All")) -> ()
    }
    frame #1 {
      n946 = call "DMR_Init.vi"() -> ()  [unwired: 3 out]
    }
    frame #2 {
      # "Setting the destination format to Mono8 makes sure that the image can be displayed in the intensity plot."
      n947 = call "DMR_GetDevice.vi"("search string IN"="DE019116701") -> ("device handle OUT"=w3818:i32)  [unwired: 4 in, 2 out]
      n948 = call "DMR_OpenDevice.vi"("device handle IN"=w3818) -> ("driver handle OUT"=w3801:i32)  [unwired: 4 out]
      n949 = call "DMR_FindList.vi"("flags IN"=u32 0 ("flags"), "list name IN"="" ("String"), "list type IN"=T37."camera descriptions", "driver handle IN"=w3801) -> ("list handle OUT"=w3804:i32)  [unwired: 2 out]
      n950 = call "DMR_FindList.vi"("flags IN"=u32 0 ("flags"), "list name IN"="Base", "list type IN"=T37."setting", "driver handle IN"=w3801) -> ("list handle OUT"=w3802:i32)  [unwired: 2 out]
      n951 = call "OBJ_GetHandle.vi"("object name IN"="VideoStandard", "list handle IN"=w3804) -> ("object handle OUT"=w3798:i32)  [unwired: 3 out]
      n952 = call "OBJ_GetHandle.vi"("object name IN"="PixelFormat", "list handle IN"=w3802) -> ("object handle OUT"=w3812:i32)  [unwired: 3 out]
      n953 = call "OBJ_SetS.vi"("value index IN"=0, "value IN"="NTSC M", "object handle IN"=w3798) -> ()  [unwired: 2 out]
      n954 = call "OBJ_SetS.vi"("value index IN"=0, "value IN"="Mono8" ("value"), "object handle IN"=w3812) -> ()  [unwired: 2 out]
      n955 = call "OBJ_GetHandle.vi"("object name IN"="VideoChannel", "list handle IN"=w3802) -> ("object handle OUT"=w3808:i32)  [unwired: 3 out]
      n956 = while {
        tunnel: [w3823] -> w3800
        tunnel: w3801 -> [w3820]
        stop <- w3821 continue-if-true
        n957 = call "DMR_ImageRequestSingle.vi"("request control IN"=0, "driver handle IN"=w3820) -> ("error code OUT"=w3822:i32, "driver handle OUT"=w3823:i32)  [unwired: 2 out]
        n958 = Equal To 0?(x=w3822) -> (x = 0?=w3821:bool)
      }
      n959 = call "OBJ_SetI.vi"("value index IN"=0, "value IN"=3 ("Video channel"), "object handle IN"=w3808) -> ()  [unwired: 2 out]
    }
    frame #3 {
      w3828 = T13 0 items=["Grayscale (U8)", "Grayscale (I16)", "Grayscale (SGL)", "Complex (CSG)", "RGB (U32)", "HSL (U32)", "RGB (U64)"] ("Image Type")
      w3836 = T13 0 items=["Grayscale (U8)", "Grayscale (I16)", "Grayscale (SGL)", "Complex (CSG)", "RGB (U32)", "HSL (U32)", "RGB (U64)"] ("Image Type")
      n960 = for "Create Greyscale map" {
        N: 256 -> [_]
        tunnel: [w3842] -> w3825 mode=indexing
        workers-P: _ -> [_]
        i -> [w3845]
        n961 = To Unsigned Byte Integer(number=w3845) -> (unsigned 8bit integer=w3841:u8)
        n962 = Join Numbers(hi=w3841, lo=w3841) -> ((hi.lo)=w3844:u16)
        n963 = Join Numbers(hi=w3841, lo=w3841) -> ((hi.lo)=w3843:u16)
        n964 = Join Numbers(hi=w3844, lo=w3843) -> ((hi.lo)=w3842:u32)
      }
      n965 = call "IMAQ Create"("Image Name"="Scaled video", "Image Type"=w3828) -> ("New Image"=w3827:T2)  [unwired: 2 in, 2 out]
      n966 = call "IMAQ Create"("Image Name"="Main video", "Image Type"=w3836) -> ("New Image"=w3837:T2)  [unwired: 2 in, 2 out]
      n967 = node-c288() -> (w3835:T19)  [unwired: 4 out]
      n968 = Initialize Array(u32 0 ("Window Number (0...15)"), 480 ("dimension size"), 640 ("dimension size")) -> (w3830:u32[][])
      n969 = timed-loop {
        tunnel: w3840 -> [w3862]
        tunnel: [w3861] -> w3839
        tunnel: w3837 -> [w3860]
        timing: w3835 -> [_]
        timing-out: [_] -> w3834
        tunnel: w3830 -> [w3849]
        tunnel: w3827 -> [w3847]
        tunnel: w3825 -> [w3846]
        stop <- w3848 stop-if-true
        # "This block performs the \nactual image capture."
        n970 = node-c288() -> ()  [unwired: 2 out]
        n971 = local read "Stop All"() -> (w3848:bool)
        n972 = Reciprocal(x="Video Capture Rate (Hz)") -> (1/x=w3852:dbl)
        n973 = Multiply(x=w3852, y=1000.0) -> (x*y=w3850:dbl)
        n974 = call "DMR_ImageRequestWaitFor.vi"("queue number IN"=0, "timeout(ms) IN"=500, "driver handle IN"=w3862) -> ("error code OUT"=w3866:i32, "request number OUT"=w3863:i32, "driver handle OUT"=w3864:i32)
        n975 = feedback #30(T38 refnum ("Avi Refnum")) -> (w3854:T38)
        n976 = case shown="True" "New Video File" {
          tunnel: [T38 refnum ("Avi Refnum") w3883] -> w3856
          tunnel: [FALSE TRUE] -> w3857
          tunnel: w3854 -> [_ w3879]
          frame #0 {
          }
          frame #1 {
            n977 = call "Create new save file.vi"("Ext"=".avi" ("string"), "Index In"="Video Index") -> ("Path Out"=w3875:path, "Index Out"=w3876:dbl)  [unwired: 1 in]
            "Path Out" <- w3875
            n978 = Not Equal?(x=w3879, y=T38 refnum ("Avi Refnum")) -> (x != y?=w3880:bool)
            n979 = Increment(x=w3876) -> (x+1=w3885:dbl)
            n980 = case shown="True" w3880 {
              tunnel: w3879 -> [_ w3886]
              frame #0 {
              }
              frame #1 {
                n981 = call "IMAQ AVI Close"("Avi Refnum"=w3886) -> ()  [unwired: 1 in, 10 out]
              }
            }
            n982 = call "IMAQ AVI Create"("Frames Per Second"=u32 30, "AVI Path"=w3875) -> ("Avi Refnum"=w3883:T38)  [unwired: 5 in, 4 out]
            n983 = local write "Video Index"(w3885) -> ()
          }
        }
        n984 = Equal To 0?(x=w3866) -> (x = 0?=w3865:bool)
        n985 = Select(t=w3856, s=w3857, f=w3854) -> (s? t:f=w3855:T38)
        n986 = case shown="True" w3865 {
          tunnel: w3864 -> [w3887 w3912]
          tunnel: w3863 -> [_ w3911]
          tunnel: [w3887 w3908] -> w3861
          tunnel: w3860 -> [_ w3892]
          tunnel: w3849 -> [_ w3896]
          tunnel: w3855 -> [_ w3894]
          tunnel: w3847 -> [_ w3889]
          tunnel: w3846 -> [_ w3888]
          frame #0 {
          }
          frame #1 {
            w3902 = u32 0 ("X-offset IN")
            n987 = call "DMR_GetImageRequestBufferData.vi"("driver handle IN"=w3912, "request number IN"=w3911) -> ("width OUT"=w3901:i32, "height OUT"=w3900:i32, "driver handle OUT"=w3907:i32, "request number OUT"=w3906:i32, "bytes per pixel OUT"=w3903:i32)  [unwired: 13 out]
            n988 = call "DMR_GetImageRequestBufferImageData.vi"("driver handle IN"=w3907, "request number IN"=w3906, "bytes per pixel IN"=w3903, "X-offset IN"=w3902, "Y-offset IN"=w3902, "height IN"=w3900, "width IN"=w3901) -> ("driver handle OUT"=w3905:u32, "request number OUT"=w3904:u32, "image OUT"=w3897:u32[][])  [unwired: 10 out]
            n989 = call "DMR_ImageRequestUnlock.vi"("request number IN"=w3904, "driver handle IN"=w3905) -> ("driver handle OUT"=w3910:i32)  [unwired: 1 in, 2 out]
            n990 = case shown="True" "Averaging" {
              tunnel: w3897 -> [w3948 w3953]
              tunnel: [w3948 w3952] -> w3893
              tunnel: w3896 -> [_ w3950]
              frame #0 {
              }
              frame #1 {
                (unwired) 1
                w3958 = 1
                n991 = feedback #31(w3950) -> (w3949:u32[][])
                n992 = Add(x=w3953, y=w3949) -> (x+y=w3954:u32[][])
                n993 = Select(t=w3950, s="Reset Averaging", f=w3954) -> (s? t:f=w3956:u32[][])
                n994 = feedback #32(w3958) -> (w3951:i32)
                n995 = Divide(x=w3954, y=w3951) -> (x/y=w3955:dbl[][])
                n996 = Increment(x=w3951) -> (x+1=w3959:i32)
                n997 = To Unsigned Long Integer(number=w3955) -> (unsigned 32bit integer=w3952:u32[][])
                n998 = Select(t=w3958, s="Reset Averaging", f=w3959) -> (s? t:f=w3957:i32)
              }
            }
            n999 = call "DMR_ImageRequestSingle.vi"("request control IN"=0, "driver handle IN"=w3910) -> ("driver handle OUT"=w3908:i32)  [unwired: 3 out]
            n1000 = disable-structure shown="Disabled" {
              disable-tunnel: w3893 -> [w3925 _]
              disable-tunnel: w3889 -> [w3924 _]
              frame #0 {
                n1001 = To Double Precision Float(number=w3925) -> (double precision float=w3923:dbl[][])
                n1002 = In Range and Coerce(upper limit="Intensity Upper", x=w3923, lower limit="Intensity Lower") -> (coerced(x)=w3922:dbl[][])  [unwired: 1 out]
                n1003 = Subtract(x="Intensity Upper", y="Intensity Lower") -> (x-y=w3919:dbl)
                n1004 = Subtract(x=w3922, y="Intensity Lower") -> (x-y=w3920:dbl[][])
                n1005 = Divide(x=w3920, y=w3919) -> (x/y=w3921:dbl[][])
                n1006 = Multiply(x=255.0, y=w3921) -> (x*y=w3917:dbl[][])
                n1007 = To Unsigned Byte Integer(number=w3917) -> (unsigned 8bit integer=w3926:u8[][])
                n1008 = call "IMAQ ArrayToImage"("Image Pixels (U8)"=w3926, "Image"=w3924) -> ("Image Out"=w3913:T2)  [unwired: 4 in, 5 out]
                n1009 = First Call?() -> (First Call?: T/F=w3914:bool)
                n1010 = case shown="True" w3914 {
                  tunnel: w3913 -> [w3927 w3938]
                  frame #0 {
                    n1011 = flat-sequence {
                      tunnel: w3927 -> [w3933]
                      frame #0 {
                        w3930 = FALSE ("Get/Set Status? (Set)")
                        w3929 = 0 ("Window Number (0...15)")
                        n1012 = call "IMAQ WindSize"("Get/Set Status? (Set)"=w3930, "Window Number"=w3929) -> ("Width & Height out"=→"Window Size":cluster{"Width":i32, "Height":i32})  [unwired: 4 in, 2 out]
                        n1013 = call "IMAQ WindMove"("Window Number (0...15)"=w3929, "Get/Set Status? (Set)"=w3930) -> ("Coordinates (screen)"=→"Window Position":cluster{"X Position":i32, "Y Position":i32})  [unwired: 3 in, 1 out]
                        n1014 = call "IMAQ WindDraw"("Resize to Image Size? (Y)"=FALSE, "Window Number (0...15)"=w3929, "Image"=w3933) -> ()  [unwired: 7 in, 2 out]
                      }
                      frame #1 {
                        n1015 = call "IMAQ WindZoom 2"("Center Point"="Center Point", "Zoom to Fit? (False)"=FALSE, "Zoom Factor"="Zoom Factor") -> ()  [unwired: 5 in, 4 out]
                      }
                    }
                  }
                  frame #1 {
                    n1016 = flat-sequence {
                      tunnel: w3938 -> [w3941]
                      tunnel: [w3939] -> w3937
                      tunnel: w3937 -> [w3943]
                      frame #0 {
                        w3940 = TRUE ("Resize to Image Size? (Y)")
                        w3939 = 0 ("Window Number (0...15)")
                        n1017 = call "IMAQ WindNonTearing"("Window Number"=w3939, "NonTearing? (True)"=w3940) -> ()  [unwired: 8 in, 2 out]
                        n1018 = call "IMAQ WindDraw"("Resize to Image Size? (Y)"=w3940, "Window Number (0...15)"=w3939, "Image"=w3941) -> ()  [unwired: 7 in, 2 out]
                      }
                      frame #1 {
                        n1019 = call "IMAQ WindSize"("Scrollbars? (N)"=FALSE, "Width & Height"="Initial Window Size", "Window Number"=w3943) -> ()  [unwired: 3 in, 3 out]
                        n1020 = call "IMAQ WindMove"("Window Number (0...15)"=w3943, "Coordinates (screen)"="Initial Window Position") -> ()  [unwired: 3 in, 2 out]
                      }
                    }
                  }
                }
              }
              frame #1 {
              }
            }
            n1021 = To Unsigned Byte Integer(number=w3893) -> (unsigned 8bit integer=w3891:u8[][])
            n1022 = call "IMAQ ArrayToImage"("Image Pixels (U8)"=w3891, "Image"=w3892) -> ("Image Out"=w3890:T2)  [unwired: 4 in, 5 out]
            "Primary Video Display" <- w3890
            n1023 = case shown="True" "Save Video" {
              tunnel: w3894 -> [_ w3947]
              tunnel: w3890 -> [_ w3946]
              frame #0 {
              }
              frame #1 {
                n1024 = call "IMAQ AVI Write Frame"("Image"=w3946, "Avi Refnum"=w3947) -> ()  [unwired: 2 in, 8 out]
              }
            }
            n1025 = case shown="True" "Save Image" {
              tunnel: w3891 -> [_ w3962]
              tunnel: w3888 -> [_ w3961]
              frame #0 {
              }
              frame #1 {
                n1026 = call <vilib>:"Flatten Pixmap.vi"("colors"=w3961, "8-bit pixmap"=w3962) -> ("image data"=w3968:T39)  [unwired: 4 in, 5 out]
                n1027 = call "Create new save file.vi"("Insert"="video_frame_" ("string"), "Ext"=".bmp" ("string"), "Index In"="Image Index") -> ("Path Out"=w3964:path, "Index Out"=w3969:dbl)
                n1028 = Increment(x=w3969) -> (x+1=w3963:dbl)
                n1029 = local write "Image Index"(w3963) -> ()
                n1030 = call <vilib>:"Write BMP File.vi"("image data"=w3968, "path to BMP file"=w3964) -> ()  [unwired: 1 in, 9 out]
              }
            }
          }
        }
        n1031 = node-c288(w3850) -> ()  [unwired: 1 out]
      }
      n1032 = node-c288(w3834) -> ()  [unwired: 1 out]
      n1033 = call "DMR_CloseDevice.vi"("driver handle IN"=w3839) -> ()  [unwired: 1 in, 4 out]
    }
    frame #4 {
      n1034 = call "DMR_Close.vi"() -> ()  [unwired: 1 out]
    }
  }
  n1035 = disable-structure shown="Disabled" {
    disable-tunnel: [w3973 _] -> w195
    disable-tunnel: w89 -> [w3972 _]
    frame #0 {
      n1036 = node-c288() -> (w3975:T19)  [unwired: 4 out]
      n1037 = timed-loop "Rough control of MCL mirror stage (debugging)" {
        tunnel: w3972 -> [w3978]
        tunnel: [w3977] -> w3973
        timing: w3975 -> [_]
        timing-out: [_] -> w3974
        stop <- w3977 stop-if-true
        n1038 = node-c288() -> ()  [unwired: 2 out]
        n1039 = case shown="1" "MCL Mode" {
          tunnel: w3978 -> [_ w3981 w4083]
          frame #0 {
          }
          frame #1 {
            n1040 = node-c288() -> (w3983:T19)  [unwired: 4 out]
            n1041 = timed-loop "Oscillate MCL mirror" {
              timing: w3983 -> [_]
              timing-out: [_] -> w3982
              tunnel: w3981 -> [w4022]
              i -> [w4021]
              stop <- w3984 stop-if-true
              n1042 = node-c288() -> (w4020:i64)  [unwired: 1 out]
              n1043 = Multiply(x="AO1", y=32767.0) -> (x*y=w4016:dbl)
              n1044 = Multiply(x="AO2", y=32767.0) -> (x*y=w4011:dbl)
              n1045 = Divide(x=w4016, y=10.0) -> (x/y=w4017:dbl)
              n1046 = Divide(x=w4011, y=10.0) -> (x/y=w4012:dbl)
              n1047 = To Word Integer(number=w4017) -> (16bit integer=w4009:i16)
              n1048 = To Word Integer(number=w4012) -> (16bit integer=w4008:i16)
              n1049 = Divide(x=w4020, y=i64 1000) -> (x/y=w3991:dbl)
              n1050 = Multiply(x=w3991, y=w4021) -> (x*y=w4002:dbl)
              n1051 = Multiply(x="Osc. freq. (Hz) 2", y=6.283185307179586) -> (x*y=w4003:dbl)
              n1052 = Multiply(x=w4003, y=w4002) -> (x*y=w4001:dbl)
              n1053 = Sine(x=w4001) -> (sin(x)=w4000:dbl)
              n1054 = Multiply(x=w4000, y="Osc. amp. (V)") -> (x*y=w3998:dbl)
              n1055 = Add(x=w3998, y="Osc. center (V)") -> (x+y=w3996:dbl)
              n1056 = Divide(x=w3996, y=10.0) -> (x/y=w3994:dbl)
              n1057 = Multiply(x=w3994, y=32767.0) -> (x*y=w3989:dbl)
              n1058 = Select(t=w3989, s="Scan axis", f=w4009) -> (s? t:f=w4007:dbl)
              n1059 = Select(t=w4008, s="Scan axis", f=w3989) -> (s? t:f=w4006:dbl)
              n1060 = local read "MCL Mode"() -> (w3988:u16)
              n1061 = Not Equal?(x=w3988, y=u16 1) -> (x != y?=w3985:bool)
              n1062 = local read "Stop All"() -> (w3986:bool)
              n1063 = xnode "Read/Write Control"("FPGA VI Reference In"=w4022, "AO1"=w4007, "AO2"=w4006) -> ()  [unwired: 1 in, 2 out]
              n1064 = Compound Arithmetic op=OR(w3986, w3985) -> (w3984:bool)
              n1065 = node-c288() -> ()  [unwired: 2 out]
            }
            n1066 = node-c288(w3982) -> ()  [unwired: 1 out]
          }
          frame #2 {
            n1067 = case shown="True" "Start Scan" {
              tunnel: w4083 -> [_ w4095]
              frame #0 {
              }
              frame #1 {
                n1068 = Subtract(x="End (V)", y="Begin (V)") -> (x-y=w4091:dbl)
                n1069 = Decrement(x="N Points") -> (x-1=w4090:dbl)
                n1070 = Divide(x=w4091, y=w4090) -> (x/y=w4088:dbl)
                n1071 = for {
                  N: "N Points" -> [_]
                  tunnel: "Begin (V)" -> [w4108]
                  tunnel: w4095 -> [w4100]
                  tunnel: [w4099] -> w4094 mode=indexing
                  tunnel: w4088 -> [w4098]
                  tunnel: [w4096] -> w4087 mode=indexing
                  i -> [w4107]
                  n1072 = Multiply(x=w4098, y=w4107) -> (x*y=w4106:dbl)
                  n1073 = Add(x=w4108, y=w4106) -> (x+y=w4103:dbl)
                  n1074 = local read "Scan axis"() -> (w4097:bool)
                  n1075 = local read "AO1"() -> (w4105:dbl)
                  n1076 = local read "AO2"() -> (w4104:dbl)
                  n1077 = Select(t=w4103, s=w4097, f=w4105) -> (s? t:f=w4102:dbl)
                  n1078 = Select(t=w4104, s=w4097, f=w4103) -> (s? t:f=w4101:dbl)
                  n1079 = flat-sequence {
                    tunnel: w4102 -> [w4112]
                    tunnel: w4101 -> [w4111]
                    tunnel: w4100 -> [w4109]
                    tunnel: [w4177] -> w4099
                    tunnel: [w4176] -> w4096
                    frame #0 {
                      w4115 = 10.0 ("y")
                      w4110 = 32767.0 ("y")
                      n1080 = Multiply(x=w4112, y=w4110) -> (x*y=w4118:dbl)
                      n1081 = Multiply(x=w4111, y=w4110) -> (x*y=w4116:dbl)
                      n1082 = Divide(x=w4118, y=w4115) -> (x/y=w4119:dbl)
                      n1083 = Divide(x=w4116, y=w4115) -> (x/y=w4117:dbl)
                      n1084 = To Word Integer(number=w4119) -> (16bit integer=w4113:i16)
                      n1085 = To Word Integer(number=w4117) -> (16bit integer=w4114:i16)
                      n1086 = xnode "Read/Write Control"("FPGA VI Reference In"=w4109, "AO1"=w4113, "AO2"=w4114) -> ()  [unwired: 1 in, 2 out]
                    }
                    frame #1 {
                      n1087 = Wait (ms)(milliseconds to wait="DAQ Delay (ms)") -> ()  [unwired: 1 out]
                    }
                    frame #2 {
                      n1088 = local read "Slow mean"() -> (w4177:dbl)
                      n1089 = local read "Sigma"() -> (w4176:dbl)
                    }
                  }
                }
                n1090 = Bundle("Begin (V)"="Begin (V)", w4088, w4094) -> (→"MCL Scan":cluster{"Begin (V)":dbl, dbl, dbl[]})  [unwired: 1 out]
                n1091 = Bundle("Begin (V)"="Begin (V)", w4088, w4087) -> (→"MCL Scan 2":cluster{"Begin (V)":dbl, dbl, dbl[]})  [unwired: 1 out]
              }
            }
          }
        }
        n1092 = local read "Stop All"() -> (w3977:bool)
        n1093 = node-c288() -> ()  [unwired: 2 out]
      }
      n1094 = node-c288(w3974) -> ()  [unwired: 1 out]
    }
    frame #1 {
    }
  }
  n1095 = timed-loop "Control parameters (event loop)" {
    tunnel: w89 -> [w4184]
    shift-right: [w4183] -> _
    shift-left: errorcluster {"status"=FALSE, "code"=0, "source"=""} ("error out") -> [w4182]
    tunnel: [w4181] -> w193
    timing: w31 -> [_]
    timing-out: [_] -> w30
    tunnel: w1 -> [w4180]
    stop <- w4181 stop-if-true
    n1096 = node-c288() -> ()  [unwired: 2 out]
    n1097 = event shown="[42] \"Sample Channel Flow\": Value Change" {
      selector: _ -> [_ _ _ _ _ _ _ _ _ _ _ _ _ _ _ _ _ _ _ _ _ _ _ _ _ _ _ _ _ _ _ _ _ _ _ _ _ _ _ _ _ _ _ _ _]
      dyn-events: _ -> [_ _ _ _ _ _ _ _ _ _ _ _ _ _ _ _ _ _ _ _ _ _ _ _ _ _ _ _ _ _ _ _ _ _ _ _ _ _ _ _ _ _ _ _ _]
      timeout: _ -> [_ _ _ _ _ _ _ _ _ _ _ _ _ _ _ _ _ _ _ _ _ _ _ _ _ _ _ _ _ _ _ _ _ _ _ _ _ _ _ _ _ _ _ _ _]
      tunnel: w4184 -> [w4225 _ _ w4352 _ w4447 _ _ _ _ w4513 _ _ w4613 w4751 w4813 w4856 w5006 w5081 w5192 w5285 w5369 w5453 w5537 w5621 w5705 w5798 w5993 w6193 w6286 w6419 _ w6589 w6630 w6677 w6754 w6795 _ w6840 _ _ _ _ w7021 _]
      tunnel: [w4224 _ _ w4342 _ w4446 _ _ w4478 _ w4492 _ _ w4612 w4747 w4810 w4853 w5005 w5079 w5191 w5279 w5363 w5447 w5531 w5615 w5699 w5796 w5992 w6191 w6284 w6417 _ w6587 w6628 w6667 w6752 w6793 _ w6838 _ _ _ _ w7019 _] -> w4183
      tunnel: w4182 -> [w4223 _ _ w4351 _ w4445 _ _ w4478 _ w4512 _ _ w4611 w4746 w4809 w4852 w5004 w5080 w5190 w5284 w5368 w5452 w5536 w5620 w5704 w5797 w5991 w6192 w6285 w6418 _ w6588 w6629 w6676 w6753 w6794 _ w6839 _ _ _ _ w7020 _]
      tunnel: [_ _ _ _ _ _ _ _ w4477 _ _ _ _ _ _ _ _ _ _ _ _ _ _ _ _ _ _ _ _ _ _ _ _ _ _ _ _ _ _ _ _ _ _ _ _] -> w4181
      tunnel: [_ _ _ _ _ _ "Round T1 X" _ _ _ _ "Load parameters" _ _ _ _ _ _ _ _ _ _ _ _ _ _ _ _ _ _ _ _ _ _ _ _ _ _ _ _ _ _ _ _ _] -> _
      tunnel: [_ _ "Adjust Scale\nto Mean" _ _ _ _ _ _ _ _ _ _ _ _ _ _ _ _ _ _ _ _ _ _ _ _ _ _ _ _ _ _ _ _ _ _ _ _ _ _ _ _ _ _] -> _
      tunnel: [_ _ _ _ _ _ _ "Round T2 X" _ "Delayed Interlace Start" _ _ _ _ _ _ _ _ _ _ _ _ _ _ _ _ _ _ _ _ _ _ _ _ _ _ _ _ _ _ _ _ _ _ _] -> _
      tunnel: [_ "Rescale on Mean" _ _ _ _ _ _ _ _ _ _ _ _ _ _ _ _ _ _ _ _ _ _ _ _ _ _ _ _ _ _ _ _ _ _ _ _ _ _ _ _ _ _ _] -> _
      tunnel: w4180 -> [_ _ _ _ _ _ _ _ _ _ _ _ _ _ _ _ _ _ _ _ _ _ _ _ _ _ _ _ _ _ _ _ _ _ _ _ _ _ _ _ _ _ w7012 _ _]
      event #0 {
        # "So that if 'Save ave N' is updated, the AOD scanning code updates too."
        n1098 = event-data() -> ()  [unwired: 6 out]
        n1099 = local read "AI Count (ticks)"() -> (w4195:u32)
        n1100 = local read "FPGA Ave."() -> (w4199:dbl)
        n1101 = Boolean To (0,1)(Boolean="Sets to FIFO (Traps)") -> (0, 1=w4213:cluster{"Set 1":i16, "Set 2":i16, "Set 3":i16})
        n1102 = xnode "Read/Write Control"("FPGA VI Reference In"=w4225, "error in"=w4223, "ai count"=w4195, "AI1 Sets to FIFO"="Sets to FIFO (Traps)", "AI Averages"=w4199, "N of AI1 Int Acq Sets"="N Acq Sets (Traps + Fl.)") -> ("error out"=w4224:errorcluster)  [unwired: 1 out]
        n1103 = Cluster To Array(cluster=w4213) -> (array=w4212:i16[])
        n1104 = local read "Scan steps (AOD)"() -> (w4214:u64)
        n1105 = Multiply(x=w4195, y="N Acq Sets (Traps + Fl.)") -> (x*y=w4193:u32)
        n1106 = Divide(x=40000000.0, y=w4195) -> (x/y=w4221:dbl)
        "AI rate (Hz)" <- w4221
        n1107 = Add Array Elements(numeric array=w4212) -> (sum=w4197:i16)
        "Trap Sets" <- w4197
        n1108 = Divide(x=w4221, y=w4199) -> (x/y=w4222:dbl)
        "Ave. Rate (Hz)" <- w4222
        n1109 = Reciprocal(x=w4222) -> (1/x=→"Ave. Period (s)":dbl)
        n1110 = property on="Scan steps (AOD)" class="DigNum (strict)"("Val(Sgnl)"=w4214) -> ()  [unwired: 2 in, 2 out]
        n1111 = Divide(x=w4222, y="N Acq Sets (Traps + Fl.)") -> (x/y=w4218:dbl)
        "Data Rate (Hz)" <- w4218
        n1112 = Reciprocal(x=w4218) -> (1/x=→"Data Period (s)":dbl)
        n1113 = local read "Save ave N"() -> (w4217:dbl)
        n1114 = Divide(x=w4218, y=w4217) -> (x/y=w4216:dbl)
        "Save Data Rate (Hz)" <- w4216
        n1115 = Reciprocal(x=w4216) -> (1/x=→"Save Data Period (s)":dbl)
        n1116 = Multiply(x=w4193, y="# Samples/trap") -> (x*y=w4189:dbl)
        "Counts/DMA" <- w4189
        n1117 = Multiply(x=w4197, y="# Samples/trap") -> (x*y=w4196:dbl)
        "# Samples/channel" <- w4196
        n1118 = Greater?(x=w4199, y=1.0) -> (0:w4202:bool)
        "FPGA Averaging" <- w4202
        n1119 = local read "APD Int. Count"() -> (w4191:u32)
        n1120 = Divide(x=w4196, y=u32 2) -> (x/y=w4205:dbl)
        n1121 = Select(t=w4196, s=w4202, f=w4205) -> (s? t:f=w4210:dbl)
        n1122 = Divide(x=w4189, y=w4191) -> (x/y=w4190:dbl)
        "APD Samples/FIFO Acq." <- w4190
        n1123 = Divide(x=w4189, y=40000000.0) -> (x/y=w4187:dbl)
        "DMA Update Period (s)" <- w4187
        n1124 = Multiply(x=w4210, y=u32 8) -> (x*y=→"Elements/DMA read":dbl)
        n1125 = Multiply(x=2.0, y=w4190) -> (x*y=→"APD Elements/DMA read":dbl)
        n1126 = local read "N sets to save"() -> (w4207:u32)
        n1127 = Multiply(x=w4187, y=w4207) -> (x*y=→"Total Time (s)":dbl)
      }
      event #1 {
        n1128 = event-data() -> ()  [unwired: 7 out]
        n1129 = local read "Bead Mean (nm)"() -> (w4330:dbl)
        n1130 = Add(x="Amplitude (nm)", y=w4330) -> (x+y=w4328:dbl)
        n1131 = Subtract(x=w4330, y="Amplitude (nm)") -> (x-y=w4327:dbl)
        n1132 = property on="Bead Separation" class="WFChart (strict)"("YScale.Minimum"=w4327) -> ()  [unwired: 2 in, 2 out]
        n1133 = property on="Bead Separation" class="WFChart (strict)"("YScale.Maximum"=w4328) -> ()  [unwired: 2 in, 2 out]
      }
      event #2 {
        n1134 = event-data() -> ()  [unwired: 7 out]
        n1135 = local read "APD 1 Rate (Hz)"() -> (w4339:dbl)
        n1136 = Multiply(x=1000.0, y="Above (kHz)") -> (x*y=w4337:dbl)
        n1137 = Multiply(x=1000.0, y="Below (kHz)") -> (x*y=w4335:dbl)
        n1138 = Add(x=w4337, y=w4339) -> (x+y=w4332:dbl)
        n1139 = Subtract(x=w4339, y=w4335) -> (x-y=w4333:dbl)
        n1140 = property on="APD Chart" class="WFChart (strict)"("YScale.Minimum"=w4333) -> ()  [unwired: 2 in, 2 out]
        n1141 = property on="APD Chart" class="WFChart (strict)"("YScale.Maximum"=w4332) -> ()  [unwired: 2 in, 2 out]
      }
      event #3 {
        n1142 = event-data() -> ()  [unwired: 7 out]
        n1143 = Negate(x="Phase adj. (AI1)") -> (-x=w4349:i16)
        n1144 = Select(t=w4349, s="- phase (AI1)", f="Phase adj. (AI1)") -> (s? t:f=w4348:i16)
        n1145 = xnode "Read/Write Control"("FPGA VI Reference In"=w4352, "error in"=w4351, "Phase count adjustment"=w4348) -> ("FPGA VI Reference Out"=w4347:T15, "error out"=w4346:errorcluster)
        n1146 = Or(x="- phase (AI1)", y="+ phase (AI1)") -> (x .or. y?=w4343:bool)
        n1147 = xnode "Read/Write Control"("FPGA VI Reference In"=w4347, "error in"=w4346, "+ phase"=w4343) -> ("error out"=w4342:errorcluster)  [unwired: 1 out]
      }
      event #4 {
        w4428 = u32 9868950 ("Color Box")
        n1148 = event-data() -> ("Row"=w4430:i32)  [unwired: 9 out]
        n1149 = property on="All Signals" class="WFChart (strict)"("Active Plot"=w4430) -> (error out=w4441:errorcluster)  [unwired: 2 in, 1 out]
        n1150 = property on="All Signals" class="WFChart (strict)" props=["Plot", "Visible?", "Plot", "Plot Color"](error in=w4441) -> (error out=w4440:errorcluster, "Plot.Visible?"=w4439:bool)  [unwired: 1 in, 2 out]
        n1151 = Select(t=FALSE ("Plot.Visible"), s=w4439, f=TRUE ("Plot.Visible")) -> (s? t:f=w4434:bool)
        n1152 = property on="All Signals" class="WFChart (strict)"(error in=w4440, "Plot.Visible?"=w4434) -> (error out=w4436:errorcluster)  [unwired: 1 in, 1 out]
        n1153 = property on="All Signals" class="WFChart (strict)"(error in=w4436) -> (error out=w4431:errorcluster, "Plot.Plot Color"=w4435:u32)  [unwired: 1 in, 1 out]
        n1154 = property on="Signals to Plot" class="LstBox (strict)"(error in=w4431, "Active Row"=w4430) -> (error out=w4429:errorcluster)  [unwired: 1 in, 1 out]
        n1155 = Select(t=w4435, s=w4434, f=u32 0) -> (s? t:f=w4432:u32)
        n1156 = property on="Signals to Plot" class="LstBox (strict)"(error in=w4429, "CellFontColor"=w4432, "SelColor"=w4428, "CellBG"=w4428, "CellFontSize"=u32 20 ("Active Row:Cell Font:Size"), "CellFontBold"=TRUE ("Active Row:Cell Font:Bold")) -> ()  [unwired: 1 in, 2 out]
      }
      event #5 {
        n1157 = event-data() -> ("CtlRef"=w4444:refnum<vi>)  [unwired: 6 out]
        n1158 = control-ref of="Trap Delta (MHz)"() -> (w4443:refnum<vi>)
        n1159 = Equal?(x=w4443, y=w4444) -> (x = y?=w4442:bool)
        n1160 = case shown="False" "Oscillate Set 1" {
          tunnel: w4447 -> [w4467 _]
          tunnel: [w4466 w4470] -> w4446
          tunnel: w4445 -> [w4465 w4470]
          tunnel: w4442 -> [w4450 _]
          frame #0 {
            n1161 = local read "BD 1 Frequency 2 (MHz)"() -> (w4454:dbl)
            n1162 = local read "BD 1 Frequency 1 (MHz)"() -> (w4452:dbl)
            n1163 = Subtract(x=w4454, y="Trap Delta (MHz)") -> (x-y=w4451:dbl)
            n1164 = Select(t=w4451, s=w4450, f=w4452) -> (s? t:f=w4449:dbl)
            n1165 = local read "Y RF Frequency Limits (MHz)"() -> (w4455:T12)
            n1166 = local read "X RF Frequency Limits (MHz)"() -> (w4456:T12)
            n1167 = local read "BD 1 Frequency 3 (MHz)"() -> (w4468:dbl)
            n1168 = local write "BD 1 Frequency 1 (MHz)"(w4449) -> ()
            n1169 = local read "BD 2 Frequency 1 (MHz)"() -> (w4459:dbl)
            n1170 = local read "BD 2 Frequency 2 (MHz)"() -> (w4458:dbl)
            n1171 = local read "BD 2 Frequency 3 (MHz)"() -> (w4469:dbl)
            n1172 = call "set RF board frequency - interlace.vi"("Board 2 Frequency Limits"=w4455, "Board 1 Frequency Limits"=w4456, "error in"=w4465, "FPGA VI Reference In"=w4467, "Board 2 Frequency 3 (MHz)"=w4469, "Board 1 Frequency 3 (MHz)"=w4468, "Board 2 Frequency 2 (MHz)"=w4458, "Board 2 Frequency 1 (MHz)"=w4459, "Board 1 Frequency 2 (MHz)"=w4454, "Board 1 Frequency 1  (MHz)"=w4449) -> ("error out"=w4466:errorcluster)  [unwired: 1 out]
            n1173 = Subtract(x=w4459, y=w4458) -> (x-y=w4463:dbl)
            n1174 = Subtract(x=w4449, y=w4454) -> (x-y=w4464:dbl)
            n1175 = Square(x=w4463) -> (x^2=w4461:dbl)
            n1176 = Square(x=w4464) -> (x^2=w4462:dbl)
            n1177 = Add(x=w4462, y=w4461) -> (x+y=w4460:dbl)
            n1178 = Square Root(x=w4460) -> (sqrt(x)=w4457:dbl)
            n1179 = local write "Trap Delta (MHz)"(w4457) -> ()
            n1180 = property on="Initial delta (MHz)" class="DigNum (strict)"("Val(Sgnl)"=w4457) -> ()  [unwired: 2 in, 2 out]
          }
          frame #1 {
          }
        }
      }
      event #6 {
        n1181 = event-data() -> ()  [unwired: 7 out]
        n1182 = local read "BD 1 Frequency 1 (MHz)"() -> (w4473:dbl)
        n1183 = Round To Nearest(number=w4473) -> (nearest integer value=w4472:dbl)
        n1184 = property on="BD 1 Frequency 1 (MHz)" class="DigNum (strict)"("Val(Sgnl)"=w4472) -> ()  [unwired: 2 in, 2 out]
      }
      event #7 {
        n1185 = event-data() -> ()  [unwired: 7 out]
        n1186 = local read "BD 1 Frequency 2 (MHz)"() -> (w4475:dbl)
        n1187 = Round To Nearest(number=w4475) -> (nearest integer value=w4474:dbl)
        n1188 = property on="BD 1 Frequency 2 (MHz)" class="DigNum (strict)"("Val(Sgnl)"=w4474) -> ()  [unwired: 2 in, 2 out]
      }
      event #8 {
        n1189 = event-data() -> ()  [unwired: 7 out]
        n1190 = local read "Stop All"() -> (w4477:bool)
      }
      event #9 {
        n1191 = event-data() -> ()  [unwired: 7 out]
        n1192 = flat-sequence {
          frame #0 {
            n1193 = Multiply(x="Delay to Interlace (s)", y=1000.0) -> (x*y=w4480:dbl)
            n1194 = Wait (ms)(milliseconds to wait=w4480) -> ()  [unwired: 1 out]
          }
          frame #1 {
            n1195 = property on="Green laser mode" class="RadioBtnsControl (strict)"("Val(Sgnl)"=enum32{"Laser ON", "Laser OFF", "Interlace"}."Interlace" ("Value (Signaling)")) -> ()  [unwired: 2 in, 2 out]
          }
        }
      }
      event #10 {
        w4504 = i16 1 ("f")
        n1196 = event-data() -> ()  [unwired: 7 out]
        n1197 = local write "Trap 1 (ON/OFF)"("Trap 1 ON") -> ()
        n1198 = local write "Trap 2 (ON/OFF)"("Trap 2 ON") -> ()
        n1199 = Boolean To (0,1)(Boolean="Trap 3 ON") -> (0, 1=w4505:i16)
        n1200 = Boolean To (0,1)(Boolean="Trap 1 ON") -> (0, 1=w4506:i16)
        n1201 = Boolean To (0,1)(Boolean="Trap 2 ON") -> (0, 1=w4507:i16)
        n1202 = Select(t=w4507, s="Trap ON/OFF X or Y Amp?", f=w4504) -> (s? t:f=w4502:i16)
        n1203 = Select(t=w4506, s="Trap ON/OFF X or Y Amp?", f=w4504) -> (s? t:f=w4503:i16)
        n1204 = Select(t=w4505, s="Trap ON/OFF X or Y Amp?", f=w4504) -> (s? t:f=w4501:i16)
        n1205 = Select(t=w4504, s="Trap ON/OFF X or Y Amp?", f=w4507) -> (s? t:f=w4499:i16)
        n1206 = Select(t=w4504, s="Trap ON/OFF X or Y Amp?", f=w4506) -> (s? t:f=w4500:i16)
        n1207 = Select(t=w4504, s="Trap ON/OFF X or Y Amp?", f=w4505) -> (s? t:f=w4498:i16)
        n1208 = And(x="All FB On/Off", y="Feedback On/Off") -> (x .and. y?=w4496:cluster{"Set 1":bool, "Set 2":bool})
        n1209 = local read "BD 1 Amplitude 1 (%)"() -> (w4516:dbl)
        n1210 = local read "BD 1 Amplitude 2 (%)"() -> (w4515:dbl)
        n1211 = local read "BD 1 Amplitude 3 (%)"() -> (w4514:dbl)
        n1212 = Unbundle By Name(w4496) -> ("Set 1"=w4491:bool, "Set 2"=w4488:bool)
        n1213 = local read "Y RF Amplitude Limits (%)"() -> (w4484:T12)
        n1214 = local read "X RF Amplitude Limits (%)"() -> (w4485:T12)
        n1215 = local read "BD 2 Amplitude 1 (%)"() -> (w4517:dbl)
        n1216 = local read "BD 2 Amplitude 2 (%)"() -> (w4518:dbl)
        n1217 = local read "BD 2 Amplitude 3 (%)"() -> (w4519:dbl)
        n1218 = And(x="Trap 2 ON", y=w4488) -> (x .and. y?=w4486:bool)
        n1219 = And(x="Trap 1 ON", y=w4491) -> (x .and. y?=w4489:bool)
        n1220 = Multiply(x=w4503, y=w4516) -> (x*y=w4511:dbl)
        n1221 = Multiply(x=w4515, y=w4502) -> (x*y=w4509:dbl)
        n1222 = Multiply(x=w4514, y=w4501) -> (x*y=w4510:dbl)
        n1223 = Multiply(x=w4517, y=w4500) -> (x*y=w4520:dbl)
        n1224 = Multiply(x=w4518, y=w4499) -> (x*y=w4521:dbl)
        n1225 = Multiply(x=w4519, y=w4498) -> (x*y=w4522:dbl)
        n1226 = call "set RF board amplitude - interlace.vi"("Board 2 Amplitude Limits"=w4484, "Board 1 Amplitude Limits"=w4485, "error in"=w4512, "FPGA VI Reference In"=w4513, "Board 2 Amplitude 3 (%)"=w4522, "Board 1 Amplitude 3 (%)"=w4510, "Board 2 Amplitude 2 (%)"=w4521, "Board 2 Amplitude 1 (%)"=w4520, "Board 1 Amplitude 2 (%)"=w4509, "Board 1 Amplitude 1 (%)"=w4511) -> ("error out"=w4493:errorcluster, "FPGA VI Reference Out"=w4494:T15)
        n1227 = xnode "Read/Write Control"("FPGA VI Reference In"=w4494, "error in"=w4493, "FB On/Off Set 1"=w4489, "FB On/Off Set 2"=w4486) -> ("error out"=w4492:errorcluster)  [unwired: 1 out]
      }
      event #11 {
        n1228 = event-data() -> ()  [unwired: 7 out]
        n1229 = property on="Saved AOD Raster Scan Parameter Sets" class="Arr (strict)"() -> ("Index Values"=w4589:u32[])  [unwired: 2 in, 2 out]
        n1230 = Index Array(array=w4589, index=0) -> (element=w4586:u32)
        n1231 = Index Array(array="Saved AOD Raster Scan Parameter Sets", index=w4586) -> (element=w4585:T40)
        n1232 = Unbundle By Name(w4585) -> ("Scan Range AOD (nm) 2"=w4584:dbl, "Step Size AOD (nm) 2"=w4583:dbl, "Scan Speed AOD (nm/s) 2"=w4582:dbl, "Number of scans (AOD) 2"=w4581:u16)
        n1233 = flat-sequence {
          tunnel: w4584 -> [w4593]
          tunnel: w4583 -> [w4592]
          tunnel: w4582 -> [w4591]
          tunnel: w4581 -> [w4594]
          frame #0 {
            n1234 = local write "Scan Speed (nm/s)"(w4591) -> ()
            n1235 = local write "Scan Range (nm)"(w4593) -> ()
            n1236 = local write "Step Size (nm)"(w4592) -> ()
          }
          frame #1 {
            n1237 = property on="Number of F/B Scans (AOD)" class="DigNum (strict)"("Val(Sgnl)"=w4594) -> ()  [unwired: 2 in, 2 out]
          }
        }
      }
      event #12 {
        n1238 = event-data() -> ()  [unwired: 7 out]
        n1239 = property on="Trap 2 ON" class="Bool (strict)"("Val(Sgnl)"="Trap 2 (ON/OFF)") -> ()  [unwired: 2 in, 2 out]
        n1240 = property on="Trap 1 ON" class="Bool (strict)"("Val(Sgnl)"="Trap 1 (ON/OFF)") -> ()  [unwired: 2 in, 2 out]
      }
      event #13 {
        n1241 = event-data() -> ()  [unwired: 7 out]
        n1242 = local read "DIO count 3 (ticks)"() -> (w4607:u32)
        n1243 = local read "DIO count 1 (ticks)"() -> (w4609:u32)
        n1244 = local read "DIO count 2 (ticks)"() -> (w4608:u32)
        n1245 = To Unsigned Byte Integer(number="Not-Interlacing Set") -> (unsigned 8bit integer=w4598:u8)
        n1246 = Add(x=w4598, y=u8 1) -> (x+y=w4602:u8)
        n1247 = xnode "Read/Write Control"("FPGA VI Reference In"=w4613, "error in"=w4611, "DIO count 1 (ticks)"=w4609, "DIO count 2 (ticks)"=w4608, "DIO count 3 (ticks)"=w4607, "Interlace ON/OFF"="Interlace", "Number Interlace Cycles"="Number Interlace Sets", "Interlace Off Parameters"=w4602) -> ("error out"=w4612:errorcluster)  [unwired: 1 out]
        n1248 = Build Array(w4609, w4608, w4607) -> (w4600:u32[])
        n1249 = Split 1D Array(array=w4600, index="Number Interlace Sets") -> (first subarray=w4610:u32[])  [unwired: 1 out]
        n1250 = Index Array(array=w4600, index=w4598) -> (element=w4599:u32)
        n1251 = Add Array Elements(numeric array=w4610) -> (sum=w4604:u32)
        n1252 = Select(t=w4604, s="Interlace", f=w4599) -> (s? t:f=→"Total Counts (ticks)":u32)
      }
      event #14 {
        n1253 = event-data() -> ()  [unwired: 7 out]
        n1254 = Unbundle By Name("Reset Feedback") -> ("Set 1"=w4749:bool, "Set 2"=w4748:bool)
        n1255 = xnode "Read/Write Control"("FPGA VI Reference In"=w4751, "error in"=w4746, "FB Reset Set 1"=w4749, "FB Reset Set 2"=w4748) -> ("error out"=w4747:errorcluster)  [unwired: 1 out]
      }
      event #15 {
        n1256 = event-data() -> ()  [unwired: 7 out]
        n1257 = Unbundle By Name("PID Gains") -> ("Set 1"=w4812:T10, "Set 2"=w4811:T10)
        n1258 = xnode "Read/Write Control"("FPGA VI Reference In"=w4813, "error in"=w4809, "FB Gains Set 1"=w4812, "FB Gains Set 2"=w4811) -> ("error out"=w4810:errorcluster)  [unwired: 1 out]
      }
      event #16 {
        n1259 = event-data() -> ()  [unwired: 7 out]
        n1260 = xnode "Read/Write Control"("FPGA VI Reference In"=w4856, "error in"=w4852) -> ("FPGA VI Reference Out"=w4855:T15, "error out"=w4854:errorcluster, "AI2 Y Sum Set 1"=w4863:i16, "AI2 Y Sum Set 2"=w4862:i16)
        n1261 = Cluster To Array(cluster="AI2 to Setpoint") -> (array=w4866:bool[])
        n1262 = local read "AI2 (V)"() -> (w4864:cluster{"Set 1":dbl, "Set 2":dbl})
        n1263 = Or Array Elements(Boolean array=w4866) -> (logical OR=w4867:bool)
        n1264 = Bundle By Name(cluster=w4864, "Set 1"=w4863, "Set 2"=w4862) -> (w4861:cluster{"Set 1":dbl, "Set 2":dbl})
        n1265 = Divide(x=w4861, y=3276.7) -> (x/y=w4860:cluster{"Set 1":dbl, "Set 2":dbl})
        "AI2 (V)" <- w4860
        n1266 = case shown="True" w4867 {
          tunnel: [w4929 w4946] -> w4859
          tunnel: "AI2 to Setpoint" -> [_ w4942]
          tunnel: "Setpoints (V)" -> [w4930 w4945]
          tunnel: w4860 -> [_ w4939]
          frame #0 {
            n1267 = Multiply(x=3276.7, y=w4930) -> (x*y=w4931:cluster{"Set 1":dbl, "Set 2":dbl})
            n1268 = To Word Integer(number=w4931) -> (16bit integer=w4929:cluster{"Set 1":i16, "Set 2":i16})
          }
          frame #1 {
            n1269 = Unbundle By Name(w4939) -> ("Set 1"=w4938:dbl, "Set 2"=w4937:dbl)
            n1270 = Unbundle By Name(w4945) -> ("Set 1"=w4944:dbl, "Set 2"=w4943:dbl)
            n1271 = Unbundle By Name(w4942) -> ("Set 1"=w4941:bool, "Set 2"=w4940:bool)
            n1272 = Select(t=w4938, s=w4941, f=w4944) -> (s? t:f=w4936:dbl)
            n1273 = Select(t=w4937, s=w4940, f=w4943) -> (s? t:f=w4935:dbl)
            n1274 = Bundle By Name(cluster=w4945, "Set 1"=w4936, "Set 2"=w4935) -> (w4933:cluster{"Set 1":dbl, "Set 2":dbl})
            n1275 = Multiply(x=3276.7, y=w4933) -> (x*y=w4934:cluster{"Set 1":dbl, "Set 2":dbl})
            n1276 = local write "Setpoints (V)"(w4933) -> ()
            n1277 = To Word Integer(number=w4934) -> (16bit integer=w4946:cluster{"Set 1":i16, "Set 2":i16})
          }
        }
        n1278 = Unbundle By Name(w4859) -> ("Set 1"=w4858:i16, "Set 2"=w4857:i16)
        n1279 = xnode "Read/Write Control"("FPGA VI Reference In"=w4855, "error in"=w4854, "FB Setpoint Set 1"=w4858, "FB Setpoint Set 2"=w4857) -> ("error out"=w4853:errorcluster)  [unwired: 1 out]
      }
      event #17 {
        n1280 = event-data() -> ()  [unwired: 7 out]
        n1281 = xnode "Read/Write Control"("FPGA VI Reference In"=w5006, "error in"=w5004, "Invert GI"="Invert GI", "Invert GI 2"="Invert GI") -> ("error out"=w5005:errorcluster)  [unwired: 1 out]
      }
      event #18 {
        n1282 = event-data() -> ()  [unwired: 7 out]
        n1283 = local read "Green FB Setpoint (mV)"() -> (w5070:dbl)
        n1284 = local read "Current When FB OFF (%)"() -> (w5073:dbl)
        n1285 = Multiply(x=w5070, y=3.2767) -> (x*y=w5069:dbl)
        n1286 = Multiply(x=w5073, y=655.35) -> (x*y=w5074:dbl)
        n1287 = To Unsigned Word Integer(number=w5074) -> (unsigned 16bit integer=w5072:u16)
        n1288 = local read "Green int current ON count adj"() -> (w5077:u32)
        n1289 = local read "Green FB Gains"() -> (w5076:T10)
        n1290 = local read "Green Laser ON/Interlacing"() -> (w5067:bool)
        n1291 = local read "Green laser mode"() -> (w5066:enum32{"Laser ON", "Laser OFF", "Interlace"})
        n1292 = local read "Green FB On/Off"() -> (w5078:bool)
        n1293 = Equal?(x=w5066, y=enum32{"Laser ON", "Laser OFF", "Interlace"}."Interlace") -> (x = y?=w5064:bool)
        n1294 = Compound Arithmetic op=AND(w5064, w5078, w5067) -> (w5068:bool)
        n1295 = xnode "Read/Write Control"("FPGA VI Reference In"=w5081, "error in"=w5080, "Green FB Setpoint"=w5069, "Green FB On/Off"=w5068, "Current Out"=w5072, "Green int current ON count adj"=w5077, "Green FB Gains"=w5076) -> ("error out"=w5079:errorcluster)  [unwired: 1 out]
      }
      event #19 {
        n1296 = event-data() -> ()  [unwired: 7 out]
        n1297 = case shown="True" "Green Laser ON/Interlacing" {
          tunnel: "Green laser mode" -> [_ w5199]
          tunnel: [enum32{"Laser ON", "Laser OFF", "Interlace"}."Laser OFF" ("Green laser mode") w5199] -> w5187
          tunnel: [FALSE w5195] -> w5186
          frame #0 {
          }
          frame #1 {
            n1298 = local read "Green FB On/Off"() -> (w5196:bool)
            n1299 = Equal?(x=w5199, y=enum32{"Laser ON", "Laser OFF", "Interlace"}."Interlace") -> (x = y?=w5197:bool)
            n1300 = And(x=w5197, y=w5196) -> (x .and. y?=w5195:bool)
          }
        }
        n1301 = xnode "Read/Write Control"("FPGA VI Reference In"=w5192, "error in"=w5190, "Operating Mode"=w5187, "Operating Mode 2"=w5187, "Green FB On/Off"=w5186) -> ("error out"=w5191:errorcluster)  [unwired: 1 out]
      }
      event #20 {
        n1302 = event-data() -> ()  [unwired: 7 out]
        n1303 = local read "Phase Adj. (APD 1 Gate)"() -> (w5275:i16)
        n1304 = Negate(x=w5275) -> (-x=w5283:i16)
        n1305 = Select(t=w5283, s="- phase (APD 1 Gate)", f=w5275) -> (s? t:f=w5282:i16)
        n1306 = Or(x="- phase (APD 1 Gate)", y="+ phase (APD 1 Gate)") -> (x .or. y?=w5278:bool)
        n1307 = xnode "Read/Write Control"("FPGA VI Reference In"=w5285, "error in"=w5284, "Phase count adjustment (APD 1 Gate)"=w5282) -> ("FPGA VI Reference Out"=w5280:T15, "error out"=w5281:errorcluster)
        n1308 = xnode "Read/Write Control"("FPGA VI Reference In"=w5280, "error in"=w5281, "+ phase (APD 1 Gate)"=w5278) -> ("error out"=w5279:errorcluster)  [unwired: 1 out]
      }
      event #21 {
        n1309 = event-data() -> ()  [unwired: 7 out]
        n1310 = local read "Phase Adj. (APD 2 Gate)"() -> (w5359:i16)
        n1311 = Negate(x=w5359) -> (-x=w5367:i16)
        n1312 = Select(t=w5367, s="- phase (APD 2 Gate)", f=w5359) -> (s? t:f=w5366:i16)
        n1313 = Or(x="- phase (APD 2 Gate)", y="+ phase (APD 2 Gate)") -> (x .or. y?=w5362:bool)
        n1314 = xnode "Read/Write Control"("FPGA VI Reference In"=w5369, "error in"=w5368, "Phase count adjustment (APD 2 Gate)"=w5366) -> ("FPGA VI Reference Out"=w5364:T15, "error out"=w5365:errorcluster)
        n1315 = xnode "Read/Write Control"("FPGA VI Reference In"=w5364, "error in"=w5365, "+ phase (APD 2 Gate)"=w5362) -> ("error out"=w5363:errorcluster)  [unwired: 1 out]
      }
      event #22 {
        n1316 = event-data() -> ()  [unwired: 7 out]
        n1317 = local read "Phase Adj. (APD Acq)"() -> (w5445:i16)
        n1318 = Negate(x=w5445) -> (-x=w5451:i16)
        n1319 = Select(t=w5451, s="+ phase (APD Acq)", f=w5445) -> (s? t:f=w5450:i16)
        n1320 = Or(x="+ phase (APD Acq)", y="- phase (APD Acq)") -> (x .or. y?=w5446:bool)
        n1321 = xnode "Read/Write Control"("FPGA VI Reference In"=w5453, "error in"=w5452, "Phase Count Adjustment (APD Acq)"=w5450) -> ("FPGA VI Reference Out"=w5448:T15, "error out"=w5449:errorcluster)
        n1322 = xnode "Read/Write Control"("FPGA VI Reference In"=w5448, "error in"=w5449, "+ phase (APD Acq)"=w5446) -> ("error out"=w5447:errorcluster)  [unwired: 1 out]
      }
      event #23 {
        n1323 = event-data() -> ()  [unwired: 7 out]
        n1324 = Negate(x="Phase adj. (GI)") -> (-x=w5535:i16)
        n1325 = Select(t=w5535, s="+ phase (GI)", f="Phase adj. (GI)") -> (s? t:f=w5534:i16)
        n1326 = Or(x="+ phase (GI)", y="- phase (GI)") -> (x .or. y?=w5530:bool)
        n1327 = xnode "Read/Write Control"("FPGA VI Reference In"=w5537, "error in"=w5536, "Phase count adjustment (GI)"=w5534) -> ("FPGA VI Reference Out"=w5532:T15, "error out"=w5533:errorcluster)
        n1328 = xnode "Read/Write Control"("FPGA VI Reference In"=w5532, "error in"=w5533, "+ phase (GI)"=w5530) -> ("error out"=w5531:errorcluster)  [unwired: 1 out]
      }
      event #24 {
        n1329 = event-data() -> ()  [unwired: 7 out]
        n1330 = Negate(x="Phase adj. (GI) 2") -> (-x=w5619:i16)
        n1331 = Select(t=w5619, s="+ phase (GI) 2", f="Phase adj. (GI) 2") -> (s? t:f=w5618:i16)
        n1332 = Or(x="+ phase (GI) 2", y="- phase (GI) 2") -> (x .or. y?=w5614:bool)
        n1333 = xnode "Read/Write Control"("FPGA VI Reference In"=w5621, "error in"=w5620, "Phase count adjustment (GI) 2"=w5618) -> ("FPGA VI Reference Out"=w5616:T15, "error out"=w5617:errorcluster)
        n1334 = xnode "Read/Write Control"("FPGA VI Reference In"=w5616, "error in"=w5617, "+ phase (GI) 2"=w5614) -> ("error out"=w5615:errorcluster)  [unwired: 1 out]
      }
      event #25 {
        n1335 = event-data() -> ()  [unwired: 7 out]
        n1336 = Negate(x="Phase adj. (Green FB)") -> (-x=w5703:i16)
        n1337 = Select(t=w5703, s="+ phase (Green FB)", f="Phase adj. (Green FB)") -> (s? t:f=w5702:i16)
        n1338 = Or(x="+ phase (Green FB)", y="- phase (Green FB)") -> (x .or. y?=w5698:bool)
        n1339 = xnode "Read/Write Control"("FPGA VI Reference In"=w5705, "error in"=w5704, "Phase count adjustment (Green FB)"=w5702) -> ("FPGA VI Reference Out"=w5700:T15, "error out"=w5701:errorcluster)
        n1340 = xnode "Read/Write Control"("FPGA VI Reference In"=w5700, "error in"=w5701, "+ phase (Green FB)"=w5698) -> ("error out"=w5699:errorcluster)  [unwired: 1 out]
      }
      event #26 {
        n1341 = event-data() -> ()  [unwired: 7 out]
        n1342 = local read "APD Integration Time (s)"() -> (w5779:dbl)
        n1343 = local read "APD Gate ON Count"() -> (w5794:u32)
        n1344 = local read "APD Gate OFF Count"() -> (w5793:u32)
        n1345 = local read "Invert APD Gate"() -> (w5795:bool)
        n1346 = local read "APD Gate"() -> (w5792:enum32{"ON", "OFF", "Interlace"})
        n1347 = Multiply(x=w5779, y=40000000.0) -> (x*y=w5790:dbl)
        n1348 = Reciprocal(x=w5779) -> (1/x=→"APD Acq Rate (Hz)":dbl)
        n1349 = To Unsigned Long Integer(number=w5790) -> (unsigned 32bit integer=w5789:u32)
        n1350 = local read "DMA Update Period (s)"() -> (w5780:dbl)
        n1351 = Divide(x=w5780, y=w5779) -> (x/y=w5783:dbl)
        n1352 = local read "APD 1 AO offset"() -> (w5785:i16)
        n1353 = local read "APD 1 AO Mult."() -> (w5787:i16)
        n1354 = local read "APD 2 AO Mult."() -> (w5786:i16)
        n1355 = local read "APD 2 AO offset"() -> (w5784:i16)
        n1356 = Multiply(x=2.0, y=w5783) -> (x*y=w5782:dbl)
        n1357 = local write "APD Samples/FIFO Acq."(w5783) -> ()
        n1358 = local write "APD Elements/DMA read"(w5782) -> ()
        n1359 = xnode "Read/Write Control"("FPGA VI Reference In"=w5798, "error in"=w5797, "Invert APD Gate"=w5795, "APD Gate ON Count"=w5794, "APD Gate OFF Count"=w5793, "APD Acq Rate Count"=w5789, "APD Gate Operating Mode"=w5792, "APD 1 AO scale factor"=w5787, "APD 2 AO scale factor"=w5786, "APD 1 AO offset"=w5785, "APD 2 AO offset"=w5784) -> ("error out"=w5796:errorcluster)  [unwired: 1 out]
      }
      event #27 {
        n1360 = event-data() -> ()  [unwired: 7 out]
        n1361 = xnode "Read/Write Control"("FPGA VI Reference In"=w5993, "error in"=w5991, "Green interlace ON count"="GI Frequency, ON count", "Green interlace OFF count"="GI Frequency, OFF count", "Green interlace ON count 2"="GI Frequency, ON count", "Green interlace OFF count 2"="GI Frequency, OFF count", "Green FB Count"="Green FB Count") -> ("error out"=w5992:errorcluster)  [unwired: 1 out]
      }
      event #28 {
        w6161 = 123.0  # AOM cal (nm/MHz)
        n1362 = event-data() -> ()  [unwired: 7 out]
        n1363 = local read "BD 1 Frequency 1 (MHz)"() -> (w6144:dbl)
        n1364 = local read "AOM X Cal (nm/MHz)"() -> (w6136:dbl)
        n1365 = local read "X RF Frequency Limits (MHz)"() -> (w6148:T12)
        n1366 = local read "Y RF Frequency Limits (MHz)"() -> (w6145:T12)
        n1367 = local read "BD 2 Frequency 1 (MHz)"() -> (w6150:dbl)
        n1368 = Negate(x="Scan Range (nm)") -> (-x=w6113:dbl)
        n1369 = Divide(x=w6113, y=w6136) -> (x/y=w6117:dbl)
        n1370 = Select(t=w6148, s="Scan BD", f=w6145) -> (s? t:f=w6147:T12)
        n1371 = Select(t=w6144, s="Scan BD", f=w6150) -> (s? t:f=w6149:dbl)
        n1372 = Unbundle By Name(w6147) -> ("Maximum"=w6156:dbl, "Minimum"=w6155:dbl)
        n1373 = Add(x=w6117, y=w6149) -> (x+y=w6153:dbl)
        n1374 = Divide(x=w6113, y="Step Size (nm)") -> (x/y=w6133:dbl)
        n1375 = Divide(x="Step Size (nm)", y=w6136) -> (x/y=w6142:dbl)
        n1376 = Absolute Value(x=w6133) -> (abs(x)=w6116:dbl)
        n1377 = Sign(1:w6113) -> (0:w6114:dbl)
        n1378 = In Range and Coerce(upper limit=w6156, x=w6153, lower limit=w6155) -> (coerced(x)=w6152:dbl, In Range?=w6154:bool)
        n1379 = To Unsigned Quad Integer(1:w6116) -> (0:w6132:u64)
        "Scan steps (AOD)" <- w6132
        n1380 = call "IR AOM freq to word.vi"("Frequency In (MHz)"=w6142) -> ("Frequency Word Out (double)"=w6139:dbl)
        n1381 = Multiply(x=w6114, y=w6139) -> (x*y=w6115:dbl)
        n1382 = Subtract(x=w6153, y=w6152) -> (x-y=w6151:dbl)
        n1383 = To Quad Integer(1:w6115) -> (0:w6138:i64)
        "Incr. int (AOD)" <- w6138
        n1384 = Subtract(x=w6117, y=w6151) -> (x-y=w6137:dbl)
        "Scan Range (MHz)" <- w6137
        n1385 = Select(t=w6117, s=w6154, f=w6137) -> (s? t:f=w6157:dbl)
        n1386 = Multiply(x=w6137, y=w6136) -> (x*y=w6135:dbl)
        n1387 = Decrement(x=w6132) -> (x-1=w6185:u64)
        n1388 = Negate(x=w6135) -> (-x=w6131:dbl)
        n1389 = local write "Scan Range (nm)"(w6131) -> ()
        n1390 = Divide(x=w6157, y=w6185) -> (x/y=w6141:dbl)
        "Scan Increment (MHz)" <- w6141
        n1391 = call "IR AOM freq to word.vi"("Frequency In (MHz)"=w6141) -> ("Frequency Word Out (double)"=w6140:dbl)
        n1392 = Divide(x="Step Size (nm)", y="Scan Speed (nm/s)") -> (x/y=w6128:dbl)
        n1393 = To Quad Integer(1:w6140) -> ()  [unwired: 1 out]
        n1394 = local read "Number Interlace Sets"() -> (w6111:u8)
        n1395 = local read "AI Count (ticks)"() -> (w6112:u32)
        n1396 = local read "Total Counts (ticks)"() -> (w6110:u32)
        n1397 = local read "# Samples/trap"() -> (w6143:dbl)
        n1398 = Multiply(x=w6112, y=w6111) -> (x*y=w6109:u32)
        n1399 = Divide(x=w6110, y=w6109) -> (x/y=w6108:dbl)
        n1400 = Select(t=w6144, s="Scan BD", f=w6150) -> (s? t:f=w6182:dbl)
        "Initial freq. (MHz)" <- w6182
        n1401 = Add(x=w6157, y=w6182) -> (x+y=→"Final freq. (MHz)":dbl)
        n1402 = Divide(x=w6110, y=40000000.0) -> (x/y=w6127:dbl)
        n1403 = Divide(x=w6128, y=w6127) -> (x/y=w6126:dbl)
        n1404 = To Unsigned Quad Integer(1:w6126) -> (0:w6125:u64)
        "Cycles/step (AOD)" <- w6125
        n1405 = xnode "Read/Write Control"("FPGA VI Reference In"=w6193, "error in"=w6192, "Scan steps"=w6132, "Number of scans"="Number of F/B Scans (AOD)", "Cycles per step"=w6125, "Scan freq.  increment"=w6138, "Scan BD"="Scan BD") -> ("error out"=w6191:errorcluster)  [unwired: 1 out]
        n1406 = Multiply(x=w6132, y=w6125) -> (x*y=w6186:u64)
        n1407 = Multiply(x=w6186, y=u64 2) -> (x*y=w6107:u64)
        n1408 = Multiply(x=w6108, y=w6107) -> (x*y=w6106:dbl)
        "Data points/scan (f/b)" <- w6106
        n1409 = Multiply(x=w6106, y="Number of F/B Scans (AOD)") -> (x*y=w6189:dbl)
        "Data points/scans" <- w6189
        n1410 = Divide(x=w6189, y=w6143) -> (x/y=→"N sets should be saved":dbl)
        n1411 = Multiply(x=w6186, y=w6127) -> (x*y=w6124:dbl)
        "Time/Scan (s) (AOD)" <- w6124
        n1412 = Select(t=w6157, s="Scan BD", f=0.0) -> (s? t:f=w6183:dbl)
        n1413 = Select(t=0.0, s="Scan BD", f=w6157) -> (s? t:f=w6179:dbl)
        n1414 = local read "BD 2 Frequency 2 (MHz)"() -> (w6175:dbl)
        n1415 = local read "BD 1 Frequency 2 (MHz)"() -> (w6178:dbl)
        n1416 = Add(x=w6179, y=w6150) -> (x+y=w6176:dbl)
        n1417 = Add(x=w6144, y=w6183) -> (x+y=w6177:dbl)
        n1418 = Multiply(x=w6124, y=2.0) -> (x*y=w6123:dbl)
        n1419 = Multiply(x=w6123, y="Number of F/B Scans (AOD)") -> (x*y=w6120:dbl)
        n1420 = Divide(x=w6120, y=60.0) -> (x/y=→"Time to Finish All (min)":dbl)
        n1421 = Add(x="Trap 2 Bead Size (nm)", y="Trap 1 Bead Size (nm)") -> (x+y=w6165:dbl)
        n1422 = Divide(x=w6165, y=2.0) -> (x/y=w6159:dbl)
        n1423 = Subtract(x=w6176, y=w6175) -> (x-y=w6173:dbl)
        n1424 = Subtract(x=w6177, y=w6178) -> (x-y=w6174:dbl)
        n1425 = local read "Initial delta (MHz)"() -> (w6162:dbl)
        n1426 = Square(x=w6173) -> (x^2=w6172:dbl)
        n1427 = Square(x=w6174) -> (x^2=w6171:dbl)
        n1428 = Add(x=w6171, y=w6172) -> (x+y=w6170:dbl)
        n1429 = Square Root(x=w6170) -> (sqrt(x)=w6169:dbl)
        "Final delta (MHz)" <- w6169
        n1430 = Multiply(x=w6161, y=w6169) -> (x*y=w6168:dbl)
        n1431 = Multiply(x=w6162, y=w6161) -> (x*y=w6160:dbl)
        n1432 = Subtract(x=w6160, y=w6159) -> (x-y=→"Initial sep (nm)":dbl)
        n1433 = Subtract(x=w6168, y=w6159) -> (x-y=→"Final sep (nm)":dbl)
      }
      event #29 {
        n1434 = event-data() -> ()  [unwired: 7 out]
        n1435 = local read "Freq or Amp switch first"() -> (w6280:bool)
        n1436 = local read "Amp switch delay"() -> (w6281:u16)
        n1437 = local read "Freq switch delay"() -> (w6283:u16)
        n1438 = local read "Swap F1 and F2"() -> (w6282:bool)
        n1439 = xnode "Read/Write Control"("FPGA VI Reference In"=w6286, "error in"=w6285, "Freq switch delay"=w6283, "Swap F1 and F2"=w6282, "Amp switch delay"=w6281, "Freq or Amp switch first"=w6280) -> ("error out"=w6284:errorcluster)  [unwired: 1 out]
      }
      event #30 {
        w6383 = 32767.0 ("y")
        n1440 = event-data() -> ()  [unwired: 7 out]
        n1441 = Select(t="Scan lines (y)", s="2D or 1D Scan", f="Number of scans (MCL)") -> (s? t:f=w6388:u64)
        n1442 = Decrement(x="Scan steps (MCL)") -> (x-1=w6404:u64)
        n1443 = Divide(x="Scan Range (V)\n(of steps)", y=w6404) -> (x/y=w6403:dbl)
        "Desired Scan Incr (V)" <- w6403
        n1444 = local read "APD Integration Time (s)"() -> (w6396:dbl)
        n1445 = Multiply(x=w6403, y=w6383) -> (x*y=w6412:dbl)
        n1446 = Divide(x=w6412, y=10.0) -> (x/y=w6402:dbl)
        "Desired incr (int)" <- w6402
        n1447 = local read "Update Count (MCL)"() -> (w6408:u32)
        n1448 = Round Toward -Infinity(1:w6402) -> (0:w6411:dbl)
        n1449 = To Word Integer(number=w6411) -> (16bit integer=w6386:i16)
        "Actual Incr. int (MCL)" <- w6386
        n1450 = Multiply(x=w6396, y=40000000.0) -> (x*y=w6409:dbl)
        n1451 = Divide(x=w6409, y=w6408) -> (x/y=w6407:dbl)
        n1452 = Multiply(x=i16 10, y=w6386) -> (x*y=w6384:i16)
        n1453 = Multiply(x="N APD Samp/step", y=w6407) -> (x*y=w6406:dbl)
        "Cycles/step (MCL)" <- w6406
        n1454 = Divide(x=w6384, y=w6383) -> (x/y=→"Actual MCL Inc (V)":dbl)
        n1455 = Multiply(x="N APD Samp/step", y="Scan steps (MCL)") -> (x*y=w6398:dbl)
        n1456 = local read "APD Samples/FIFO Acq."() -> (w6395:dbl)
        n1457 = Multiply(x=w6398, y=u64 2) -> (x*y=w6397:dbl)
        "Data points/scan (f+b)" <- w6397
        n1458 = Multiply(x=w6397, y=w6388) -> (x*y=w6415:dbl)
        "Data points/scans (MCL)" <- w6415
        n1459 = Multiply(x=w6396, y=w6397) -> (x*y=w6389:dbl)
        "Time/f+b scan (s) (MCL)" <- w6389
        n1460 = Divide(x=w6415, y=w6395) -> (x/y=→"N sets should be saved (MCL)":dbl)
        n1461 = Multiply(x=w6389, y=w6388) -> (x*y=→"Total Time (s)":dbl)
        n1462 = Not(x="Fast Scan Dir") -> (.not. x?=w6393:bool)
        n1463 = xnode "Read/Write Control"("FPGA VI Reference In"=w6419, "error in"=w6418, "Scan steps (MCL)"="Scan steps (MCL)", "Number of scans (MCL)"=w6388, "Cycles per step (MCL)"=w6406, "Scan freq.  increment (MCL)"=w6386, "1D or 2D Scan?"="2D or 1D Scan", "MCL Scan Axis"=w6393, "Cont. Scan (MCL)"="Continuous MCL Scanning") -> ("error out"=w6417:errorcluster)  [unwired: 1 out]
      }
      event #31 {
        w6556 = 1000.0 ("y")
        n1464 = event-data() -> ()  [unwired: 7 out]
        n1465 = local read "Save file name"() -> (w6581:path)
        n1466 = local write "Read Cal"(FALSE ("Read Cal")) -> ()
        n1467 = Strip Path(path=w6581) -> (stripped path=w6580:path)  [unwired: 1 out]
        n1468 = Path To String(path=w6580) -> (string=w6579:string)
        n1469 = Concatenate Strings(w6579, "\\current.cal" ("string")) -> (w6577:string)
        n1470 = String To Path(string=w6577) -> (path=w6576:path)
        n1471 = Open/Create/Replace File(file path (use dialog)=w6576, operation (0:open)=T29."open", access (0:read/write)=enum16{"read/write", "read-only", "write-only"}."read-only") -> (refnum out=w6584:refnum<file>, error out=w6570:errorcluster)  [unwired: 1 in, 3 out]
        n1472 = Deny Access(4:w6570, 7:w6584) -> (0:w6569:errorcluster, 3:w6575:refnum<file>)  [unwired: 1 out]
        n1473 = Read from Binary File(5:0.0, 8:w6569, 9:T30."big-endian, network order" ("byte order (0:big-endian, network order)"), 10:-1 ("count (1)"), 11:w6575) -> (0:w6568:errorcluster, 2:w6566:dbl[], 3:w6571:refnum<file>)  [unwired: 2 out]
        n1474 = Array To Cluster(array=w6566) -> (cluster=w6565:T41)
        n1475 = Unbundle(w6565) -> ("[0]"=w6564:dbl, "[1]"=w6563:dbl, "[2]"=w6562:dbl, "[3]"=w6561:dbl, "[4]"=w6560:dbl, "[5]"=w6559:dbl)
        n1476 = Close File(refnum=w6571, error in=w6568) -> (error out=→"Read cal error":errorcluster)  [unwired: 1 out]
        n1477 = Multiply(x=w6559, y=w6556) -> (x*y=w6557:dbl)
        n1478 = local write "T2 kappa_x (pN/nm)"(w6561) -> ()
        n1479 = local write "T1 kappa_x (pN/nm)"(w6562) -> ()
        n1480 = local write "T1 alpha_x (nm/V)"(w6564) -> ()
        n1481 = local write "T2 alpha_x (nm/V)"(w6563) -> ()
        n1482 = Multiply(x=w6560, y=w6556) -> (x*y=w6558:dbl)
        n1483 = local write "T1 offset_x (mV)"(w6558) -> ()
        n1484 = local write "T2 offset_x (mV)"(w6557) -> ()
      }
      event #32 {
        n1485 = event-data() -> ()  [unwired: 7 out]
        n1486 = local write "MCL Scanning"(FALSE ("MCL Scanning")) -> ()
        n1487 = xnode "Read/Write Control"("FPGA VI Reference In"=w6589, "error in"=w6588, "Abort scan (MCL)"="Abort MCL Scan") -> ("error out"=w6587:errorcluster)  [unwired: 1 out]
      }
      event #33 {
        n1488 = event-data() -> ()  [unwired: 7 out]
        n1489 = xnode "Read/Write Control"("FPGA VI Reference In"=w6630, "error in"=w6629, "MCL count"="Update Count (MCL)") -> ("error out"=w6628:errorcluster)  [unwired: 1 out]
      }
      event #34 {
        n1490 = event-data() -> ()  [unwired: 7 out]
        n1491 = Negate(x="Phase adjust (MCL)") -> (-x=w6675:i16)
        n1492 = Select(t=w6675, s="- phase (MCL)", f="Phase adjust (MCL)") -> (s? t:f=w6673:i16)
        n1493 = Or(x="- phase (MCL)", y="+ phase (MCL)") -> (x .or. y?=w6668:bool)
        n1494 = xnode "Read/Write Control"("FPGA VI Reference In"=w6677, "error in"=w6676, "Phase count adjustment (MCL)"=w6673) -> ("FPGA VI Reference Out"=w6669:T15, "error out"=w6670:errorcluster)
        n1495 = xnode "Read/Write Control"("FPGA VI Reference In"=w6669, "error in"=w6670, "+ phase (MCL)"=w6668) -> ("error out"=w6667:errorcluster)  [unwired: 1 out]
      }
      event #35 {
        n1496 = event-data() -> ()  [unwired: 7 out]
        n1497 = xnode "Read/Write Control"("FPGA VI Reference In"=w6754, "error in"=w6753, "Abort scan"="Abort AOD Scan") -> ("error out"=w6752:errorcluster)  [unwired: 1 out]
      }
      event #36 {
        n1498 = event-data() -> ()  [unwired: 7 out]
        n1499 = xnode "Read/Write Control"("FPGA VI Reference In"=w6795, "error in"=w6794, "Cont. Scan"="Continuous AOD Scanning") -> ("error out"=w6793:errorcluster)  [unwired: 1 out]
      }
      event #37 {
        n1500 = event-data() -> ()  [unwired: 7 out]
        n1501 = call "Create new save file.vi"("Insert"="", "Ext"=".dat" ("string"), "Index In"="Index") -> ("Path Out"=→"Save file name":path, "Index Out"=w6833:dbl)
        "Save index" <- w6833
        n1502 = local write "Index"(w6833) -> ()
      }
      event #38 {
        w6848 = 10.0 ("y")
        w6847 = 32767.0 ("y")
        n1503 = event-data() -> ()  [unwired: 7 out]
        n1504 = local read "AO2"() -> (w6846:dbl)
        n1505 = local read "AO1"() -> (w6843:dbl)
        n1506 = Multiply(x=w6843, y=w6847) -> (x*y=w6842:dbl)
        n1507 = Multiply(x=w6846, y=w6847) -> (x*y=w6845:dbl)
        n1508 = Divide(x=w6842, y=w6848) -> (x/y=w6841:dbl)
        n1509 = Divide(x=w6845, y=w6848) -> (x/y=w6844:dbl)
        n1510 = To Word Integer(number=w6841) -> (16bit integer=w6849:i16)
        n1511 = To Word Integer(number=w6844) -> (16bit integer=w6850:i16)
        n1512 = xnode "Read/Write Control"("FPGA VI Reference In"=w6840, "error in"=w6839, "AO1"=w6849, "AO2"=w6850) -> ("error out"=w6838:errorcluster)  [unwired: 1 out]
      }
      event #39 {
        n1513 = local read "Chemyx Syringe Pump Serial Port"() -> (w6906:refnum<visa-resource-name>)
        n1514 = event-data() -> ()  [unwired: 7 out]
        n1515 = local read "Pump write delay (ms)"() -> (w6907:dbl)
        n1516 = case shown="True" "Inject Pump 1" {
          tunnel: w6907 -> [w6914 w6928]
          tunnel: w6906 -> [w6911 w6927]
          frame #0 {
            n1517 = flat-sequence {
              tunnel: w6911 -> [w6915]
              tunnel: [w6915] -> w6912
              tunnel: w6914 -> [_]
              tunnel: [w6918] -> w6913
              tunnel: w6912 -> [w6918]
              tunnel: w6913 -> [w6919]
              tunnel: [w6919] -> w6909
              tunnel: [w6921] -> w6910
              tunnel: w6909 -> [w6921]
              tunnel: w6910 -> [w6923]
              frame #0 {
                n1518 = call "Write to pump.vi"("string"="enter pump1", "VISA resource name"=w6915) -> ()  [unwired: 1 out]
              }
              frame #1 {
                n1519 = Wait (ms)(milliseconds to wait="Pump pause delay (ms)") -> ()  [unwired: 1 out]
              }
              frame #2 {
                n1520 = call "Write to pump.vi"("string"="stop", "VISA resource name"=w6919) -> ()  [unwired: 1 out]
              }
              frame #3 {
                n1521 = Wait (ms)(milliseconds to wait=u32 500) -> ()  [unwired: 1 out]
              }
              frame #4 {
                n1522 = call "Write to pump.vi"("string"="stop", "VISA resource name"=w6923) -> ()  [unwired: 1 out]
              }
            }
          }
          frame #1 {
            n1523 = flat-sequence {
              tunnel: w6927 -> [w6937]
              tunnel: w6928 -> [w6932]
              tunnel: w6928 -> [w6939]
              tunnel: w6927 -> [w6940]
              tunnel: [w6940] -> w6925
              tunnel: [w6942] -> w6926
              tunnel: w6925 -> [w6942]
              tunnel: w6926 -> [w6944]
              frame #0 {
                n1524 = local read "All Pump Parameters"() -> (w6931:T5)
                n1525 = Unbundle By Name(w6931) -> ("Pump 1"=w6938:T42)
                n1526 = call "Set pump parameters.vi"("Pump write delay (ms)"=w6932, "Volume (uL)"="Ch 2 Inject Volume (uL)", "Rate (uL/h)"="Ch 1 Inject Rate (ul/h)", "Units"=4.0, "Pump #"=1.0, "Pump Parameters In"=w6938, "VISA resource name"=w6937) -> ("Pump Parameters Out"=w6930:T42)  [unwired: 3 in]
                n1527 = Bundle By Name(cluster=w6931, "Pump 1"=w6930) -> (w6929:T5)
                n1528 = local write "All Pump Parameters"(w6929) -> ()
              }
              frame #1 {
                n1529 = Wait (ms)(milliseconds to wait=w6939) -> ()  [unwired: 1 out]
              }
              frame #2 {
                n1530 = call "Write to pump.vi"("string"="start", "VISA resource name"=w6940) -> ()  [unwired: 1 out]
              }
              frame #3 {
                n1531 = Wait (ms)(milliseconds to wait=u32 500) -> ()  [unwired: 1 out]
              }
              frame #4 {
                n1532 = call "Write to pump.vi"("string"="start", "VISA resource name"=w6944) -> ()  [unwired: 1 out]
              }
            }
          }
        }
      }
      event #40 {
        n1533 = event-data() -> ()  [unwired: 7 out]
        n1534 = local read "Pump write delay (ms)"() -> (w6947:dbl)
        n1535 = case shown="False" "Inject Pump 3" {
          tunnel: w6947 -> [w6954 w6968]
          tunnel: "Chemyx Syringe Pump Serial Port" -> [w6951 w6967]
          frame #0 {
            n1536 = flat-sequence {
              tunnel: w6951 -> [w6955]
              tunnel: [w6955] -> w6952
              tunnel: w6954 -> [_]
              tunnel: [w6958] -> w6953
              tunnel: w6952 -> [w6958]
              tunnel: w6953 -> [w6959]
              tunnel: [w6959] -> w6949
              tunnel: [w6961] -> w6950
              tunnel: w6949 -> [w6961]
              tunnel: w6950 -> [w6963]
              frame #0 {
                n1537 = call "Write to pump.vi"("string"="enter pump3", "VISA resource name"=w6955) -> ()  [unwired: 1 out]
              }
              frame #1 {
                n1538 = local read "Pump pause delay (ms)"() -> (w6957:u32)
                n1539 = Wait (ms)(milliseconds to wait=w6957) -> ()  [unwired: 1 out]
              }
              frame #2 {
                n1540 = call "Write to pump.vi"("string"="stop", "VISA resource name"=w6959) -> ()  [unwired: 1 out]
              }
              frame #3 {
                n1541 = Wait (ms)(milliseconds to wait=u32 0) -> ()  [unwired: 1 out]
              }
              frame #4 {
                n1542 = call "Write to pump.vi"("string"="stop", "VISA resource name"=w6963) -> ()  [unwired: 1 out]
              }
            }
          }
          frame #1 {
            n1543 = flat-sequence {
              tunnel: w6967 -> [w6977]
              tunnel: w6968 -> [w6972]
              tunnel: w6968 -> [w6979]
              tunnel: w6967 -> [w6980]
              tunnel: [w6980] -> w6965
              tunnel: [w6983] -> w6966
              tunnel: w6965 -> [w6983]
              tunnel: w6966 -> [w6984]
              frame #0 {
                n1544 = local read "All Pump Parameters"() -> (w6971:T5)
                n1545 = Unbundle By Name(w6971) -> ("Pump 3"=w6978:T42)
                n1546 = call "Set pump parameters.vi"("Pump write delay (ms)"=w6972, "Volume (uL)"="Ch 3 Inject Volume (uL)", "Rate (uL/h)"="Ch 3 Inject Rate (ul/h)", "Units"=4.0, "Pump #"=3.0, "Pump Parameters In"=w6978, "VISA resource name"=w6977) -> ("Pump Parameters Out"=w6970:T42)  [unwired: 3 in]
                n1547 = Bundle By Name(cluster=w6971, "Pump 3"=w6970) -> (w6969:T5)
                n1548 = local write "All Pump Parameters"(w6969) -> ()
              }
              frame #1 {
                n1549 = Wait (ms)(milliseconds to wait=w6979) -> ()  [unwired: 1 out]
              }
              frame #2 {
                n1550 = call "Write to pump.vi"("string"="start", "VISA resource name"=w6980) -> ()  [unwired: 1 out]
              }
              frame #3 {
                n1551 = Wait (ms)(milliseconds to wait=u32 500) -> ()  [unwired: 1 out]
              }
              frame #4 {
                n1552 = call "Write to pump.vi"("string"="start", "VISA resource name"=w6984) -> ()  [unwired: 1 out]
              }
            }
          }
        }
      }
      event #41 {
        n1553 = event-data() -> ()  [unwired: 7 out]
        n1554 = local read "Pump write delay (ms)"() -> (w6988:dbl)
        n1555 = flat-sequence {
          tunnel: w6986 -> [w7001]
          tunnel: w6988 -> [w6997]
          tunnel: "Inject Pump 2" -> [_]
          tunnel: w6988 -> [w7003]
          tunnel: w6986 -> [w7004]
          frame #0 {
            n1556 = local read "All Pump Parameters"() -> (w6996:T5)
            n1557 = Multiply(x=60.0, y="Flush Center Ch Rate (ul/m)") -> (x*y=w6993:dbl)
            n1558 = Unbundle By Name(w6996) -> ("Pump 2"=w7002:T42)
            n1559 = call "Set pump parameters.vi"("Pump write delay (ms)"=w6997, "Volume (uL)"="Flush Center Ch Volume (uL)", "Rate (uL/h)"=w6993, "Units"=3.0, "Pump #"=2.0, "Pump Parameters In"=w7002, "VISA resource name"=w7001) -> ("Pump Parameters Out"=w6995:T42)  [unwired: 3 in]
            n1560 = Bundle By Name(cluster=w6996, "Pump 2"=w6995) -> (w6994:T5)
            n1561 = local write "All Pump Parameters"(w6994) -> ()
            n1562 = Add(x="Flush Center Ch Volume (uL)", y="Total Volume\nFlushed (uL)") -> (x+y=w6990:dbl)
            n1563 = local write "Total Volume\nFlushed (uL)"(w6990) -> ()
          }
          frame #1 {
            n1564 = Wait (ms)(milliseconds to wait=w7003) -> ()  [unwired: 1 out]
          }
          frame #2 {
            n1565 = call "Write to pump.vi"("string"="start", "VISA resource name"=w7004) -> ()  [unwired: 1 out]
          }
        }
        n1566 = local read "Chemyx Syringe Pump Serial Port"() -> (w6986:refnum<visa-resource-name>)
      }
      event #42 {
        n1567 = event-data() -> ()  [unwired: 7 out]
        n1568 = Select(t="run" ("string"), s="Sample Channel Flow", f="stop" ("string")) -> (s? t:f=w7006:string)
        n1569 = Concatenate Strings(w7006, "\r") -> (w7010:string)
        n1570 = VISA Write(VISA resource name=w7012, write buffer=w7010) -> ()  [unwired: 1 in, 3 out]
      }
      event #43 {
        n1571 = event-data() -> ()  [unwired: 7 out]
        n1572 = Not(x="Flip Green Filter") -> (.not. x?=w7013:bool)
        n1573 = local write "Flip Green Filter"(w7013) -> ()
        n1574 = flat-sequence {
          tunnel: w7021 -> [w7026]
          tunnel: w7020 -> [w7025]
          tunnel: [w7023] -> w7018
          tunnel: [w7022] -> w7017
          tunnel: [w7065] -> w7016
          tunnel: w7018 -> [w7065]
          tunnel: [w7064] -> w7015
          tunnel: w7017 -> [w7064]
          tunnel: w7016 -> [w7069]
          tunnel: w7015 -> [w7068]
          tunnel: [w7067] -> w7019
          frame #0 {
            n1575 = xnode "Read/Write Control"("FPGA VI Reference In"=w7026, "error in"=w7025, "Green Filter Flipper"=TRUE) -> ("FPGA VI Reference Out"=w7023:T15, "error out"=w7022:errorcluster)
          }
          frame #1 {
            n1576 = Wait (ms)(milliseconds to wait=u32 100) -> ()  [unwired: 1 out]
          }
          frame #2 {
            n1577 = xnode "Read/Write Control"("FPGA VI Reference In"=w7069, "error in"=w7068, "Green Filter Flipper"=FALSE) -> ("error out"=w7067:errorcluster)  [unwired: 1 out]
          }
        }
      }
      event #44 {
        n1578 = event-data() -> ()  [unwired: 7 out]
        n1579 = local read "Pump 1 contents"() -> (→"Pump 1 cont disp":string)
        n1580 = local read "Pump 3 contents"() -> (→"Pump 3 cont disp":string)
      }
    }
    "error out 2" <- w4183
    n1581 = node-c288() -> ()  [unwired: 2 out]
  }
  n1582 = timed-loop "Oscillate AOD (debugging)" {
    tunnel: w89 -> [w7111]
    tunnel: [w7110] -> w34
    timing: w29 -> [_]
    timing-out: [_] -> w28
    stop <- w7110 stop-if-true
    n1583 = node-c288() -> ()  [unwired: 2 out]
    n1584 = event shown="[0] \"Oscillate Set 1\", \"Fish for Tether\": Value Change" {
      selector: _ -> [_ _ _]
      dyn-events: _ -> [_ _ _]
      timeout: _ -> [_ _ _]
      tunnel: w7111 -> [w7118 _ _]
      tunnel: [FALSE ("Stop All") _ w7371] -> w7110
      event #0 {
        n1585 = event-data() -> ()  [unwired: 6 out]
        n1586 = local read "Oscillate Set 1"() -> (w7117:bool)
        n1587 = Or(x=w7117, y="Fish for Tether") -> (x .or. y?=w7115:bool)
        n1588 = case shown="True" w7115 {
          tunnel: w7118 -> [_ w7120]
          tunnel: "Fish for Tether" -> [_ w7119]
          frame #0 {
          }
          frame #1 {
            n1589 = case shown="True" w7119 {
              frame #0 {
              }
              frame #1 {
                n1590 = local write "Scan axis 2"(TRUE) -> ()
                n1591 = local write "Tether"(FALSE ("Tether")) -> ()
              }
            }
            n1592 = node-c288() -> (w7122:T19)  [unwired: 4 out]
            n1593 = timed-loop "Oscillate AOD" {
              timing: w7122 -> [_]
              timing-out: [_] -> w7121
              tunnel: w7120 -> [w7132]
              tunnel: w7119 -> [w7131]
              i -> [w7134]
              stop <- w7130 stop-if-true
              n1594 = node-c288() -> (w7133:i64)  [unwired: 1 out]
              n1595 = flat-sequence {
                tunnel: w7134 -> [w7161]
                tunnel: w7133 -> [w7160]
                tunnel: w7132 -> [w7139]
                tunnel: w7131 -> [w7142]
                tunnel: [w7142] -> w7129
                tunnel: [w7141] -> w7128
                tunnel: [w7138] -> w7127
                tunnel: [w7135] -> w7125
                tunnel: w7129 -> [w7197]
                tunnel: w7128 -> [w7195]
                tunnel: w7127 -> [w7194]
                tunnel: [w7193] -> w7126
                tunnel: w7125 -> [w7192]
                tunnel: [w7245] -> w7130
                tunnel: w7126 -> [w7244]
                frame #0 {
                  n1596 = Divide(x=w7160, y=i64 1000) -> (x/y=w7155:dbl)
                  n1597 = Multiply(x=w7155, y=w7161) -> (x*y=w7157:dbl)
                  n1598 = local read "BD 1 Frequency 2 (MHz)"() -> (w7140:dbl)
                  n1599 = Multiply(x="Osc. freq. (Hz)", y=6.283185307179586) -> (x*y=w7158:dbl)
                  n1600 = Multiply(x=w7158, y=w7157) -> (x*y=w7137:dbl)
                  n1601 = local read "BD 1 Frequency 1 (MHz)"() -> (w7145:dbl)
                  n1602 = case shown="True" w7142 {
                    tunnel: w7137 -> [w7167 w7172]
                    tunnel: w7145 -> [_ w7183]
                    tunnel: w7140 -> [_ w7184]
                    tunnel: [w7164 w7178] -> w7143
                    tunnel: [FALSE w7175] -> w7138
                    tunnel: [0.0 w7168] -> w7135
                    frame #0 {
                      n1603 = Sine(x=w7167) -> (sin(x)=w7165:dbl)
                      n1604 = Multiply(x=w7165, y="Osc. amp. (MHz)") -> (x*y=w7164:dbl)
                    }
                    frame #1 {
                      n1605 = Cosine(x=w7172) -> (cos(x)=w7187:dbl)
                      n1606 = Subtract(x=w7184, y=w7183) -> (x-y=w7182:dbl)
                      n1607 = Decrement(x=w7187) -> (x-1=w7186:dbl)
                      n1608 = Subtract(x=w7182, y="Closest Delta (MHz)") -> (x-y=w7179:dbl)
                      n1609 = Divide(x=w7186, y=-2.0) -> (x/y=w7180:dbl)
                      n1610 = Multiply(x=w7180, y=w7179) -> (x*y=w7178:dbl)
                      n1611 = local read "Vec Mean of T1 T2"() -> (w7174:dbl[])
                      n1612 = Greater?(x=w7174, y="Stop F (pN)") -> (0:w7176:bool[])
                      n1613 = Or Array Elements(Boolean array=w7176) -> (logical OR=w7175:bool)
                      n1614 = Divide(x=w7172, y=6.283185307179586) -> (x/y=w7171:dbl)
                      n1615 = Round Toward +Infinity(x=w7171) -> (ceil(x): smallest int >= x=w7168:dbl)
                      "Attempts" <- w7168
                      n1616 = Greater?(x=w7168, y="Attempt Limit") -> (0:w7170:bool)
                      n1617 = case shown="True" w7170 {
                        frame #0 {
                        }
                        frame #1 {
                          n1618 = call <vilib>:"Beep.vi"() -> ()  [unwired: 3 in, 9 out]
                          n1619 = local write "Fish for Tether"(FALSE ("Fish for Tether")) -> ()
                          n1620 = local read "Messages"() -> (w7189:string)
                          n1621 = call "Update messages.vi"("Message to add"="Tether fishing timeout." ("Messages"), "Old message string"=w7189) -> ("New message string"=→"Messages":string)
                        }
                      }
                    }
                  }
                  n1622 = local read "BD 2 Frequency 1 (MHz)"() -> (w7144:dbl)
                  n1623 = Select(t=w7145, s="Scan axis 2", f=w7144) -> (s? t:f=w7148:dbl)
                  n1624 = Add(x=w7143, y=w7148) -> (x+y=w7141:dbl)
                  n1625 = Select(t=w7141, s="Scan axis 2", f=w7145) -> (s? t:f=w7151:dbl)
                  n1626 = Select(t=w7144, s="Scan axis 2", f=w7141) -> (s? t:f=w7150:dbl)
                  n1627 = local read "Y RF Frequency Limits (MHz)"() -> (w7146:T12)
                  n1628 = local read "X RF Frequency Limits (MHz)"() -> (w7147:T12)
                  n1629 = local read "BD 1 Frequency 3 (MHz)"() -> (w7154:dbl)
                  n1630 = local read "BD 2 Frequency 2 (MHz)"() -> (w7153:dbl)
                  n1631 = local read "BD 2 Frequency 3 (MHz)"() -> (w7152:dbl)
                  n1632 = call "set RF board frequency - interlace.vi"("Board 2 Frequency Limits"=w7146, "Board 1 Frequency Limits"=w7147, "FPGA VI Reference In"=w7139, "Board 2 Frequency 3 (MHz)"=w7152, "Board 1 Frequency 3 (MHz)"=w7154, "Board 2 Frequency 2 (MHz)"=w7153, "Board 2 Frequency 1 (MHz)"=w7150, "Board 1 Frequency 2 (MHz)"=w7140, "Board 1 Frequency 1  (MHz)"=w7151) -> ()  [unwired: 1 in, 2 out]
                }
                frame #1 {
                  n1633 = And(x=w7197, y=w7194) -> (x .and. y?=w7196:bool)
                  n1634 = case "Only if were fishing and now formed tether" shown="True" w7196 {
                    tunnel: w7195 -> [w7199 w7212]
                    tunnel: [w7198 w7211] -> w7193
                    tunnel: w7192 -> [_ w7207]
                    frame #0 {
                      n1635 = local read "Fish for Tether"() -> (w7198:bool)
                      n1636 = case shown="False" w7198 {
                        tunnel: w7199 -> [w7200 _]
                        frame #0 {
                          n1637 = property on="BD 1 Frequency 1 (MHz)" class="DigNum (strict)"("Val(Sgnl)"=w7200) -> ()  [unwired: 2 in, 2 out]
                        }
                        frame #1 {
                        }
                      }
                    }
                    frame #1 {
                      w7211 = FALSE ("Fish for Tether")
                      n1638 = call <vilib>:"Beep.vi"() -> ()  [unwired: 3 in, 9 out]
                      n1639 = Number To Decimal String(number=w7207, width (-)=i16 1) -> (decimal integer string=w7205:string)
                      n1640 = case shown="\"2\", \"3\", \"4\", \"5\", \"6\"" "Then..." {
                        selector: "Then..." -> [_ w7215]
                        tunnel: w7212 -> [w7214 _]
                        frame #0 {
                          n1641 = property on="BD 1 Frequency 1 (MHz)" class="DigNum (strict)"("Val(Sgnl)"=w7214) -> ()  [unwired: 2 in, 2 out]
                        }
                        frame #1 {
                          n1642 = flat-sequence {
                            tunnel: w7215 -> [w7217]
                            frame #0 {
                              n1643 = property on="Trap Delta (MHz)" class="DigNum (strict)"("Val(Sgnl)"="Move to Delta 1 (MHz)") -> ()  [unwired: 2 in, 2 out]
                            }
                            frame #1 {
                              n1644 = case shown="\"5\", \"6\"" w7217 {
                                selector: w7217 -> [w7220 w7230 _]
                                frame #0 {
                                n1645 = flat-sequence {
                                tunnel: w7220 -> [w7221]
                                tunnel: [w7221] -> w7218
                                tunnel: [w7223] -> w7219
                                tunnel: w7218 -> [w7223]
                                tunnel: w7219 -> [w7227]
                                frame #0 {
                                n1646 = property on="Green Laser ON/Interlacing" class="Bool (strict)"("Val(Sgnl)"=TRUE ("Value (Signaling)")) -> ()  [unwired: 2 in, 2 out]
                                }
                                frame #1 {
                                n1647 = Multiply(x="Wait Before Save (s)", y=u32 1000 ("x")) -> (x*y=w7225:u32)
                                n1648 = Wait (ms)(milliseconds to wait=w7225) -> ()  [unwired: 1 out]
                                }
                                frame #2 {
                                n1649 = property on="Start Saving" class="Bool (strict)"("Value"=TRUE ("Start Saving")) -> ()  [unwired: 2 in, 2 out]
                                n1650 = case shown="\"4\"" w7227 {
                                frame #0 {
                                }
                                frame #1 {
                                n1651 = property on="Fl. Triggered..." class="Bool (strict)"("Val(Sgnl)"=TRUE ("Value (Signaling)")) -> ()  [unwired: 2 in, 2 out]
                                }
                                }
                                }
                                }
                                }
                                frame #1 {
                                n1652 = flat-sequence {
                                tunnel: w7230 -> [w7238]
                                frame #0 {
                                n1653 = Wait (ms)(milliseconds to wait=u32 500) -> ()  [unwired: 1 out]
                                }
                                frame #1 {
                                n1654 = property on="Trap Raster Scan" class="Bool (strict)"("Val(Sgnl)"=TRUE ("Value (Signaling)")) -> ()  [unwired: 2 in, 2 out]
                                }
                                frame #2 {
                                n1655 = Wait (ms)(milliseconds to wait=u32 500) -> ()  [unwired: 1 out]
                                }
                                frame #3 {
                                n1656 = while {
                                stop <- w7234 stop-if-true
                                n1657 = local read "Saving..."() -> (w7235:bool)
                                n1658 = Wait (ms)(milliseconds to wait=u32 100) -> ()  [unwired: 1 out]
                                n1659 = Not(x=w7235) -> (.not. x?=w7234:bool)
                                }
                                }
                                frame #4 {
                                n1660 = property on="Trap Delta (MHz)" class="DigNum (strict)"("Val(Sgnl)"="Move to Delta 2 (MHz)") -> ()  [unwired: 2 in, 2 out]
                                }
                                frame #5 {
                                n1661 = case shown="\"6\"" w7238 {
                                frame #0 {
                                }
                                frame #1 {
                                n1662 = local read "Tether"() -> (w7239:bool)
                                n1663 = case shown="True" w7239 {
                                frame #0 {
                                }
                                frame #1 {
                                n1664 = flat-sequence {
                                frame #0 {
                                n1665 = Wait (ms)(milliseconds to wait=u32 500) -> ()  [unwired: 1 out]
                                }
                                frame #1 {
                                n1666 = property on="Green Laser ON/Interlacing" class="Bool (strict)"("Val(Sgnl)"=TRUE ("Green Laser ON/Interlacing")) -> ()  [unwired: 2 in, 2 out]
                                }
                                frame #2 {
                                n1667 = Wait (ms)(milliseconds to wait=u32 500) -> ()  [unwired: 1 out]
                                }
                                frame #3 {
                                n1668 = local write "Start Saving"(TRUE ("Start Saving")) -> ()
                                }
                                }
                                }
                                }
                                }
                                }
                                }
                                }
                                }
                                frame #2 {
                                }
                              }
                            }
                          }
                        }
                      }
                      n1669 = Concatenate Strings("Formed tether in ", w7205, " attempt(s)." ("string")) -> (w7202:string)
                      n1670 = local read "Messages"() -> (w7209:string)
                      n1671 = local write "Fish for Tether"(w7211) -> ()
                      n1672 = call "Update messages.vi"("Message to add"=w7202, "Old message string"=w7209) -> ("New message string"=w7208:string)
                      n1673 = local write "Messages"(w7208) -> ()
                      n1674 = Get Date/Time In Seconds() -> (seconds since 1Jan1904=→"Time tether formed":timestamp)
                      "Tether" <- "Tether Alarm?"
                    }
                  }
                }
                frame #2 {
                  n1675 = local read "Oscillate Set 1"() -> (w7249:bool)
                  n1676 = Or(x=w7249, y=w7244) -> (x .or. y?=w7246:bool)
                  n1677 = local read "Stop All"() -> (w7247:bool)
                  n1678 = Not(x=w7246) -> (.not. x?=w7248:bool)
                  n1679 = Compound Arithmetic op=OR(w7247, w7248) -> (w7245:bool)
                }
              }
              n1680 = node-c288() -> ()  [unwired: 2 out]
            }
            n1681 = node-c288(w7121) -> ()  [unwired: 1 out]
          }
        }
      }
      event #1 {
        n1682 = event-data() -> ()  [unwired: 7 out]
        n1683 = case shown="True" "Fl. Triggered..." {
          frame #0 {
          }
          frame #1 {
            n1684 = node-c288() -> (w7259:T19)  [unwired: 4 out]
            n1685 = timed-loop {
              timing: w7259 -> [_]
              timing-out: [_] -> w7258
              tunnel: "Action" -> [w7263]
              shift-right: [w7260] -> _
              shift-left: u8 255 -> [w7262]
              stop <- w7264 stop-if-true
              n1686 = node-c288() -> ()  [unwired: 2 out]
              n1687 = flat-sequence {
                tunnel: w7263 -> [w7276]
                tunnel: w7262 -> [w7273]
                tunnel: [w7272] -> w7261
                tunnel: [w7362] -> w7264
                tunnel: w7261 -> [w7361]
                tunnel: [w7361] -> w7260
                frame #0 {
                  n1688 = local read "Delta Fl. 2"() -> (w7267:dbl)
                  n1689 = local read "Delta Fl. 1"() -> (w7268:dbl)
                  n1690 = Select(t=w7268, s="APD to Watch", f=w7267) -> (s? t:f=w7266:dbl)
                  n1691 = Multiply(x="Fl. Delta Thresh. (kHz)", y=1000.0) -> (x*y=w7275:dbl)
                  n1692 = Greater?(x=w7266, y=w7275) -> (0:w7270:bool)
                  n1693 = Or(x="Force Yank", y=w7270) -> (x .or. y?=w7271:bool)
                  n1694 = case shown="True" w7271 {
                    tunnel: w7276 -> [_ w7286]
                    tunnel: w7273 -> [w7278 w7282]
                    tunnel: [w7278 w7279] -> w7272
                    frame #0 {
                    }
                    frame #1 {
                      n1695 = flat-sequence {
                        tunnel: w7283 -> [w7292]
                        tunnel: [w7292] -> w7287
                        tunnel: w7286 -> [w7291]
                        tunnel: [w7291] -> w7285
                        tunnel: [w7290] -> w7284
                        tunnel: w7282 -> [w7289]
                        tunnel: [w7288] -> w7281
                        tunnel: w7287 -> [w7317]
                        tunnel: w7285 -> [w7316]
                        tunnel: w7284 -> [w7315]
                        tunnel: w7281 -> [w7314]
                        tunnel: [w7314] -> w7280
                        tunnel: w7280 -> [w7359]
                        tunnel: [w7359] -> w7279
                        frame #0 {
                          n1696 = call <vilib>:"Beep.vi"() -> ()  [unwired: 3 in, 9 out]
                          n1697 = local write "Waiting"(FALSE ("Waiting")) -> ()
                          n1698 = Increment(x=w7289) -> (x+1=w7288:u8)
                          n1699 = case shown="\"Yank\"" w7291 {
                            tunnel: w7288 -> [_ _ w7298]
                            frame #0 {
                              n1700 = property on="Confocal Image" class="Bool (strict)"("Val(Sgnl)"=TRUE ("Value (Signaling)")) -> ()  [unwired: 2 in, 2 out]
                            }
                            frame #1 {
                            }
                            frame #2 {
                              n1701 = flat-sequence {
                                tunnel: w7298 -> [w7301]
                                tunnel: [w7300] -> w7297
                                tunnel: ["N Array El"] -> w7296
                                tunnel: w7297 -> [w7311]
                                tunnel: w7296 -> [w7307]
                                frame #0 {
                                n1702 = Multiply(x="Yank Delay (s)", y=1000.0) -> (x*y=w7304:dbl)
                                n1703 = Quotient & Remainder(x=w7301, y="N Array El") -> (x-y*floor(x/y)=w7300:u8)  [unwired: 1 out]
                                n1704 = Wait (ms)(milliseconds to wait=w7304) -> ()  [unwired: 1 out]
                                }
                                frame #1 {
                                n1705 = Random Number (0-1)() -> (number: 0 to 1=w7308:dbl)
                                n1706 = Multiply(x=w7307, y=w7308) -> (x*y=w7306:dbl)
                                n1707 = Round Toward -Infinity(1:w7306) -> (0:w7305:dbl)
                                n1708 = Select(t=w7305, s="Random Choice", f=w7311) -> (s? t:f=w7309:dbl)
                                n1709 = Index Array(array="Yank to Delta Array (MHz)", index=w7309) -> (element=w7312:dbl)
                                n1710 = property on="Trap Delta (MHz)" class="DigNum (strict)"("Val(Sgnl)"=w7312) -> ()  [unwired: 2 in, 2 out]
                                }
                              }
                            }
                          }
                          n1711 = local read "Time (s)"() -> (w7290:dbl)
                          "Fl. High" <- TRUE ("Yanking")
                        }
                        frame #1 {
                          n1712 = node-c288() -> (w7319:T19)  [unwired: 4 out]
                          n1713 = timed-loop {
                            timing: w7319 -> [_]
                            timing-out: [_] -> w7318
                            tunnel: w7317 -> [w7335]
                            tunnel: w7316 -> [w7333]
                            tunnel: w7315 -> [w7332]
                            stop <- w7334 stop-if-true
                            n1714 = node-c288() -> ()  [unwired: 2 out]
                            n1715 = local read "Fl. Delta Thresh. (kHz)"() -> (w7327:dbl)
                            n1716 = local read "Fl. Triggered..."() -> (w7336:bool)
                            n1717 = local read "Delta Fl. 1"() -> (w7323:dbl)
                            n1718 = local read "Delta Fl. 2"() -> (w7321:dbl)
                            n1719 = local read "Stop All"() -> (w7330:bool)
                            n1720 = local read "APD to Watch"() -> (w7322:bool)
                            n1721 = Select(t=w7323, s=w7322, f=w7321) -> (s? t:f=w7320:dbl)
                            n1722 = Not(x=w7336) -> (.not. x?=w7331:bool)
                            n1723 = Multiply(x=w7327, y=1000.0) -> (x*y=w7326:dbl)
                            n1724 = Negate(x=w7326) -> (-x=w7325:dbl)
                            n1725 = Less?(x=w7320, y=w7325) -> (x < y?=w7329:bool)
                            n1726 = Compound Arithmetic op=OR(w7329, w7330, w7331, "Force Reset") -> (w7334:bool)
                            n1727 = case shown="True" w7334 {
                              tunnel: w7335 -> [_ w7347]
                              tunnel: w7333 -> [_ w7346]
                              tunnel: w7332 -> [_ w7344]
                              frame #0 {
                              }
                              frame #1 {
                                n1728 = case shown="\"Yank\"" w7346 {
                                tunnel: w7347 -> [_ w7348]
                                frame #0 {
                                }
                                frame #1 {
                                n1729 = flat-sequence {
                                tunnel: [w7353] -> w7349
                                tunnel: w7348 -> [w7353]
                                tunnel: w7349 -> [w7354]
                                frame #0 {
                                n1730 = local read "Yank Delay (s)"() -> (w7352:dbl)
                                n1731 = Multiply(x=w7352, y=1000.0) -> (x*y=w7350:dbl)
                                n1732 = Wait (ms)(milliseconds to wait=w7350) -> ()  [unwired: 1 out]
                                }
                                frame #1 {
                                n1733 = property on="Trap Delta (MHz)" class="DigNum (strict)"("Val(Sgnl)"=w7354) -> ()  [unwired: 2 in, 2 out]
                                }
                                }
                                }
                                }
                                n1734 = local read "Time (s)"() -> (w7345:dbl)
                                n1735 = Subtract(x=w7345, y=w7344) -> (x-y=w7341:dbl)
                                "Duration (s)" <- w7341
                                n1736 = Number To Decimal String(number=w7341, width (-)=i16 0) -> (decimal integer string=w7339:string)
                                n1737 = Concatenate Strings(w7339, " s fluorescence event." ("string")) -> (w7337:string)
                                n1738 = local read "Messages"() -> (w7343:string)
                                n1739 = call "Update messages.vi"("Message to add"=w7337, "Old message string"=w7343) -> ("New message string"=w7342:string)
                                n1740 = call <vilib>:"Beep.vi"() -> ()  [unwired: 3 in, 9 out]
                                n1741 = local write "Messages"(w7342) -> ()
                              }
                            }
                            n1742 = node-c288() -> ()  [unwired: 2 out]
                          }
                          n1743 = node-c288(w7318) -> ()  [unwired: 1 out]
                        }
                        frame #2 {
                          n1744 = local write "Fl. High"(FALSE ("Yanking")) -> ()
                        }
                      }
                      n1745 = local read "Trap Delta (MHz)"() -> (w7283:dbl)
                    }
                  }
                }
                frame #1 {
                  n1746 = local read "Stop All"() -> (w7365:bool)
                  n1747 = local read "Fl. Triggered..."() -> (w7363:bool)
                  n1748 = Not(x=w7363) -> (.not. x?=w7364:bool)
                  n1749 = Or(x=w7364, y=w7365) -> (x .or. y?=w7362:bool)
                  n1750 = Not(x=w7362) -> (.not. x?=→"Waiting":bool)
                }
              }
              n1751 = node-c288() -> ()  [unwired: 2 out]
            }
            n1752 = node-c288(w7258) -> ()  [unwired: 1 out]
          }
        }
      }
      event #2 {
        n1753 = event-data() -> ()  [unwired: 7 out]
        n1754 = local read "Stop All"() -> (w7371:bool)
      }
    }
    n1755 = node-c288() -> ()  [unwired: 2 out]
  }
  n1756 = timed-loop "Mouse control: trap position (AOM deflection), set confocal spot from image" {
    tunnel: [w7373] -> w146
    tunnel: w89 -> [w7372]
    timing: w33 -> [_]
    timing-out: [_] -> w32
    stop <- w7373 stop-if-true
    n1757 = node-c288() -> ()  [unwired: 2 out]
    n1758 = event shown="[0] \"Pane\": Mouse Down" {
      selector: _ -> [_ _]
      dyn-events: _ -> [_ _]
      timeout: _ -> [_ _]
      tunnel: w7372 -> [w7376 _]
      event #0 {
        n1759 = event-data() -> ("Time"=w7378:u32, "Coords"=w7377:T7, "Button"=w7379:u16)  [unwired: 6 out]
        n1760 = case shown="1" w7379 {
          tunnel: w7378 -> [_ _ w7482]
          tunnel: w7377 -> [_ w7416 w7480]
          tunnel: w7376 -> [_ _ w7478]
          frame #0 {
          }
          frame #1 {
            n1761 = property on="APD 2" class="ImageControl"() -> ("Displayed Image Position"=w7386:cluster{"Left":i32, "Top":i32})  [unwired: 2 in, 2 out]
            n1762 = property on="APD 1" class="ImageControl"() -> ("Displayed Image Position"=w7415:cluster{"Left":i32, "Top":i32})  [unwired: 2 in, 2 out]
            n1763 = property on="Detection Laser X" class="ImageControl"() -> ("Displayed Image Position"=w7412:cluster{"Left":i32, "Top":i32})  [unwired: 2 in, 2 out]
            n1764 = property on="Detection Laser Y" class="ImageControl"() -> ("Displayed Image Position"=w7411:cluster{"Left":i32, "Top":i32})  [unwired: 2 in, 2 out]
            n1765 = property on="APD 2" class="ImageControl"() -> ("Displayed Image Size"=w7385:cluster{"Width":u32, "Height":u32})  [unwired: 2 in, 2 out]
            n1766 = property on="APD 1" class="ImageControl"() -> ("Displayed Image Size"=w7413:cluster{"Width":u32, "Height":u32})  [unwired: 2 in, 2 out]
            n1767 = property on="Detection Laser X" class="ImageControl"() -> ("Displayed Image Size"=w7414:cluster{"Width":u32, "Height":u32})  [unwired: 2 in, 2 out]
            n1768 = property on="Detection Laser Y" class="ImageControl"() -> ("Displayed Image Size"=w7410:cluster{"Width":u32, "Height":u32})  [unwired: 2 in, 2 out]
            n1769 = Unbundle By Name(w7385) -> ("Width"=w7382:u32, "Height"=w7381:u32)
            n1770 = Unbundle By Name(w7386) -> ("Left"=w7384:i32, "Top"=w7383:i32)
            n1771 = Unbundle By Name(w7413) -> ("Width"=w7407:u32, "Height"=w7406:u32)
            n1772 = Unbundle By Name(w7414) -> ("Width"=w7403:u32, "Height"=w7402:u32)
            n1773 = Unbundle By Name(w7410) -> ("Width"=w7399:u32, "Height"=w7398:u32)
            n1774 = Unbundle By Name(w7415) -> ("Left"=w7409:i32, "Top"=w7408:i32)
            n1775 = Unbundle By Name(w7412) -> ("Left"=w7405:i32, "Top"=w7404:i32)
            n1776 = Unbundle By Name(w7411) -> ("Left"=w7401:i32, "Top"=w7400:i32)
            n1777 = Bundle("Left"=w7384, "Top"=w7383, "Width"=w7382, "Height"=w7381) -> (w7380:T43)  [unwired: 1 in]
            n1778 = Bundle("Left"=w7409, "Top"=w7408, "Width"=w7407, "Height"=w7406) -> (w7397:T43)  [unwired: 1 in]
            n1779 = Bundle("Left"=w7405, "Top"=w7404, "Width"=w7403, "Height"=w7402) -> (w7396:T43)  [unwired: 1 in]
            n1780 = Bundle("Left"=w7401, "Top"=w7400, "Width"=w7399, "Height"=w7398) -> (w7395:T43)  [unwired: 1 in]
            n1781 = Build Cluster Array(w7380, w7397, w7396, w7395) -> (w7394:T44)
            n1782 = for {
              tunnel: w7416 -> [w7427]
              tunnel: w7394 -> [w7428] mode=indexing
              shift-right: [w7425] -> w7392
              shift-left: TRUE -> [w7426]
              shift-right: [w7424] -> w7390
              shift-left: _ -> [w7420]
              shift-right: [w7423] -> w7389
              shift-left: _ -> [w7419]
              shift-right: [w7422] -> w7388
              shift-left: _ -> [w7418]
              shift-right: [w7421] -> w7387
              shift-left: _ -> [w7417]
              n1783 = case shown="True" w7426 {
                selector: w7426 -> [w7433 _]
                tunnel: w7428 -> [_ w7442]
                tunnel: w7427 -> [_ w7440]
                tunnel: [w7433 w7438] -> w7425
                tunnel: [w7432 w7437] -> w7424
                tunnel: [w7431 w7436] -> w7423
                tunnel: [w7430 w7435] -> w7422
                tunnel: [w7429 w7434] -> w7421
                tunnel: w7420 -> [w7432 _]
                tunnel: w7419 -> [w7431 _]
                tunnel: w7418 -> [w7430 _]
                tunnel: w7417 -> [w7429 _]
                frame #0 {
                }
                frame #1 {
                  n1784 = Unbundle(w7442) -> (w7441:T43)
                  n1785 = call "isclickinwindow.vi"("Image Param"=w7441, "Point32"=w7440) -> ("4 Y"=w7434:i32, "3 Height"=w7435:i32, "2 X"=w7436:i32, "1 Width"=w7437:i32, "In image?"=w7439:bool)  [unwired: 1 in]
                  n1786 = Not(x=w7439) -> (.not. x?=w7438:bool)
                }
              }
            }
            n1787 = Not(x=w7392) -> (.not. x?=w7391:bool)
            n1788 = case shown="True" w7391 {
              tunnel: w7389 -> [_ w7455]
              tunnel: w7387 -> [_ w7454]
              tunnel: w7390 -> [_ w7453]
              tunnel: w7388 -> [_ w7452]
              frame #0 {
              }
              frame #1 {
                w7448 = FALSE ("Get Point")
                n1789 = local read "Scan lines (y)"() -> (w7457:u64)
                n1790 = local read "Actual MCL Inc (V)"() -> (w7449:dbl)
                n1791 = local read "Scan steps (MCL)"() -> (w7456:u64)
                n1792 = Divide "Y Pix/step"(x=w7452, y=w7457) -> (x/y=w7464:dbl)
                n1793 = Divide "Y V/pix"(x=w7449, y=w7464) -> (x/y=w7463:dbl)
                n1794 = Divide "Y half step offset"(x=w7449, y=2.0) -> (x/y=w7465:dbl)
                n1795 = Divide "X pix/step"(x=w7453, y=w7456) -> (x/y=w7462:dbl)
                n1796 = Negate(x=w7465) -> (-x=w7466:dbl)
                n1797 = local read "Initial Y"() -> (w7472:dbl)
                n1798 = Multiply(x=w7454, y=w7463) -> (x*y=w7473:dbl)
                n1799 = Divide "X half step offset"(x=w7449, y=2.0) -> (x/y=w7459:dbl)
                n1800 = Divide "X V/pix"(x=w7449, y=w7462) -> (x/y=w7461:dbl)
                n1801 = Multiply(x=w7449, y=w7456) -> (x*y=w7468:dbl)
                n1802 = Compound Arithmetic op=ADD(w7466, w7473, w7472) -> (w7450:dbl)
                "Pointer Y (V)" <- w7450
                n1803 = Multiply(x=w7461, y=w7455) -> (x*y=w7470:dbl)
                n1804 = Negate(x=w7459) -> (-x=w7458:dbl)
                n1805 = local read "Initial X"() -> (w7471:dbl)
                n1806 = Negate(x=w7470) -> (-x=w7469:dbl)
                n1807 = Compound Arithmetic op=ADD(w7458, w7468, w7471, w7469) -> (w7451:dbl)
                "Pointer X (V)" <- w7451
                n1808 = Or(x="Set X Only", y="Set Confocal Spot (X-Y)") -> (x .or. y?=w7444:bool)
                n1809 = Or(x="Set Confocal Spot (X-Y)", y="Set Y Only") -> (x .or. y?=w7443:bool)
                n1810 = case shown="True" w7444 {
                  tunnel: w7451 -> [_ w7474]
                  frame #0 {
                  }
                  frame #1 {
                    n1811 = property on="AO2" class="Slide (strict)"("Val(Sgnl)"=w7474) -> ()  [unwired: 2 in, 2 out]
                  }
                }
                n1812 = case shown="True" w7443 {
                  tunnel: w7450 -> [_ w7475]
                  frame #0 {
                  }
                  frame #1 {
                    n1813 = property on="AO1" class="Slide (strict)"("Val(Sgnl)"=w7475) -> ()  [unwired: 2 in, 2 out]
                  }
                }
                n1814 = local write "Set Confocal Spot (X-Y)"(w7448) -> ()
                n1815 = local write "Set X Only"(w7448) -> ()
                n1816 = local write "Set Y Only"(w7448) -> ()
              }
            }
          }
          frame #2 {
            n1817 = local read "BD 2 Frequency 1 (MHz)"() -> (w7476:dbl)
            n1818 = local read "BD 1 Frequency 1 (MHz)"() -> (w7477:dbl)
            n1819 = local write "Manipulating Trap"(TRUE ("Manipulating Trap")) -> ()
            n1820 = local write "Coords"(T7 {"Horizontal"=0, "Vertical"=0} ("Coords")) -> ()
            n1821 = while {
              tunnel: w7482 -> [w7487]
              tunnel: w7480 -> [w7486]
              tunnel: w7478 -> [w7485]
              tunnel: w7477 -> [w7484]
              tunnel: w7476 -> [w7483]
              stop <- w7488 stop-if-true
              n1822 = event shown="[0] \"Pane\": Mouse Move" {
                selector: _ -> [_ _]
                dyn-events: _ -> [_ _]
                timeout: _ -> [_ _]
                tunnel: ["Force Manip Abort" w7552] -> w7488
                tunnel: w7487 -> [w7495 _]
                tunnel: w7486 -> [w7493 _]
                tunnel: w7485 -> [w7492 _]
                tunnel: w7484 -> [w7491 _]
                tunnel: w7483 -> [w7490 _]
                event #0 {
                  n1823 = event-data() -> ("Time"=w7496:u32, "Coords"=w7497:T7)  [unwired: 3 out]
                  n1824 = Less?(x=w7496, y=w7495) -> (x < y?=w7494:bool)
                  n1825 = case "Makes sure old motion events prior to mouse click aren't used" shown="False" w7494 {
                    tunnel: w7497 -> [w7539 _]
                    tunnel: w7493 -> [w7540 _]
                    tunnel: w7492 -> [w7517 _]
                    tunnel: w7491 -> [w7513 _]
                    tunnel: w7490 -> [w7512 _]
                    frame #0 {
                      n1826 = Subtract(x=w7539, y=w7540) -> (x-y=w7538:T7)
                      "Coords" <- w7538
                      n1827 = local read "Y RF Frequency Limits (MHz)"() -> (w7498:T12)
                      n1828 = To Double Precision Float(number=w7538) -> (double precision float=w7537:cluster{"Horizontal":dbl, "Vertical":dbl})
                      n1829 = Multiply(x=cluster{"Horizontal":dbl, "Vertical":dbl} {"Horizontal"=-1.0, "Vertical"=1.0}, y="Manipulation Scaling") -> (x*y=w7533:cluster{"Horizontal":dbl, "Vertical":dbl})
                      n1830 = local read "X RF Frequency Limits (MHz)"() -> (w7499:T12)
                      n1831 = Multiply(x=w7537, y=w7533) -> (x*y=w7535:cluster{"Horizontal":dbl, "Vertical":dbl})
                      n1832 = Unbundle By Name(w7535) -> ("Horizontal"=w7530:dbl, "Vertical"=w7534:dbl)
                      n1833 = Unbundle By Name(w7498) -> ("Maximum"=w7501:dbl, "Minimum"=w7500:dbl)
                      n1834 = Boolean To (0,1)(Boolean="Manip. X?") -> (0, 1=w7528:i16)
                      n1835 = Boolean To (0,1)(Boolean="Manip. Y?") -> (0, 1=w7525:i16)
                      n1836 = Multiply(x=w7534, y=w7525) -> (x*y=w7527:dbl)
                      n1837 = Multiply(x=w7528, y=w7530) -> (x*y=w7531:dbl)
                      n1838 = local read "BD 1 Frequency 2 (MHz)"() -> (w7515:dbl)
                      n1839 = Unbundle By Name(w7499) -> ("Maximum"=w7503:dbl, "Minimum"=w7502:dbl)
                      n1840 = local read "BD 2 Frequency 2 (MHz)"() -> (w7514:dbl)
                      n1841 = Add(x=w7512, y=w7527) -> (x+y=w7505:dbl)
                      n1842 = Add(x=w7513, y=w7531) -> (x+y=w7507:dbl)
                      n1843 = In Range and Coerce(upper limit=w7503, x=w7507, lower limit=w7502) -> (coerced(x)=w7506:dbl)  [unwired: 1 out]
                      n1844 = In Range and Coerce(upper limit=w7501, x=w7505, lower limit=w7500) -> (coerced(x)=w7504:dbl)  [unwired: 1 out]
                      n1845 = Subtract(x=w7506, y=w7515) -> (x-y=w7524:dbl)
                      n1846 = Subtract(x=w7504, y=w7514) -> (x-y=w7523:dbl)
                      n1847 = Square(x=w7524) -> (x^2=w7522:dbl)
                      n1848 = Square(x=w7523) -> (x^2=w7521:dbl)
                      n1849 = Add(x=w7522, y=w7521) -> (x+y=w7520:dbl)
                      n1850 = Square Root(x=w7520) -> (sqrt(x)=w7516:dbl)
                      n1851 = In Range and Coerce(upper limit="Limit Max (MHz)", x=w7516, lower limit="Limit Min (MHz)") -> (In Range?=w7509:bool)  [unwired: 1 out]
                      n1852 = Not(x="Limits Enable") -> (.not. x?=w7508:bool)
                      n1853 = Or(x=w7509, y=w7508) -> (x .or. y?=w7510:bool)
                      n1854 = case shown="True" w7510 {
                        tunnel: w7517 -> [_ w7550]
                        tunnel: w7516 -> [_ w7541]
                        tunnel: w7506 -> [_ w7548]
                        tunnel: w7515 -> [_ w7547]
                        tunnel: w7504 -> [_ w7546]
                        tunnel: w7514 -> [_ w7545]
                        tunnel: w7499 -> [_ w7543]
                        tunnel: w7498 -> [_ w7542]
                        frame #0 {
                        }
                        frame #1 {
                          n1855 = local read "BD 1 Frequency 3 (MHz)"() -> (w7549:dbl)
                          n1856 = local read "BD 2 Frequency 3 (MHz)"() -> (w7544:dbl)
                          n1857 = local write "Trap Delta (MHz)"(w7541) -> ()
                          n1858 = property on="Initial delta (MHz)" class="DigNum (strict)"("Val(Sgnl)"=w7541) -> ()  [unwired: 2 in, 2 out]
                          n1859 = call "set RF board frequency - interlace.vi"("Board 2 Frequency Limits"=w7542, "Board 1 Frequency Limits"=w7543, "FPGA VI Reference In"=w7550, "Board 2 Frequency 3 (MHz)"=w7544, "Board 1 Frequency 3 (MHz)"=w7549, "Board 2 Frequency 2 (MHz)"=w7545, "Board 2 Frequency 1 (MHz)"=w7546, "Board 1 Frequency 2 (MHz)"=w7547, "Board 1 Frequency 1  (MHz)"=w7548) -> ()  [unwired: 1 in, 2 out]
                          n1860 = local write "BD 2 Frequency 1 (MHz)"(w7546) -> ()
                          n1861 = local write "BD 1 Frequency 1 (MHz)"(w7548) -> ()
                        }
                      }
                    }
                    frame #1 {
                    }
                  }
                }
                event #1 {
                  n1862 = event-data() -> ("Button"=w7551:u16)  [unwired: 8 out]
                  n1863 = case shown="3" w7551 {
                    tunnel: [FALSE TRUE] -> w7552
                    frame #0 {
                    }
                    frame #1 {
                      n1864 = local write "Manipulating Trap"(FALSE ("Manipulating Trap")) -> ()
                    }
                  }
                }
              }
            }
          }
        }
      }
      event #1 {
        n1865 = event-data() -> ()  [unwired: 6 out]
      }
    }
    n1866 = local read "Stop All"() -> (w7373:bool)
    n1867 = node-c288() -> ()  [unwired: 2 out]
  }
  n1868 = timed-loop "Run Scripts, including: stage motion" {
    tunnel: w23 -> [w7558]
    tunnel: w22 -> [w7559]
    tunnel: [w7559] -> w21
    tunnel: [w7558] -> w20
    timing: w18 -> [_]
    timing-out: [_] -> w17
    tunnel: w1 -> [w7557]
    tunnel: w2 -> [w7556]
    stop <- w7560 stop-if-true
    n1869 = node-c288() -> ()  [unwired: 1 in, 1 out]
    n1870 = event shown="[10] \"Got ADig bead\": Value Change" {
      selector: _ -> [_ _ _ _ _ _ _ _ _ _ _ _ _ _]
      dyn-events: _ -> [_ _ _ _ _ _ _ _ _ _ _ _ _ _]
      timeout: _ -> [_ _ _ _ _ _ _ _ _ _ _ _ _ _]
      tunnel: ["Set Position" "Move to Position" "Move Cap. 1 (DNA Right)" "Move Cap. 2 (ADig Left)" _ "Cal/Data Acq. Spot" "Dump Beads" "Dip for Protein" _ _ "Got ADig bead" "Got DNA bead" "Take Detection Laser\nImage" _] -> _
      tunnel: [_ _ _ _ _ _ _ _ _ _ _ _ _ w7978] -> w7560
      tunnel: w7558 -> [w7578 w7586 w7610 w7665 w7710 w7746 w7787 w7812 w7862 w7888 _ _ _ _]
      tunnel: w7559 -> [w7579 w7587 w7611 w7666 w7711 w7747 w7788 w7813 w7863 w7889 _ _ _ _]
      tunnel: w7557 -> [_ _ w7608 w7662 _ _ _ _ _ _ _ _ _ _]
      tunnel: w7556 -> [_ _ w7607 w7663 _ _ _ _ _ _ _ _ _ _]
      event #0 {
        n1871 = event-data() -> ()  [unwired: 1 in, 5 out]
        n1872 = Build Array("Set Position 1", "Set Position 2", "Set Position 3", "Set Position 4", "Set Position 5") -> (w7577:bool[])
        n1873 = Boolean Array To Number(Boolean array=w7577) -> (number=w7576:u32)
        n1874 = Logarithm Base 2(1:w7576) -> (0:w7568:dbl)
        n1875 = call "Read Stage Position.vi"("error in"=w7578, "VISA resource name in"=w7579) -> ("Current Position"=w7583:cluster{dbl, dbl, dbl}, "error out"=w7582:errorcluster)  [unwired: 2 out]
        n1876 = Decrement(x="Position") -> (x-1=w7566:dbl)
        n1877 = Greater Or Equal?(x=w7568, y=0.0) -> (x >= y?=w7569:bool)
        n1878 = local write "Stage Control Serial Error"(w7582) -> ()
        n1879 = Cluster To Array(cluster=w7583) -> (array=w7580:dbl[])
        n1880 = Select(t=w7568, s=w7569, f=w7566) -> (s? t:f=w7565:dbl)
        n1881 = Increment(x=w7565) -> (x+1=w7564:dbl)
        n1882 = Build Array (concatenate)(w7564, w7580) -> (w7563:dbl[])
        n1883 = Replace Array Subset(array="Saved Stage Positions", new element=w7563, index (row)=w7565) -> (w7581:dbl[][])  [unwired: 1 in]
        n1884 = local write "Saved Stage Positions"(w7581) -> ()
      }
      event #1 {
        n1885 = event-data() -> ()  [unwired: 1 in, 5 out]
        n1886 = flat-sequence {
          tunnel: w7587 -> [w7590]
          tunnel: w7586 -> [w7589]
          frame #0 {
            n1887 = local read "Position"() -> (w7602:dbl)
            n1888 = local read "Saved Stage Positions"() -> (w7600:dbl[][])
            n1889 = Decrement(x=w7602) -> (x-1=w7599:dbl)
            n1890 = Array Subset(array=w7600, index (row)=w7599, length (row)=1 ("length"), index (col)=1 ("index"), length (col)=3 ("length")) -> (w7596:dbl[][])
            n1891 = Reshape Array(w7596, 3 ("dimension size")) -> (w7594:dbl[])
            n1892 = Array To Cluster(array=w7594) -> (cluster=w7593:cluster{"[0]":dbl, "[1]":dbl, "[2]":dbl})
            n1893 = call "Set Stage Position.vi"("Position"=w7593, "error in"=w7589, "VISA resource name in"=w7590) -> ("error out"=w7592:errorcluster)  [unwired: 2 out]
            n1894 = local write "Stage Control Serial Error"(w7592) -> ()
            n1895 = local write "Stage Moving"(TRUE ("Stage Moving")) -> ()
          }
          frame #1 {
            n1896 = call <vilib>:"Beep.vi"() -> ()  [unwired: 3 in, 9 out]
            n1897 = local write "Stage Moving"(FALSE ("Stage Moving")) -> ()
          }
        }
      }
      event #2 {
        n1898 = event-data() -> ()  [unwired: 1 in, 5 out]
        n1899 = local write "Move Cap. 1 (DNA Right)"(FALSE ("Move Cap. 1 (DNA Right)")) -> ()
        n1900 = flat-sequence {
          tunnel: w7611 -> [w7619]
          tunnel: w7610 -> [w7618]
          tunnel: w7608 -> [w7617]
          tunnel: w7607 -> [w7616]
          tunnel: [w7615] -> w7606
          tunnel: [w7614] -> w7605
          tunnel: ["Cap 1 Samp Flow ON"] -> w7604
          tunnel: w7606 -> [w7642]
          tunnel: w7605 -> [w7641]
          tunnel: w7604 -> [w7640]
          frame #0 {
            n1901 = local read "Saved Stage Positions"() -> (w7629:dbl[][])
            n1902 = Array Subset(array=w7629, index (row)=0 ("index"), length (row)=1 ("length"), index (col)=1 ("index"), length (col)=3 ("length")) -> (w7626:dbl[][])
            n1903 = Reshape Array(w7626, 3 ("dimension size")) -> (w7624:dbl[])
            n1904 = Array To Cluster(array=w7624) -> (cluster=w7623:cluster{"[0]":dbl, "[1]":dbl, "[2]":dbl})
            n1905 = case shown="True" "Cap 1 Samp Flow ON" {
              tunnel: w7616 -> [w7631 w7637]
              tunnel: w7617 -> [w7632 w7636]
              tunnel: [w7632 w7634] -> w7615
              tunnel: [w7631 w7633] -> w7614
              frame #0 {
              }
              frame #1 {
                # "run flow"
                n1906 = Concatenate Strings("run" ("string"), "\r") -> (w7638:string)
                n1907 = VISA Write(VISA resource name=w7636, write buffer=w7638, error in (no error)=w7637) -> (VISA resource name out=w7634:refnum<visa-resource-name>, error out=w7633:errorcluster)  [unwired: 1 out]
              }
            }
            n1908 = call "Set Stage Position.vi"("Position"=w7623, "error in"=w7618, "VISA resource name in"=w7619) -> ("error out"=w7622:errorcluster)  [unwired: 2 out]
            n1909 = local write "Stage Control Serial Error"(w7622) -> ()
            n1910 = local write "Stage Moving"(TRUE ("Stage Moving")) -> ()
          }
          frame #1 {
            n1911 = local write "Stage Moving"(FALSE ("Stage Moving")) -> ()
            n1912 = case shown="True" w7640 {
              tunnel: w7641 -> [w7647 w7653]
              tunnel: w7642 -> [w7648 w7652]
              tunnel: [w7648 w7650] -> _
              tunnel: [w7647 w7649] -> _
              frame #0 {
              }
              frame #1 {
                n1913 = Concatenate Strings("stop" ("string"), "\r") -> (w7654:string)
                n1914 = VISA Write(VISA resource name=w7652, write buffer=w7654, error in (no error)=w7653) -> (VISA resource name out=w7650:refnum<visa-resource-name>, error out=w7649:errorcluster)  [unwired: 1 out]
              }
            }
            n1915 = case shown="True" TRUE {
              tunnel: "Cap 1 T ON" -> [w7657 w7658]
              frame #0 {
                n1916 = property on="Trap 1 (ON/OFF)" class="Bool (strict)"("Val(Sgnl)"=w7657) -> ()  [unwired: 2 in, 2 out]
              }
              frame #1 {
                n1917 = property on="Trap 2 (ON/OFF)" class="Bool (strict)"("Val(Sgnl)"=w7658) -> ()  [unwired: 2 in, 2 out]
              }
            }
            n1918 = call <vilib>:"Beep.vi"() -> ()  [unwired: 3 in, 9 out]
            n1919 = case shown="True" "Cap 1 Flow ON" {
              frame #0 {
              }
              frame #1 {
                n1920 = property on="Inject Pump 1" class="Bool (strict)"("Val(Sgnl)"=TRUE ("Value (Signaling)")) -> ()  [unwired: 2 in, 2 out]
              }
            }
          }
        }
      }
      event #3 {
        n1921 = event-data() -> ()  [unwired: 1 in, 5 out]
        n1922 = local write "Move Cap. 2 (ADig Left)"(FALSE ("Move Cap. 2 (ADig Left)")) -> ()
        n1923 = flat-sequence {
          tunnel: w7666 -> [w7674]
          tunnel: w7665 -> [w7673]
          tunnel: w7663 -> [w7672]
          tunnel: w7662 -> [w7671]
          tunnel: [w7670] -> w7661
          tunnel: [w7669] -> w7660
          tunnel: ["Cap 2 Samp Flow ON"] -> w7659
          tunnel: w7661 -> [w7697]
          tunnel: w7660 -> [w7696]
          tunnel: w7659 -> [w7695]
          frame #0 {
            n1924 = local read "Saved Stage Positions"() -> (w7684:dbl[][])
            n1925 = case shown="True" "Cap 2 Samp Flow ON" {
              tunnel: w7672 -> [w7686 w7692]
              tunnel: w7671 -> [w7687 w7691]
              tunnel: [w7687 w7689] -> w7670
              tunnel: [w7686 w7688] -> w7669
              frame #0 {
              }
              frame #1 {
                # "run flow"
                n1926 = Concatenate Strings("run" ("string"), "\r") -> (w7693:string)
                n1927 = VISA Write(VISA resource name=w7691, write buffer=w7693, error in (no error)=w7692) -> (VISA resource name out=w7689:refnum<visa-resource-name>, error out=w7688:errorcluster)  [unwired: 1 out]
              }
            }
            n1928 = Array Subset(array=w7684, index (row)=1 ("index"), length (row)=1 ("length"), index (col)=1 ("index"), length (col)=3 ("length")) -> (w7681:dbl[][])
            n1929 = Reshape Array(w7681, 3 ("dimension size")) -> (w7679:dbl[])
            n1930 = Array To Cluster(array=w7679) -> (cluster=w7678:cluster{"[0]":dbl, "[1]":dbl, "[2]":dbl})
            n1931 = call "Set Stage Position.vi"("Position"=w7678, "error in"=w7673, "VISA resource name in"=w7674) -> ("error out"=w7677:errorcluster)  [unwired: 2 out]
            n1932 = local write "Stage Moving"(TRUE ("Stage Moving")) -> ()
            n1933 = local write "Stage Control Serial Error"(w7677) -> ()
          }
          frame #1 {
            n1934 = local write "Stage Moving"(FALSE ("Stage Moving")) -> ()
            n1935 = case shown="True" TRUE {
              tunnel: "Cap 2 T ON" -> [w7708 w7709]
              frame #0 {
                n1936 = property on="Trap 2 (ON/OFF)" class="Bool (strict)"("Val(Sgnl)"=w7708) -> ()  [unwired: 2 in, 2 out]
              }
              frame #1 {
                n1937 = property on="Trap 1 (ON/OFF)" class="Bool (strict)"("Val(Sgnl)"=w7709) -> ()  [unwired: 2 in, 2 out]
              }
            }
            n1938 = call <vilib>:"Beep.vi"() -> ()  [unwired: 3 in, 9 out]
            n1939 = case shown="True" w7695 {
              tunnel: w7697 -> [_ w7703]
              tunnel: w7696 -> [_ w7702]
              frame #0 {
              }
              frame #1 {
                n1940 = Concatenate Strings("stop" ("string"), "\r") -> (w7705:string)
                n1941 = VISA Write(VISA resource name=w7703, write buffer=w7705, error in (no error)=w7702) -> ()  [unwired: 3 out]
              }
            }
            n1942 = case shown="True" "Cap 2 Flow ON" {
              frame #0 {
              }
              frame #1 {
                n1943 = property on="Inject Pump 3" class="Bool (strict)"("Val(Sgnl)"=TRUE ("Value (Signaling)")) -> ()  [unwired: 2 in, 2 out]
              }
            }
          }
        }
      }
      event #4 {
        n1944 = event-data() -> ()  [unwired: 1 in, 5 out]
        n1945 = flat-sequence {
          tunnel: w7710 -> [w7732]
          tunnel: w7711 -> [w7712]
          frame #0 {
            n1946 = call "Read Stage Position.vi"("error in"=w7732, "VISA resource name in"=w7712) -> ("Current Position"=w7717:cluster{dbl, dbl, dbl}, "error out"=w7730:errorcluster, "VISA resource name out"=w7731:refnum<visa-resource-name>)  [unwired: 1 out]
            n1947 = local read "Saved Stage Positions"() -> (w7741:dbl[][])
            n1948 = Divide(x="z nudge increment (um)", y=1000.0) -> (x/y=w7729:dbl)
            n1949 = Boolean To (0,1)(Boolean="+z") -> (0, 1=w7721:i16)
            n1950 = Boolean To (0,1)(Boolean="-z") -> (0, 1=w7722:i16)
            n1951 = Array Subset(array=w7741, index (row)=1 ("index"), length (row)=1 ("length"), index (col)=1 ("index"), length (col)=3 ("length")) -> (w7738:dbl[][])
            n1952 = Multiply(x=w7721, y=w7729) -> (x*y=w7725:dbl)
            n1953 = Multiply(x=w7722, y=w7729) -> (x*y=w7723:dbl)
            n1954 = Unbundle(w7717) -> (w7715:dbl, w7714:dbl, w7718:dbl)
            n1955 = Negate(x=w7723) -> (-x=w7724:dbl)
            n1956 = Reshape Array(w7738, 3 ("dimension size")) -> (w7736:dbl[])
            n1957 = Add(x=w7725, y=w7724) -> (x+y=w7726:dbl)
            n1958 = Array To Cluster(array=w7736) -> ()  [unwired: 1 out]
            n1959 = Add(x=w7726, y=w7718) -> (x+y=w7716:dbl)
            n1960 = Bundle(cluster=w7717, w7715, w7714, w7716) -> (w7713:cluster{dbl, dbl, dbl})
            n1961 = call "Set Stage Position.vi"("Position"=w7713, "error in"=w7730, "VISA resource name in"=w7731) -> ("error out"=w7735:errorcluster)  [unwired: 2 out]
            n1962 = local write "Stage Moving"(TRUE ("Stage Moving")) -> ()
            n1963 = local write "Stage Control Serial Error"(w7735) -> ()
          }
          frame #1 {
            n1964 = local write "Stage Moving"(FALSE ("Stage Moving")) -> ()
            n1965 = call <vilib>:"Beep.vi"() -> ()  [unwired: 3 in, 9 out]
          }
        }
      }
      event #5 {
        n1966 = event-data() -> ()  [unwired: 1 in, 5 out]
        n1967 = flat-sequence {
          tunnel: w7747 -> [w7750]
          tunnel: w7746 -> [w7749]
          tunnel: ["Cal @ (MHz)"] -> w7745
          tunnel: w7745 -> [w7770]
          frame #0 {
            n1968 = local read "Saved Stage Positions"() -> (w7753:dbl[][])
            n1969 = Array Subset(array=w7753, index (row)=2 ("index"), length (row)=1 ("length"), index (col)=1 ("index"), length (col)=3 ("length")) -> (w7756:dbl[][])
            n1970 = Reshape Array(w7756, 3 ("dimension size")) -> (w7758:dbl[])
            n1971 = local write "Stage Moving"(TRUE ("Stage Moving")) -> ()
            n1972 = Array To Cluster(array=w7758) -> (cluster=w7759:cluster{"[0]":dbl, "[1]":dbl, "[2]":dbl})
            n1973 = call "Set Stage Position.vi"("Position"=w7759, "error in"=w7749, "VISA resource name in"=w7750) -> ("error out"=w7760:errorcluster)  [unwired: 2 out]
            n1974 = local write "Stage Control Serial Error"(w7760) -> ()
          }
          frame #1 {
            n1975 = property on="Trap Delta (MHz)" class="DigNum (strict)"("Val(Sgnl)"="Cal @ (MHz)") -> ()  [unwired: 2 in, 2 out]
            n1976 = local write "Stage Moving"(FALSE ("Stage Moving")) -> ()
            n1977 = call <vilib>:"Beep.vi"() -> ()  [unwired: 3 in, 9 out]
          }
          frame #2 {
            n1978 = Wait (ms)(milliseconds to wait=u32 500) -> ()  [unwired: 1 out]
          }
          frame #3 {
            n1979 = property on="Save Calibration" class="Bool (strict)"("Val(Sgnl)"=TRUE ("Value (Signaling)")) -> ()  [unwired: 2 in, 2 out]
          }
          frame #4 {
            n1980 = Wait (ms)(milliseconds to wait=u32 4000) -> ()  [unwired: 1 out]
          }
          frame #5 {
            n1981 = while {
              stop <- w7767 stop-if-true
              n1982 = local read "Saving..."() -> (w7768:bool)
              n1983 = Wait (ms)(milliseconds to wait=u32 500) -> ()  [unwired: 1 out]
              n1984 = Not(x=w7768) -> (.not. x?=w7767:bool)
            }
          }
          frame #6 {
            n1985 = case shown="True" "W/ Offset" {
              tunnel: w7770 -> [_ w7775]
              frame #0 {
                n1986 = Multiply(x="Cal read wait (s)", y=u32 1000 ("milliseconds to wait")) -> (x*y=w7773:u32)
                n1987 = Wait (ms)(milliseconds to wait=w7773) -> ()  [unwired: 1 out]
              }
              frame #1 {
                n1988 = flat-sequence {
                  tunnel: w7775 -> [w7783]
                  frame #0 {
                    n1989 = property on="Trap Delta (MHz)" class="DigNum (strict)"("Val(Sgnl)"="Offset @ (MHz)") -> ()  [unwired: 2 in, 2 out]
                  }
                  frame #1 {
                    n1990 = Wait (ms)(milliseconds to wait=u32 500) -> ()  [unwired: 1 out]
                  }
                  frame #2 {
                    n1991 = property on="Trap Raster Scan" class="Bool (strict)"("Val(Sgnl)"=TRUE ("Value (Signaling)")) -> ()  [unwired: 2 in, 2 out]
                  }
                  frame #3 {
                    n1992 = Wait (ms)(milliseconds to wait=u32 2000) -> ()  [unwired: 1 out]
                  }
                  frame #4 {
                    n1993 = while {
                      stop <- w7781 stop-if-true
                      n1994 = local read "Raster Scanning..."() -> (w7782:bool)
                      n1995 = Wait (ms)(milliseconds to wait=u32 500) -> ()  [unwired: 1 out]
                      n1996 = Not(x=w7782) -> (.not. x?=w7781:bool)
                    }
                  }
                  frame #5 {
                    n1997 = property on="Trap Delta (MHz)" class="DigNum (strict)"("Val(Sgnl)"=w7783) -> ()  [unwired: 2 in, 2 out]
                  }
                }
              }
            }
          }
          frame #7 {
            n1998 = property on="Read Cal" class="Bool (strict)"("Val(Sgnl)"=TRUE ("Value (Signaling)")) -> ()  [unwired: 2 in, 2 out]
          }
          frame #8 {
            n1999 = Wait (ms)(milliseconds to wait=u32 500) -> ()  [unwired: 1 out]
          }
          frame #9 {
            n2000 = property on="Fish for Tether" class="Bool (strict)"("Val(Sgnl)"=TRUE ("Value (Signaling)")) -> ()  [unwired: 2 in, 2 out]
          }
        }
        n2001 = local write "Cal/Data Acq. Spot"(FALSE ("Cal/Data Acq. Spot")) -> ()
      }
      event #6 {
        n2002 = event-data() -> ()  [unwired: 1 in, 5 out]
        n2003 = flat-sequence {
          tunnel: w7788 -> [w7794]
          tunnel: w7787 -> [w7793]
          frame #0 {
            w7790 = FALSE ("Fl. Triggered...")
            n2004 = local read "Saving..."() -> (w7791:bool)
            n2005 = local write "Fl. Triggered..."(w7790) -> ()
            n2006 = local write "Stage Moving"(TRUE ("Stage Moving")) -> ()
            n2007 = property on="Green Laser ON/Interlacing" class="Bool (strict)"("Val(Sgnl)"=w7790) -> ()  [unwired: 2 in, 2 out]
            n2008 = local write "Stop Saving"(w7791) -> ()
          }
          frame #1 {
            n2009 = local read "Saved Stage Positions"() -> (w7795:dbl[][])
            n2010 = Array Subset(array=w7795, index (row)=3 ("index"), length (row)=1 ("length"), index (col)=1 ("index"), length (col)=3 ("length")) -> (w7800:dbl[][])
            n2011 = Reshape Array(w7800, 3 ("dimension size")) -> (w7798:dbl[])
            n2012 = Array To Cluster(array=w7798) -> (cluster=w7797:cluster{"[0]":dbl, "[1]":dbl, "[2]":dbl})
            n2013 = call "Set Stage Position.vi"("Position"=w7797, "error in"=w7793, "VISA resource name in"=w7794) -> ()  [unwired: 3 out]
          }
          frame #2 {
            w7804 = FALSE ("Value (Signaling)")
            n2014 = property on="Trap 1 (ON/OFF)" class="Bool (strict)"("Val(Sgnl)"=w7804) -> ()  [unwired: 2 in, 2 out]
            n2015 = property on="Trap 2 (ON/OFF)" class="Bool (strict)"("Val(Sgnl)"=w7804) -> ()  [unwired: 2 in, 2 out]
            n2016 = call <vilib>:"Beep.vi"() -> ()  [unwired: 3 in, 9 out]
          }
          frame #3 {
            n2017 = property on="Move Cap. 2 (ADig Left)" class="Bool (strict)"("Val(Sgnl)"=TRUE ("Value (Signaling)")) -> ()  [unwired: 2 in, 2 out]
          }
        }
      }
      event #7 {
        n2018 = event-data() -> ()  [unwired: 1 in, 5 out]
        n2019 = flat-sequence {
          tunnel: w7812 -> [w7816]
          tunnel: w7813 -> [w7817]
          tunnel: [w7817] -> w7807
          tunnel: [w7816] -> w7806
          tunnel: [w7820] -> w7810
          tunnel: [w7819] -> w7808
          tunnel: w7807 -> [w7823]
          tunnel: w7806 -> [w7822]
          tunnel: [w7833] -> w7811
          tunnel: w7810 -> [w7833]
          tunnel: [w7832] -> w7809
          tunnel: w7808 -> [w7832]
          tunnel: w7811 -> [w7838]
          tunnel: w7809 -> [w7837]
          frame #0 {
            n2020 = case shown="True" "Move Trap Before?" {
              frame #0 {
              }
              frame #1 {
                n2021 = property on="Trap Delta (MHz)" class="DigNum (strict)"("Val(Sgnl)"="Dip Trap Delta 1 (MHz)") -> ()  [unwired: 2 in, 2 out]
              }
            }
          }
          frame #1 {
            n2022 = local read "Saved Stage Positions"() -> (w7821:dbl[][])
            n2023 = Array Subset(array=w7821, index (row)=4 ("index"), length (row)=1 ("length"), index (col)=1 ("index"), length (col)=3 ("length")) -> (w7828:dbl[][])
            n2024 = Reshape Array(w7828, 3 ("dimension size")) -> (w7826:dbl[])
            n2025 = Array To Cluster(array=w7826) -> (cluster=w7825:cluster{"[0]":dbl, "[1]":dbl, "[2]":dbl})
            n2026 = call "Set Stage Position.vi"("Position"=w7825, "error in"=w7822, "VISA resource name in"=w7823) -> ("error out"=w7819:errorcluster, "VISA resource name out"=w7820:refnum<visa-resource-name>)  [unwired: 1 out]
          }
          frame #2 {
            n2027 = Multiply(x="Duration (s)", y=1000.0) -> (x*y=w7834:dbl)
            n2028 = Wait (ms)(milliseconds to wait=w7834) -> ()  [unwired: 1 out]
          }
          frame #3 {
            n2029 = local read "Saved Stage Positions"() -> (w7839:dbl[][])
            n2030 = Array Subset(array=w7839, index (row)=2 ("index"), length (row)=1 ("length"), index (col)=1 ("index"), length (col)=3 ("length")) -> (w7844:dbl[][])
            n2031 = Reshape Array(w7844, 3 ("dimension size")) -> (w7842:dbl[])
            n2032 = Array To Cluster(array=w7842) -> (cluster=w7841:cluster{"[0]":dbl, "[1]":dbl, "[2]":dbl})
            n2033 = call "Set Stage Position.vi"("Position"=w7841, "error in"=w7837, "VISA resource name in"=w7838) -> ()  [unwired: 3 out]
          }
          frame #4 {
            n2034 = case shown="True" "Move Trap After?" {
              frame #0 {
              }
              frame #1 {
                n2035 = property on="Trap Delta (MHz)" class="DigNum (strict)"("Val(Sgnl)"="Dip Trap Delta 2 (MHz)") -> ()  [unwired: 2 in, 2 out]
              }
            }
          }
          frame #5 {
            n2036 = case shown="True" "Green ON After?" {
              frame #0 {
              }
              frame #1 {
                n2037 = property on="Green Laser ON/Interlacing" class="Bool (strict)"("Val(Sgnl)"=TRUE ("Value (Signaling)")) -> ()  [unwired: 2 in, 2 out]
              }
            }
          }
          frame #6 {
            n2038 = Wait (ms)(milliseconds to wait=u32 500) -> ()  [unwired: 1 out]
          }
          frame #7 {
            n2039 = case shown="True" "Save Data After?" {
              frame #0 {
              }
              frame #1 {
                n2040 = property on="Start Saving" class="Bool (strict)"("Val(Sgnl)"=TRUE ("Value (Signaling)")) -> ()  [unwired: 2 in, 2 out]
              }
            }
          }
        }
      }
      event #8 {
        n2041 = event-data() -> ()  [unwired: 1 in, 5 out]
        n2042 = flat-sequence {
          tunnel: w7863 -> [w7866]
          tunnel: w7862 -> [w7874]
          tunnel: [w7868] -> w7861
          tunnel: [w7867] -> w7860
          tunnel: [w7865] -> w7858
          tunnel: [w7864] -> w7855
          tunnel: w7861 -> [w7881]
          tunnel: w7860 -> [w7880]
          tunnel: [w7878] -> w7859
          tunnel: w7858 -> [w7879]
          tunnel: [w7877] -> w7857
          tunnel: [w7876] -> w7856
          tunnel: w7855 -> [w7876]
          tunnel: w7859 -> [w7885]
          tunnel: w7857 -> [w7884]
          tunnel: w7856 -> [w7883]
          frame #0 {
            n2043 = call "Read Stage Position.vi"("error in"=w7874, "VISA resource name in"=w7866) -> ("Current Position"=w7864:cluster{dbl, dbl, dbl}, "error out"=w7867:errorcluster, "VISA resource name out"=w7865:refnum<visa-resource-name>)  [unwired: 1 out]
            "Current Position" <- w7864
            n2044 = local write "Stage Control Serial Error"(w7867) -> ()
            n2045 = Unbundle(w7864) -> (w7871:dbl, w7873:dbl, w7869:dbl)
            n2046 = Add(x=w7873, y="Y change (mm)") -> (x+y=w7870:dbl)
            n2047 = Bundle(w7871, w7870, w7869) -> (w7868:cluster{dbl, dbl, dbl})  [unwired: 1 in]
          }
          frame #1 {
            # "move to new position and start saving"
            n2048 = local write "Stage Moving"(TRUE ("Stage Moving")) -> ()
            n2049 = local write "Start Saving"(TRUE ("Start Saving")) -> ()
            n2050 = call "Set Stage Position.vi"("Position"=w7881, "error in"=w7880, "VISA resource name in"=w7879) -> ("error out"=w7877:errorcluster, "VISA resource name out"=w7878:refnum<visa-resource-name>)  [unwired: 1 out]
          }
          frame #2 {
            # "go back to start"
            n2051 = call "Set Stage Position.vi"("Position"=w7883, "error in"=w7884, "VISA resource name in"=w7885) -> ()  [unwired: 3 out]
          }
          frame #3 {
            # "stop saving"
            n2052 = local write "Stop Saving"(TRUE ("Stop Saving")) -> ()
            n2053 = local write "Stage Moving"(FALSE ("Stage Moving")) -> ()
          }
        }
      }
      event #9 {
        n2054 = event-data() -> ()  [unwired: 1 in, 5 out]
        n2055 = Or(x="Move to Position 5", y="Lower Ch. Cap.") -> (x .or. y?=w7891:bool)
        n2056 = Build Array("Move to Position 1", "Move to Position 2", "Move to Position 3", "Move to Position 4", w7891) -> (w7894:bool[])
        n2057 = Boolean Array To Number(Boolean array=w7894) -> (number=w7893:u32)
        n2058 = Logarithm Base 2(1:w7893) -> (0:w7892:dbl)
        n2059 = flat-sequence {
          tunnel: w7892 -> [w7903]
          tunnel: w7889 -> [w7901]
          tunnel: w7888 -> [w7900]
          frame #0 {
            n2060 = local read "Saved Stage Positions"() -> (w7911:dbl[][])
            n2061 = Array Subset(array=w7911, index (row)=w7903, length (row)=1 ("length"), index (col)=1 ("index"), length (col)=3 ("length")) -> (w7908:dbl[][])
            n2062 = Reshape Array(w7908, 3 ("dimension size")) -> (w7906:dbl[])
            n2063 = Array To Cluster(array=w7906) -> (cluster=w7905:cluster{"[0]":dbl, "[1]":dbl, "[2]":dbl})
            n2064 = call "Set Stage Position.vi"("Position"=w7905, "error in"=w7900, "VISA resource name in"=w7901) -> ("error out"=w7904:errorcluster)  [unwired: 2 out]
            n2065 = local write "Stage Moving"(TRUE ("Stage Moving")) -> ()
            n2066 = local write "Stage Control Serial Error"(w7904) -> ()
          }
          frame #1 {
            n2067 = call <vilib>:"Beep.vi"() -> ()  [unwired: 3 in, 9 out]
            n2068 = local write "Stage Moving"(FALSE ("Stage Moving")) -> ()
          }
        }
      }
      event #10 {
        n2069 = event-data() -> ()  [unwired: 1 in, 5 out]
        n2070 = property on="Move Cap. 1 (DNA Right)" class="Bool (strict)"("Val(Sgnl)"=TRUE ("Value (Signaling)")) -> ()  [unwired: 2 in, 2 out]
        n2071 = property on="Inject Pump 3" class="Bool (strict)"("Val(Sgnl)"=FALSE ("Value (Signaling)")) -> ()  [unwired: 2 in, 2 out]
      }
      event #11 {
        n2072 = event-data() -> ()  [unwired: 1 in, 5 out]
        n2073 = property on="Cal/Data Acq. Spot" class="Bool (strict)"("Val(Sgnl)"=TRUE ("Value (Signaling)")) -> ()  [unwired: 2 in, 2 out]
        n2074 = property on="Inject Pump 1" class="Bool (strict)"("Val(Sgnl)"=FALSE ("Value (Signaling)")) -> ()  [unwired: 2 in, 2 out]
      }
      event #12 {
        n2075 = event-data() -> ()  [unwired: 1 in, 5 out]
        n2076 = flat-sequence {
          tunnel: [w7945] -> w7935
          tunnel: [w7944] -> w7928
          tunnel: [w7943] -> w7920
          tunnel: [w7948] -> w7936
          tunnel: w7935 -> [w7948]
          tunnel: [w7947] -> w7929
          tunnel: w7928 -> [w7947]
          tunnel: [w7946] -> w7921
          tunnel: w7920 -> [w7946]
          tunnel: [w7952] -> w7937
          tunnel: w7936 -> [w7952]
          tunnel: [w7951] -> w7930
          tunnel: w7929 -> [w7951]
          tunnel: [w7950] -> w7922
          tunnel: w7921 -> [w7950]
          tunnel: [w7958] -> w7938
          tunnel: w7937 -> [w7958]
          tunnel: [w7957] -> w7931
          tunnel: w7930 -> [w7957]
          tunnel: [w7956] -> w7923
          tunnel: w7922 -> [w7956]
          tunnel: [w7962] -> w7939
          tunnel: w7938 -> [w7962]
          tunnel: [w7961] -> w7932
          tunnel: w7931 -> [w7961]
          tunnel: [w7960] -> w7924
          tunnel: w7923 -> [w7960]
          tunnel: [w7966] -> w7940
          tunnel: w7939 -> [w7966]
          tunnel: [w7965] -> w7933
          tunnel: w7932 -> [w7965]
          tunnel: [w7964] -> w7925
          tunnel: w7924 -> [w7964]
          tunnel: [w7970] -> w7941
          tunnel: w7940 -> [w7970]
          tunnel: [w7969] -> w7934
          tunnel: w7933 -> [w7969]
          tunnel: [w7968] -> w7926
          tunnel: w7925 -> [w7968]
          tunnel: w7941 -> [w7976]
          tunnel: w7934 -> [w7975]
          tunnel: [w7973] -> w7927
          tunnel: w7926 -> [w7973]
          tunnel: w7927 -> [w7977]
          frame #0 {
            n2077 = local read "Green Laser ON/Interlacing"() -> (w7945:bool)
            n2078 = local read "Green laser mode"() -> (w7944:enum32{"Laser ON", "Laser OFF", "Interlace"})
            n2079 = local read "Green FB On/Off"() -> (w7943:bool)
          }
          frame #1 {
            n2080 = property on="Green FB On/Off" class="Bool (strict)"("Val(Sgnl)"=FALSE ("Value (Signaling)")) -> ()  [unwired: 2 in, 2 out]
          }
          frame #2 {
            n2081 = property on="Green Laser ON/Interlacing" class="Bool (strict)"("Val(Sgnl)"=TRUE ("Value (Signaling)")) -> ()  [unwired: 2 in, 2 out]
            n2082 = property on="Flip Green Filter" class="Bool (strict)"("Val(Sgnl)"=TRUE ("Value (Signaling)")) -> ()  [unwired: 2 in, 2 out]
            n2083 = property on="Green laser mode" class="RadioBtnsControl (strict)"("Val(Sgnl)"=enum32{"Laser ON", "Laser OFF", "Interlace"}."Laser ON" ("Value (Signaling)")) -> ()  [unwired: 2 in, 2 out]
          }
          frame #3 {
            n2084 = Wait (ms)(milliseconds to wait=u32 500) -> ()  [unwired: 1 out]
          }
          frame #4 {
            n2085 = property on="Confocal Image" class="Bool (strict)"("Val(Sgnl)"=TRUE ("Value (Signaling)")) -> ()  [unwired: 2 in, 2 out]
          }
          frame #5 {
            n2086 = Wait (ms)(milliseconds to wait=u32 2000) -> ()  [unwired: 1 out]
          }
          frame #6 {
            n2087 = while {
              stop <- w7971 stop-if-true
              n2088 = local read "Saving..."() -> (w7972:bool)
              n2089 = Not(x=w7972) -> (.not. x?=w7971:bool)
            }
          }
          frame #7 {
            n2090 = property on="Flip Green Filter" class="Bool (strict)"("Val(Sgnl)"=TRUE ("Value (Signaling)")) -> ()  [unwired: 2 in, 2 out]
            n2091 = property on="Green Laser ON/Interlacing" class="Bool (strict)"("Val(Sgnl)"=w7976) -> ()  [unwired: 2 in, 2 out]
            n2092 = property on="Green laser mode" class="RadioBtnsControl (strict)"("Val(Sgnl)"=w7975) -> ()  [unwired: 2 in, 2 out]
          }
          frame #8 {
            n2093 = property on="Green FB On/Off" class="Bool (strict)"("Val(Sgnl)"=w7977) -> ()  [unwired: 2 in, 2 out]
          }
        }
      }
      event #13 {
        n2094 = event-data() -> ()  [unwired: 1 in, 5 out]
        n2095 = local read "Stop All"() -> (w7978:bool)
      }
    }
    n2096 = node-c288() -> ()  [unwired: 1 in, 1 out]
  }
  n2097 = node-c288(w30) -> ()  [unwired: 1 out]
  n2098 = node-c288(w32) -> ()  [unwired: 1 out]
  n2099 = node-c288(w17) -> ()  [unwired: 1 out]
  n2100 = VISA Close(VISA resource name=w21, error in (no error)=w20) -> (error out=w74:errorcluster)
  n2101 = call <vilib>:"Simple Error Handler.vi"("error in (no error)"=w74) -> ()  [unwired: 1 in, 8 out]
  n2102 = node-c288(w28) -> ()  [unwired: 1 out]
  n2103 = node-c288(w138) -> ()  [unwired: 1 out]
  n2104 = flat-sequence {
    tunnel: w237 -> [w7982]
    tunnel: w239 -> [w7983]
    tunnel: [w7981] -> w217
    tunnel: [w7980] -> w216
    tunnel: w195 -> [_]
    tunnel: w193 -> [_]
    tunnel: w146 -> [_]
    tunnel: w34 -> [_]
    tunnel: w217 -> [w8041]
    tunnel: w216 -> [w8042]
    frame #0 {
      w7979 = FALSE ("AI to FIFO")
      n2105 = xnode "Read/Write Control"("FPGA VI Reference In"=w7983, "error in"=w7982, "AI to FIFO"=w7979, "APD to FIFO"=w7979) -> ("FPGA VI Reference Out"=w7981:T15, "error out"=w7980:errorcluster)
    }
    frame #1 {
      n2106 = xnode "Close FPGA VI Reference"("FPGA VI Reference In"=w8041, "error in"=w8042) -> ("error out"=→"error out":errorcluster)
    }
  }
